vi "EPR DAQ - 1.2.5.13.vi"() -> ()   [LabVIEW 2016]
uses:
  Types/State Control.ctl
  Types/Fitting Model Selection.ctl
  Types/Acquisition Parameters.ctl
  Types/Hardware Parameters.ctl
  Types/Measurement Information.ctl
  Analysis/Dose Calculation and Reporting/Dose Calculation Control.ctl
  Types/Sample Type.ctl
  Types/Spectral Data.ctl
  Types/Save Data Type.ctl
  Types/Global Variables.vi
  DAQ Management/Write Key Bool.vi
  DAQ Management/Get Key U32.vi
panel:
  out "In-Phase SNR":dbl
  in  "Flag Bad Set":bool
  out "Previous Scan range (Gauss)":dbl=25.0 min=0.001 max=55.0 format="%.3f"
  out "Previous Mod. Amp. (Gauss)":dbl=4.0 min=0.0 max=4.0 format="%.4f"
  in  "Acquisition Updates Prescribe":bool
  in  "Single Test Scan":bool
  out "Unacceptable pO2 Estimate":bool
  in  "Exclude Unacceptable pO2":bool
  out "Number of Fit Iterations":i32 caption="Iterations"
  out "SpO2 [%]":dbl format="%#.0f"
  in  "SpO2 Calibration [SpO2/V]":dbl
  in  "Acquire SpO2":bool
  out "pO2 [mmHg]":dbl[](array[numeric]) format="%.1f"
  in  "AFC Field Correction":bool
  in  "Report pO2/Scan":bool
  in  "Open Session Data Folder":bool
  in  "Show Variable Window?":bool
  out "Script Progress":dbl(slide) scale=0.0..1.0
  out "Set Progress":dbl(slide) scale=0.0..1.0
  in  "Sweep Rise [sec]":u32=3
  in  "Prescan delay (ms)":u32=750
  in  "Scan time (sec)":dbl=3.0 format="%.2f"
  in  "Find Peaks":bool
  in  "Continuous Sweeping":bool
  in  "Show Calibration Constants":bool
  in  "Gradients on/off":bool
  in  "Z-Gradient [G/mm]":dbl min=0.0
  in  "Y-Gradient [G/mm]":dbl min=0.0
  in  "X-Gradient [G/mm]":dbl min=0.0
  in  "Spectral Data":T1={"PDT Amp [v]"=0.0, "RIS Amp [v]"=0.0, "B-Field"=[], "All In-Phase Scan Spectra"=[], "Model Select"=enum."OneCompRISTwoPDT", "Fit Each Scan"=FALSE, "PDT Center [g]"=0.0, "In-Phase Average Spectra"=[], "In-Phase Median Spectra"=[], "Out-Phase Median Spectra"=[], "Out-Phase Average Spectra"=[], "Fit Spectra"=[], "Fit No-Baseline Spectra"=[], "All Out-Phase Scan Spectra"=[], "Baseline Offset Correction"=FALSE, "In-Phase Offset [v]"=0.0, "Out-Phase Offset [v]"=0.0, "Ch2 Input\n(Balance)"=[], "Ch3 Input\n(Phase)"=[], "Ch4 Input\n(AFC)"=[], "Fit Pars"=[], "Fit Pars Errors"=[], "Fit Pars Labels"=[], "Raw Scan DAQ Data"=[], "Bad Scans Indicies"=[], "Good In-Phase Scan Spectra"=[], "Good Out-Phase Scan Spectra"=[], "Bad In-Phase Scan Spectra"=[], "Bad Out-Phase Scan Spectra"=[], "Number of bad scans"=0, "Fit History"=[], "PDT Amp. History/Set [v]"=[], "RIS Amp. History/Set [v]"=[], "RIS Amp. History/Scan [v]"=[], "All Shifted B-Fields"=[], "Good Shifted B-Fields"=[], "Ch5 Input\n(SpO2)"=[], "Ch6 Input\n(BPM)"=[], "Global SNR"=0.0, "Fit Error History"=[], "SNR History"=[]} {"Global SNR" min=0.0; "PDT Center [g]" min=0.0; "RIS Amp [v]" min=0.0; "PDT Amp [v]" min=0.0}
  in  "Measurement Information":T3={"Comments"="", "Directory Input"="", "Data file path"=path "C:/Data/EPR Data", "Scripting File"=path "C:/Data/Configuration Script.csv", "Save Data"=FALSE, "Tooth size (d11) [mm]"=0.0, "Tooth size (d12) [mm]"=0.0, "Tooth size (d21) [mm]"=0.0, "Tooth size (d22) [mm]"=0.0, "Dose of Tooth [Gy]"=0.0, "Safe Shutdown?"=FALSE, "Gases Available"=[], "Database Username"="", "Database Password"="", "Database Login URL"="", "Database Upload URL"="", "Database Success URL"="", "Database XML URL"="", "Database Resonator URL"="", "Session Number"=0, "Set #"=0, "Resonator Operator"="", "Session Type"="", "Tooth/Sample ID"="", "Volunteer ID"="", "Computer Operator"="", "Volunteer Type"="", "Site/Tooth Selection (T8,T9)"="", "Resonator"="", "Measurement Site"="", "Non-standard session?"=FALSE, "EPR DAQ Version"="", "Session Path"=path "C:/Data/EPR Data", "Chosen Applied State"="", "Chosen Initial State"="", "Time of Transition"="", "DAQ Mode"=enum."Engineering", "pO2/Scan [mmHg]"=[], "pO2/Set [mmHg]"=[], "Linewidth (HWHM)/Scan [Gauss]"=[], "Linewidth (HWHM)/Set [Gauss]"=[], "pO2 Conversion"="", "Dose Calibration Cluster"={"Dose Response"={"grand_mean"=0.0292016, "slope"=0.0188720543}, "Dose Correction"={"Sex"=1, "a0"=7.719669421, "a1"=-2.746550736, "a2"=-0.186490355, "a3"=0.041922063, "a4"=-0.849147359, "a5"=0.14330063, "a6"=0.019930219, "A_n"=40.0, "H_n"=10.12, "Dose Correction"=FALSE}, "Dose Reporting"={"Reporting is"=TRUE, "sd_threshold [AU]"=0.06, "sd_model [Gy]"=0.66, "dosimetric_threshold [Gy]"=2.0, "Add intrasession errors is"=FALSE, "Prior Radiation?"=FALSE}}, "OxyChip Slope"=0.0, "OxyChip Intercept"=0.0, "QA Mode"=enum."Select QA Mode", "QA Session?"=FALSE, "Sample Type"=enum."Empty Resonator", "Report pO2/Scan"=FALSE, "Skip End Session Save"=FALSE, "Number of sites"=enum."# Probes", "Recipient Name"="", "Sender Name"="", "Recipient Email"="", "Transition State History"=[], "pO2 Report Times"=[], "Temperature [C]"=0.0, "+Error pO2/Scan [mmHg]"=[], "-Error pO2/Scan [mmHg]"=[], "+Error pO2/Set [mmHg]"=[], "-Error pO2/Set [mmHg]"=[], "Oxy Phase Exclusion Tolerance [rad]"=0.0, "Oxy Center Exclusion Tolerance [%]"=0.0, "Oxy Exclude Unacceptable"=FALSE, "Oxy Unacceptable Estimate Flags"=[], "Save Session PPT"=FALSE, "Flagged Bad Sets"=[]} {"Oxy Center Exclusion Tolerance [%]" format="%#_9g"; "Oxy Phase Exclusion Tolerance [rad]" format="%#_9g"; "Temperature [C]" format="%#_9g"; "OxyChip Intercept" format="%#_9g"; "OxyChip Slope" format="%#_9g"; "Dose Calibration Cluster"."Dose Reporting"."dosimetric_threshold [Gy]" format="%#_9g"; "Dose Calibration Cluster"."Dose Reporting"."sd_model [Gy]" format="%#_9g"; "Dose Calibration Cluster"."Dose Reporting"."sd_threshold [AU]" format="%#_9g"; "Dose Calibration Cluster"."Dose Correction"."H_n" format="%#_9g"; "Dose Calibration Cluster"."Dose Correction"."A_n" format="%#_9g"; "Dose Calibration Cluster"."Dose Correction"."a6" format="%#.9g"; "Dose Calibration Cluster"."Dose Correction"."a5" format="%#.9g"; "Dose Calibration Cluster"."Dose Correction"."a4" format="%#.9g"; "Dose Calibration Cluster"."Dose Correction"."a3" format="%#.9g"; "Dose Calibration Cluster"."Dose Correction"."a2" format="%#.9g"; "Dose Calibration Cluster"."Dose Correction"."a1" format="%#.9g"; "Dose Calibration Cluster"."Dose Correction"."a0" format="%#.9g"; "Dose Calibration Cluster"."Dose Correction"."Sex" items=["Male"=1, "Female"=0]; "Dose Calibration Cluster"."Dose Response"."slope" format="%#_9g"; "Dose Calibration Cluster"."Dose Response"."grand_mean" format="%#_9g"}
  in  "Hardware Parameters":T6={"Scan Calibration [G/V]"=0.0, "Modulation Calibration [G/V]"=0.0, "Modulation Phase [deg]"=0.0, "Modulation Frequency [Hz]"=0.0, "Attenuation [dB]"=0, "Input Channel Count"=0, "Time constant"=7, "Sensitivity"=17, "Frequency Output Voltage [V]"=0.0, "Phase Output Voltage [V]"=0.0, "Lock-in Offset Compensation"=FALSE, "RF [GHz]"=0.0, "Q Start"=0.0, "Q End"=0.0, "Balance"=0.0, "Phase Error"=0.0, "AFC Error"=0.0, "AFC"=FALSE, "Magnet Rotation"=FALSE, "Balance Scaling Factor"=1.0, "Phase Error Scaling Factor"=1.0, "AFC Error Scaling Factor"=1.0, "Frequency Counter ID"="", "Sweep Waveform"=enum."Sawtooth", "Q-Factor Scale"=0.0, " Q-Data Scale"=0.0, " Q-Data Offset"=0.0, "Magnet Rotation Slope"=0.0, "Magnet Rotation Offset"=0.0, "Phase Sweep Resolution"=0.0, "Hardware Version Number"="", "Spectrometer ID Number"=0, "Spectrometer Name"="", "Lock in Saturation"=0.0, "Balance Threshold"=0.0, "Phase Error Threshold"=0.0, "AFC Error Threshold"=0.0, "Linear Actuator Length"=0.0, "Lock-in OK?"=FALSE, "Ignore Lock-in Comm. Failure"=FALSE, "Gradient Addresses"=[], "Gradient Calibrations [G/A*mm]"=[], "Gradient Power Supplies"=[], "Lock-in Address"="", "Magnet Type"=enum."RRI", "Camera Names"=[], "Sweep Limit [Gauss]"=0.0, "Modulation Limit [Gauss]"=0.0, "Balance Threshold Exceeded?"=FALSE, "Phase Threshold Exceeded?"=FALSE, "AFC Threshold Exceeded?"=FALSE, "Consecutive Re-tune attempts"=0, "Reverse Sweep Slope [sec]"=0.0, "Reverse Sweep Offset [G]"=0.0, "AFC Field Correction [V/MHz]"=0.0, "Active Gradients (X Y Z)"=[], "SpO2 Calibration [SpO2/V]"=1.0, "Heart Rate Calibration [BPM/V]"=1.0, "Thermocouple Channel"=""} {"Sensitivity" items=["", "2 nV", "5 nV", "10 nV", "20 nV", "50 nV", "100 nV", "200 nV", "500 nV", "1 uV", "2 uV", "5 uV", "10 uV", "20 uV", "50 uV", "100 uV", "200 uV", "500 uV", "1 mV", "2 mV", "5 mV", "10 mV", "20 mV", "50 mV", "100 mV", "200 mV", "500 mV", "1 V"]; "Time constant" items=["10 us", "20 us", "40 us", "80 us", "160 us", "320 us", "640 us", "5 ms", "10 ms", "20 ms", "50 ms", "100 ms", "200 ms", "500 ms", "1 s", "2 s", "5 s", "10 s", "20 s", "50 s", "100 s", "200 s", "500 s", "1 ks", "2 ks", "5 ks", "10 ks", "20 ks", "50 ks", "100 ks"]}
  in  "Acquisition Parameters":T7={"Magnet Angle [deg]"=0.0, "Magnet Angles [deg]"=[], "DeltaVpp [v]"=0.0, "SEM [v]"=0.0, "DeltaVpp Thresh [v]"=0.0, "SEM Thresh [v]"=0.0, "Adaptive Processing"=FALSE, "Acquire Q"=FALSE, "Acquire Photos"=FALSE, "Adaptive Tuning"=FALSE, "Automated Matching"=FALSE, "X-Gradient [G/mm]"=0.0, "Y-Gradient [G/mm]"=0.0, "Z-Gradient [G/mm]"=0.0, "Central Field [G]"=0.0, "Scan Width [G]"=0.0, "Mod. Amp. [G]"=0.0, "Scan Time [s]"=0.0, "Pre-Scan Delay [ms]"=0, "Measurement Timeout [s]"=0.0, "Electromagnet Main Field [G]"=0.0, "Locked Central Field [G]"=0.0, "Scans Excluded"=0, "Scans Completed"=0, "No. Scans/Set"=0, "No. Scans for SNR"=0, "Field Locked Frequency [GHz]"=0.0, "Auto Set-based Field Center"=FALSE, "Prompt for oxy acquisition updates"=FALSE, "Oxy QA Scan?"=FALSE, "Exclude Bad Data"=FALSE, "Optimizing RF Power"=FALSE, "Gradients on/off"=FALSE, "Running Script"=TRUE, "Opto-Coupler Current [A]"=0.0, "Continuous Sweeping"=FALSE, "Sweep Rise Time [sec]"=0, "Reverse Sweep Central Field [G]"=0.0, "Forward Sweep Central Field [G]"=0.0, "Sweep Calibrated"=FALSE, "Modulation Calibrated"=FALSE, "First CheckCal Scan?"=FALSE, "AFC Field Correction"=FALSE, "OxyQAInit Scan Width [G]"=0.0, "OxyQAInit Mod. Amp. [G]"=0.0, "Scans Completed/Session"=0, "Acquire SpO2"=FALSE, "Acquire Temperature"=FALSE, "Over Mod"=FALSE} {"OxyQAInit Mod. Amp. [G]" min=0.0; "OxyQAInit Scan Width [G]" min=0.0; "Mod. Amp. [G]" min=0.0; "Scan Width [G]" min=0.0; "Measurement Timeout [s]" min=0.0; "Scan Time [s]" min=0.0; "Z-Gradient [G/mm]" min=0.0; "Y-Gradient [G/mm]" min=0.0; "X-Gradient [G/mm]" min=0.0; "SEM Thresh [v]" min=0.0; "DeltaVpp Thresh [v]" min=0.0; "SEM [v]" min=0.0}
  in  "Update Scan/Mod from Cursors":bool
  in  "Model Select":T2=enum."OneCompRISTwoPDT"
  in  "Refit Spectra":bool
  in  "Fit Each Scan":bool=TRUE
  in  "DAQ Mode":enum16{"Engineering", "Dosimetry", "Oximetry"}(ring)
  out "Out-Phase Noise":dbl
  out "In-Phase Noise":dbl
  out "Fit Pars and Labels":cluster{"Pars Labels":string[], "pars":dbl[]}
  in  "Timer on/off":bool
  out "Time Remaining":dbl caption="Elapsed Time (s)" format="%<%H:%M:%S>t"
  in  "Timer Value":dbl=600.0 caption="Time Target (s)" min=1.0 format="%<%H:%M:%S>t"
  in  "Optimize RF Power":bool
  in  "Apply & Lock Center Field":bool
  in  "Update Center Field":bool
  in  "Collect QA Scan":bool
  out "Linewidth (HWHM)/Set [Gauss]":dbl[][](graph)
  out "pO2/Set [mmHg]":dbl[][](graph)
  out "Linewidth (HWHM) [Gauss]":dbl[][](graph)
  out "pO2/Scan [mmHg]":dbl[][](graph)
  in  "Prompt for acquisition updates":bool
  in  "Electromagnet Main Field (Gauss)":dbl=-2.1630895005314263 format="%.3f"
  in  "Lock Field":bool
  in  "Auto Set-based Field Center":bool
  in  "Balance Scale Factor":dbl
  in  "Phase Scale Factor":dbl
  in  "AFC Scale Factor":dbl
  out "Last Error":errorcluster
  in  "Ignore Errors":bool
  in  "Mark Time of Transition":bool
  in  "Applied State":i32(ring) items=["Air", "100%-O2", "Compression", "None", "custom1", "custom2"]
  in  "Initial State":i32(ring) items=["Air", "100%-O2", "Compression", "None", "custom1", "custom2"]
  out "State Control History":T8[](array[typedef])
  in  "Error Counter":i32
  in  "Input Channel Count":i32=4
  out "Status of EPR DAQ":T8
  in  "Show All":bool
  in  "Sweep Waveform":T9(ring)=enum."Sawtooth"
  out "Producer Loop":i32
  out "Consumer Loop":i32
  in  "Get Q":bool
  in  "Reset Match":bool
  in  "AdaptiveTune_Enable":bool=TRUE
  in  "Attenuation/dB":u16 max=31 step=1
  in  "Set Match":bool
  in  "Set Freq":bool
  in  "Zero All Voltage":bool
  out "Frequency Voltage":dbl
  out "Phase Voltage":dbl
  in  "Set Phase":bool
  in  "AFC Control":bool=TRUE
  in  "Adaptive Evaluation":bool=TRUE
  out "DELTAVpp_THRESH":dbl
  out "DELTAVpp":dbl
  out "SEM_THRESH":dbl
  out "SEM":dbl
  in  "Magnet Angle (deg)":dbl min=-360.0 max=360.0 step=0.001 format="%.2f"
  out "Balance/Phase/AFC Meter":cluster{dbl, dbl, dbl}(knob)={0.0, 0.3938071037321068, -0.43103227358131235} caption="Balance          Phase              AFC" scale=-10.0..10.0 scale format="%#_3g"
  in  "Magnet Rotation":bool=TRUE
  out "Scripting Sets":i32
  out "Session Number":i32=3344
  out "Out Phase Offset":dbl format="%0.4f"
  out "In Phase Offset":dbl format="%0.4f"
  in  "Baseline Correction":bool=TRUE
  out "Q Start":dbl
  in  "Start Script":bool
  in  "End Session?":bool
  out "Sets Completed":u32 min=1 max=1000 step=1
  out "Volunteer ID":string
  out "Sample ID":string
  out "Session Type":string
  in  "Directory Input":string
  in  "Scripting File":path=path "C:/Data/EPR DAQ Scripting File.csv"
  in  "Data file path":path=path "C:/Data/EPR Data"
  in  "Manual Tuning":bool
  in  "Mode":bool
  out "Lock-In OK?":bool=TRUE
  in  "Calibrate":bool
  in  "Auto-Tune":bool
  in  "Stop Scan":bool
  in  "Measure Noise":bool
  in  "New Session":bool
  out "Operators":string
  in  "Comments":string
  out "PDT Amp p-p":dbl format="%#_4g"
  in  "Visible-Center PDT":bool
  out "Tooth Amp P-P":dbl format="%#_4g"
  in  "Visible-CFitNoBaseline":bool=TRUE
  in  "Visible-CFit":bool
  in  "Visible-Median Out Phase":bool=TRUE
  in  "Visible-Median In Phase":bool
  in  "Offset comp.?":bool
  in  "Sensitivity":u16(ring)=17 items=["", "2 nV", "5 nV", "10 nV", "20 nV", "50 nV", "100 nV", "200 nV", "500 nV", "1 uV", "2 uV", "5 uV", "10 uV", "20 uV", "50 uV", "100 uV", "200 uV", "500 uV", "1 mV", "2 mV", "5 mV", "10 mV", "20 mV", "50 mV", "100 mV", "200 mV", "500 mV", "1 V"]
  in  "Mod. Gauss/Vrms":dbl=6.7 format="%.4f"
  in  "Scan Gauss/V":dbl=3.93 format="%.4f"
  in  "Visible-Out Phase":bool=TRUE
  in  "Visible-In Phase":bool
  out "of":u32=5
  out "Scan no.":u32=2
  in  "No. Scans/Set":u32=5 min=1 step=1
  out "LW,\nAmp":dbl[](array[numeric]) format="%.3f"
  in  "Save data":bool=TRUE
  in  "Mod. Amp. (Gauss)":dbl=4.0 min=0.0 max=4.0 format="%.4f"
  in  "Phase (deg)":dbl=-12.9 min=-360.0 max=360.0 step=0.001 format="%.2f"
  in  "Time constant":u16(ring)=7 items=["10 us", "20 us", "40 us", "80 us", "160 us", "320 us", "640 us", "5 ms", "10 ms", "20 ms", "50 ms", "100 ms", "200 ms", "500 ms", "1 s", "2 s", "5 s", "10 s", "20 s", "50 s", "100 s", "200 s", "500 s", "1 ks", "2 ks", "5 ks", "10 ks", "20 ks", "50 ks", "100 ks"]
  in  "Frequency (Hz)":dbl=20800.0 min=10000.0 max=30000.0 step=1.0
  out "RF (GHz)":dbl=1.1465201999999999 format="%.9f"
  out "Spectra Graph":cluster{dbl[], "Value":dbl[]}[](graph)=[{array[1024 elements], "Value"=array[1024 elements]}, {array[1024 elements], "Value"=array[1024 elements]}, {array[1024 elements], "Value"=array[1024 elements]}, {array[1024 elements], "Value"=array[1024 elements]}, {array[1024 elements], "Value"=array[8194 elements]}, {array[1024 elements], "Value"=array[8194 elements]}, {[5.5, 5.5], "Value"=[4.2, 1.8]}]
  in  "Scan?":bool caption="Scan"
  in  "Central field (Gauss)":dbl format="%.3f"
  in  "Quit":bool
  in  "Scan range (Gauss)":dbl=25.0 min=0.001 max=55.0 format="%.3f"
  # "Fitting Parameters"
  # "Data Saving"
  # "Tuning Controls"
  # "Sweep Field"
  # "Lock-In Amplifier"
  # "Modulation Field"
  # "Offset Correction"
  # "Resonator"
  # "Gradients"
  # "Adaptive Processing"
  # "Fitting"
  # "Noise"
  # "Timing"
  # "Session Information"
  # "Oximetric Data and Information"
  # "Email"
  # "Tooth Information"
  # "Database"
  # "Bridge I/O"
  # "Magnet Rotation"
  # "Field Calibration"
  # "Lock In Amplifier"
  # "Spectrometer Information"
  # "DAQ Settings"
  # "Gradient Coils and Field"
  # "X"
  # "Y"
  # "Z"
  # "Q-Measurements"
  # "Gradients"
  # "Field"
  # "Scans and Sets"
  # "Timing"
  # "Adaptive Dosimetric \nData Processing"
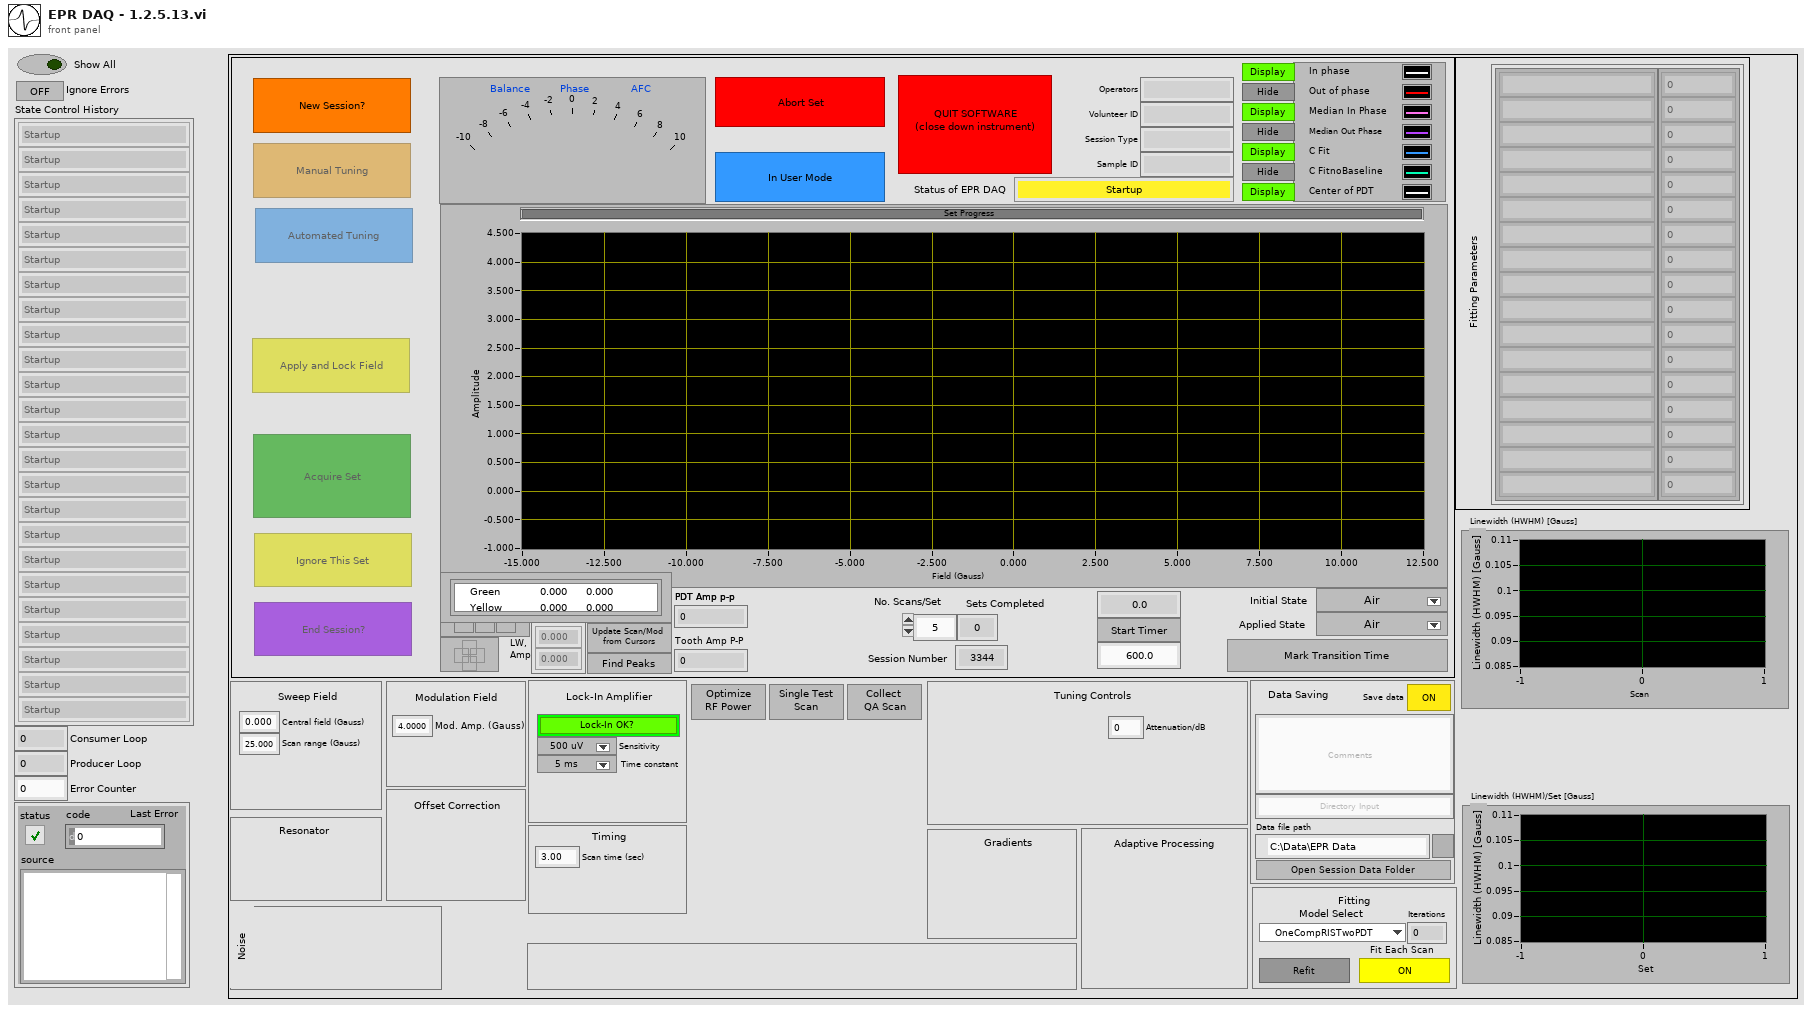
[diagram p1: front panel]
types:
  T1 = typedef "Spectral Data.ctl" = cluster{"PDT Amp [v]":dbl, "RIS Amp [v]":dbl, "B-Field":dbl[], "All In-Phase Scan Spectra":dbl[][], "Model Select":T2, "Fit Each Scan":bool, "PDT Center [g]":dbl, "In-Phase Average Spectra":dbl[], "In-Phase Median Spectra":dbl[], "Out-Phase Median Spectra":dbl[], "Out-Phase Average Spectra":dbl[], "Fit Spectra":dbl[], "Fit No-Baseline Spectra":dbl[], "All Out-Phase Scan Spectra":dbl[][], "Baseline Offset Correction":bool, "In-Phase Offset [v]":dbl, "Out-Phase Offset [v]":dbl, "Ch2 Input\n(Balance)":dbl[], "Ch3 Input\n(Phase)":dbl[], "Ch4 Input\n(AFC)":dbl[], "Fit Pars":dbl[], "Fit Pars Errors":dbl[], "Fit Pars Labels":string[], "Raw Scan DAQ Data":dbl[][], "Bad Scans Indicies":i32[], "Good In-Phase Scan Spectra":dbl[][], "Good Out-Phase Scan Spectra":dbl[][], "Bad In-Phase Scan Spectra":dbl[][], "Bad Out-Phase Scan Spectra":dbl[][], "Number of bad scans":i32, "Fit History":dbl[][], "PDT Amp. History/Set [v]":dbl[], "RIS Amp. History/Set [v]":dbl[], "RIS Amp. History/Scan [v]":dbl[], "All Shifted B-Fields":dbl[][], "Good Shifted B-Fields":dbl[][], "Ch5 Input\n(SpO2)":dbl[], "Ch6 Input\n(BPM)":dbl[], "Global SNR":dbl, "Fit Error History":dbl[][], "SNR History":dbl[]}
  T2 = typedef "Fitting Model Selection.ctl" = enum16{"OneCompRIS", "OneCompRISTwoPDT", "OneCompRISRev", "OneCompRISTwoPDTRev", "LiPc", "TwoLiPc", "ThreeLiPc", "FourLiPc", "PDTCalibration", "CE_Ink", "Printex", "MelaninTwoPDT"}
  T3 = typedef "Measurement Information.ctl" = cluster{"Comments":string, "Directory Input":string, "Data file path":path, "Scripting File":path, "Save Data":bool, "Tooth size (d11) [mm]":dbl, "Tooth size (d12) [mm]":dbl, "Tooth size (d21) [mm]":dbl, "Tooth size (d22) [mm]":dbl, "Dose of Tooth [Gy]":dbl, "Safe Shutdown?":bool, "Gases Available":string[], "Database Username":string, "Database Password":string, "Database Login URL":string, "Database Upload URL":string, "Database Success URL":string, "Database XML URL":string, "Database Resonator URL":string, "Session Number":i32, "Set #":u32, "Resonator Operator":string, "Session Type":string, "Tooth/Sample ID":string, "Volunteer ID":string, "Computer Operator":string, "Volunteer Type":string, "Site/Tooth Selection (T8,T9)":string, "Resonator":string, "Measurement Site":string, "Non-standard session?":bool, "EPR DAQ Version":string, "Session Path":path, "Chosen Applied State":string, "Chosen Initial State":string, "Time of Transition":string, "DAQ Mode":enum16{"Engineering", "Dosimetry", "Oximetry"}, "pO2/Scan [mmHg]":dbl[][], "pO2/Set [mmHg]":dbl[][], "Linewidth (HWHM)/Scan [Gauss]":dbl[][], "Linewidth (HWHM)/Set [Gauss]":dbl[][], "pO2 Conversion":string, "Dose Calibration Cluster":T4, "OxyChip Slope":dbl, "OxyChip Intercept":dbl, "QA Mode":enum16{"Select QA Mode", "QA-Start/End", "QA-Mid", "QA-Weekly", "QA-Eng", "Check Calibration"}, "QA Session?":bool, "Sample Type":T5, "Report pO2/Scan":bool, "Skip End Session Save":bool, "Number of sites":enum16{"# Probes", "1", "2", "3", "4"}, "Recipient Name":string, "Sender Name":string, "Recipient Email":string, "Transition State History":string[], "pO2 Report Times":string[], "Temperature [C]":dbl, "+Error pO2/Scan [mmHg]":dbl[][], "-Error pO2/Scan [mmHg]":dbl[][], "+Error pO2/Set [mmHg]":dbl[][], "-Error pO2/Set [mmHg]":dbl[][], "Oxy Phase Exclusion Tolerance [rad]":dbl, "Oxy Center Exclusion Tolerance [%]":dbl, "Oxy Exclude Unacceptable":bool, "Oxy Unacceptable Estimate Flags":bool[], "Save Session PPT":bool, "Flagged Bad Sets":u32[]}
  T4 = typedef "Dose Calculation Control.ctl" = cluster{"Dose Response":cluster{"grand_mean":dbl, "slope":dbl}, "Dose Correction":cluster{"Sex":u16, "a0":dbl, "a1":dbl, "a2":dbl, "a3":dbl, "a4":dbl, "a5":dbl, "a6":dbl, "A_n":dbl, "H_n":dbl, "Dose Correction":bool}, "Dose Reporting":cluster{"Reporting is":bool, "sd_threshold [AU]":dbl, "sd_model [Gy]":dbl, "dosimetric_threshold [Gy]":dbl, "Add intrasession errors is":bool, "Prior Radiation?":bool}}
  T5 = typedef "Sample Type.ctl" = enum16{"Empty Resonator", "IRS", "BallZero", "Irradiated Tooth", "Non-irradiated Tooth", "OxyChip", "LiPc", "PDT", "India Ink"}
  T6 = typedef "Hardware Parameters.ctl" = cluster{"Scan Calibration [G/V]":dbl, "Modulation Calibration [G/V]":dbl, "Modulation Phase [deg]":dbl, "Modulation Frequency [Hz]":dbl, "Attenuation [dB]":u16, "Input Channel Count":i32, "Time constant":u16, "Sensitivity":u16, "Frequency Output Voltage [V]":dbl, "Phase Output Voltage [V]":dbl, "Lock-in Offset Compensation":bool, "RF [GHz]":dbl, "Q Start":dbl, "Q End":dbl, "Balance":dbl, "Phase Error":dbl, "AFC Error":dbl, "AFC":bool, "Magnet Rotation":bool, "Balance Scaling Factor":dbl, "Phase Error Scaling Factor":dbl, "AFC Error Scaling Factor":dbl, "Frequency Counter ID":string, "Sweep Waveform":enum16{"Sine Wave", "Square Wave", "Sawtooth", "Triangle Wave"}, "Q-Factor Scale":dbl, " Q-Data Scale":dbl, " Q-Data Offset":dbl, "Magnet Rotation Slope":dbl, "Magnet Rotation Offset":dbl, "Phase Sweep Resolution":dbl, "Hardware Version Number":string, "Spectrometer ID Number":i32, "Spectrometer Name":string, "Lock in Saturation":dbl, "Balance Threshold":dbl, "Phase Error Threshold":dbl, "AFC Error Threshold":dbl, "Linear Actuator Length":dbl, "Lock-in OK?":bool, "Ignore Lock-in Comm. Failure":bool, "Gradient Addresses":string[], "Gradient Calibrations [G/A*mm]":dbl[], "Gradient Power Supplies":string[], "Lock-in Address":refnum<visa-resource-name>, "Magnet Type":enum16{"RRI", "BARDA", "Whole Body Permanent", "RRI Electromagnet"}, "Camera Names":string[], "Sweep Limit [Gauss]":dbl, "Modulation Limit [Gauss]":dbl, "Balance Threshold Exceeded?":bool, "Phase Threshold Exceeded?":bool, "AFC Threshold Exceeded?":bool, "Consecutive Re-tune attempts":i32, "Reverse Sweep Slope [sec]":dbl, "Reverse Sweep Offset [G]":dbl, "AFC Field Correction [V/MHz]":dbl, "Active Gradients (X Y Z)":bool[], "SpO2 Calibration [SpO2/V]":dbl, "Heart Rate Calibration [BPM/V]":dbl, "Thermocouple Channel":tag}
  T7 = typedef "Acquisition Parameters.ctl" = cluster{"Magnet Angle [deg]":dbl, "Magnet Angles [deg]":dbl[], "DeltaVpp [v]":dbl, "SEM [v]":dbl, "DeltaVpp Thresh [v]":dbl, "SEM Thresh [v]":dbl, "Adaptive Processing":bool, "Acquire Q":bool, "Acquire Photos":bool, "Adaptive Tuning":bool, "Automated Matching":bool, "X-Gradient [G/mm]":dbl, "Y-Gradient [G/mm]":dbl, "Z-Gradient [G/mm]":dbl, "Central Field [G]":dbl, "Scan Width [G]":dbl, "Mod. Amp. [G]":dbl, "Scan Time [s]":dbl, "Pre-Scan Delay [ms]":u32, "Measurement Timeout [s]":dbl, "Electromagnet Main Field [G]":dbl, "Locked Central Field [G]":dbl, "Scans Excluded":u32, "Scans Completed":u32, "No. Scans/Set":u32, "No. Scans for SNR":u32, "Field Locked Frequency [GHz]":dbl, "Auto Set-based Field Center":bool, "Prompt for oxy acquisition updates":bool, "Oxy QA Scan?":bool, "Exclude Bad Data":bool, "Optimizing RF Power":bool, "Gradients on/off":bool, "Running Script":bool, "Opto-Coupler Current [A]":dbl, "Continuous Sweeping":bool, "Sweep Rise Time [sec]":u32, "Reverse Sweep Central Field [G]":dbl, "Forward Sweep Central Field [G]":dbl, "Sweep Calibrated":bool, "Modulation Calibrated":bool, "First CheckCal Scan?":bool, "AFC Field Correction":bool, "OxyQAInit Scan Width [G]":dbl, "OxyQAInit Mod. Amp. [G]":dbl, "Scans Completed/Session":u32, "Acquire SpO2":bool, "Acquire Temperature":bool, "Over Mod":bool}
  T8 = typedef "State Control.ctl" = enum16{"Startup", "Read Config File", "Initilize Optional Hardware", "Idle", "New Session", "Read GUI Pars", "Configure Hardware", "Initialize Set", "Pre-Scan", "Scan", "Post-Scan", "Exit Set", "Automated Tuning", "Manual Tuning", "Check Calibration", "Optimize RF Power", "Test Scan", "Set Oxy QA-Scan Pars", "Find Peaks", "Update from Cursors", "Flag Bad Set", "Mark transition time", "Measure Q", "Measure Noise", "Rotate Magnet", "Lock Field", "Engineering Tuning", "Zero Voltages", "Update Center Field", "Refit Data", "Open Session Data Folder", "AfterSave", "Undo Auto Update Pars", "Read from Script", "End Session", "Quit Software", "Error"}
  T9 = enum16{"Sine Wave", "Square Wave", "Sawtooth", "Triangle Wave"}
  T10 = enum8{"Enabled", "Disabled", "Disabled and Grayed Out"}
  T11 = enum16{"RRI", "BARDA", "Whole Body Permanent", "RRI Electromagnet"}
  T12 = enum16{"Main and Gradients", "Main Field", "Gradients"}
  T13 = typedef "Save Data Type.ctl" = enum16{"Good Scan", "Bad Scan", "Appended Scans", "Median", "Filename"}
  T14 = enum16{"Select QA Mode", "QA-Start/End", "QA-Mid", "QA-Weekly", "QA-Eng", "Check Calibration"}
  T15 = typedef "LVCursorListTypeDef.ctl" = cluster{"Name":string, "Color":u32, "Style":u8, "Point Style":u8, "Name Visible":bool, "Allow Drag":bool, "Cursor Mode":u32, "Plot":i32, "Index":i32, "Position":cluster{"X":dbl, "Y":dbl}, "X Scale":u32, "Y Scale":u32, "Watch Plots":i32[], "Watch All Plots":bool, "Plot Area":i32, "Label Offset":cluster{"X":dbl, "Y":dbl}}[]
  T16 = cluster{"Name":string, "Color":u32, "Style":u8, "Point Style":u8, "Name Visible":bool, "Allow Drag":bool, "Cursor Mode":u32, "Plot":i32, "Index":i32, "Position":cluster{"X":dbl, "Y":dbl}, "X Scale":u32, "Y Scale":u32, "Watch Plots":i32[], "Watch All Plots":bool, "Plot Area":i32, "Label Offset":cluster{"X":dbl, "Y":dbl}}
  T17 = cluster{"Name":string, "Color":u32, "Style":u8, "Point Style":u8, "Name Visible":bool, "Allow Drag":bool, "Cursor Mode":u32, "Plot":i32, "Index":i32, "Position":cluster{"X":dbl, "Y":dbl}, "X Scale":u32, "Y Scale":u32, "Watch Plots":i32[], "Watch All Plots":bool, "Plot Area":i32, "Label Offset":cluster{"X":dbl, "Y":dbl}}[]
  T18 = cluster{"B-Field":dbl[], "Graphing Array":dbl[]}[]
  T19 = typedef "LVPointTypeDef.ctl" = cluster{"Horizontal":i16, "Vertical":i16}
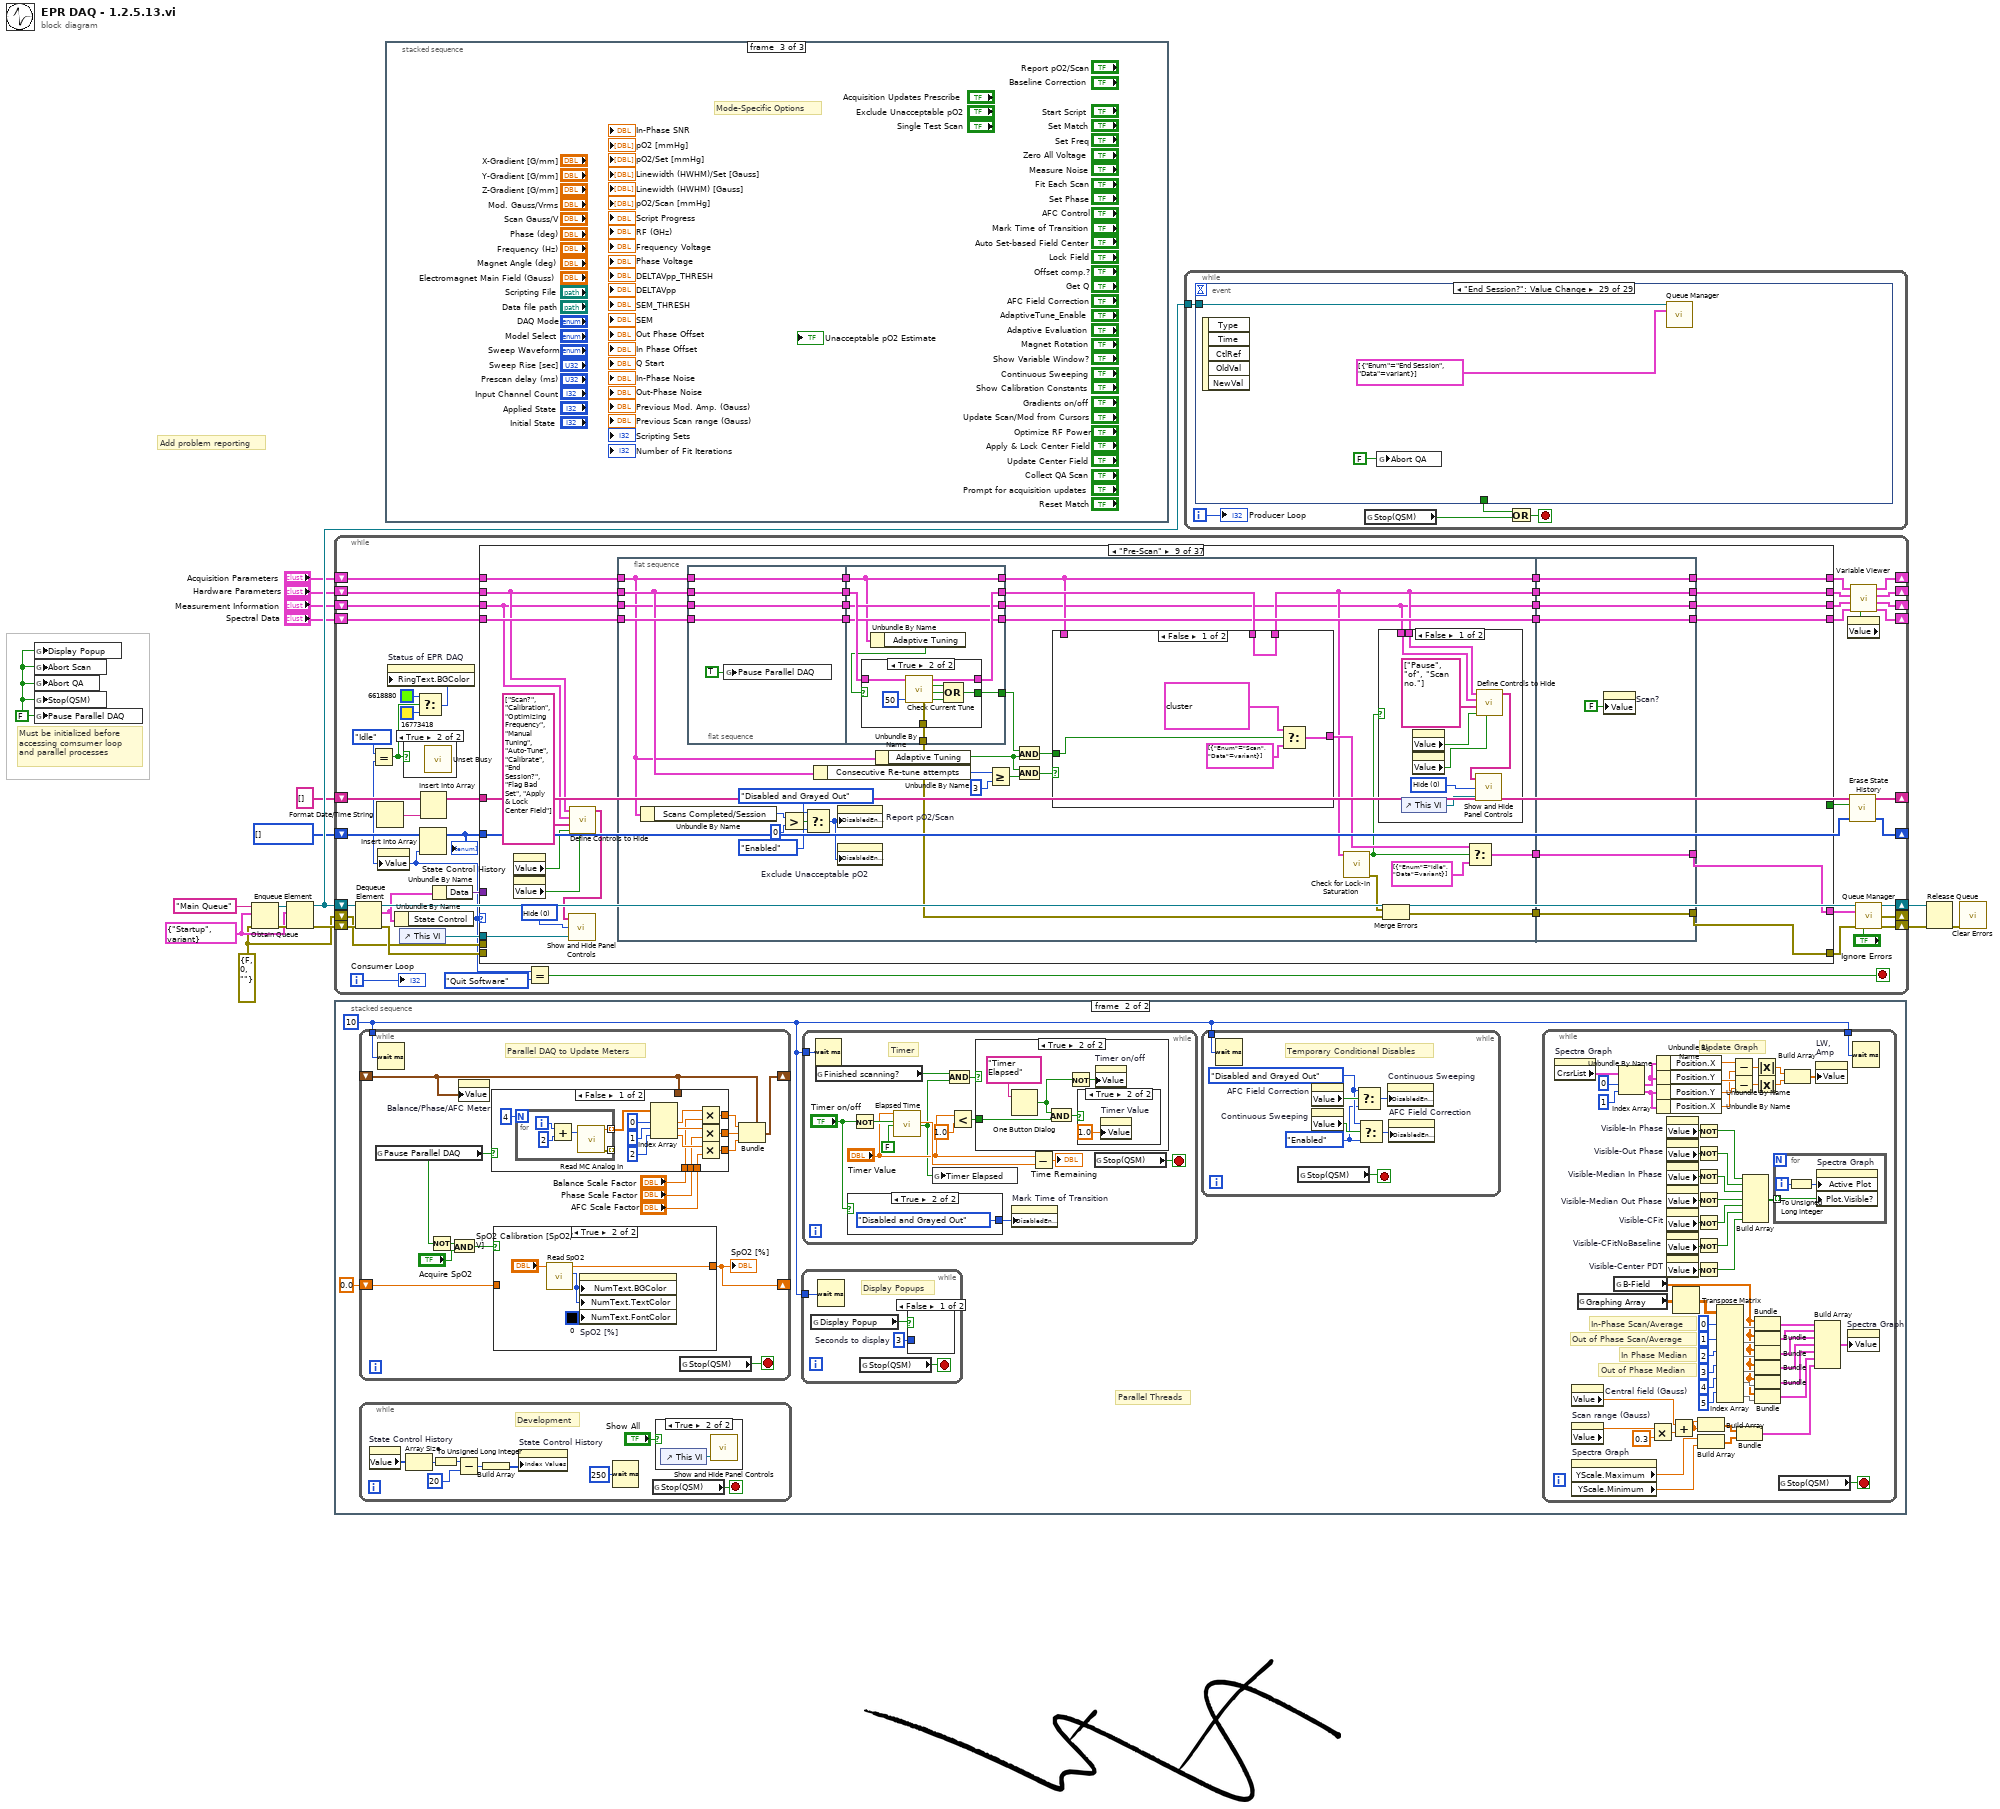
[diagram p0: block diagram]
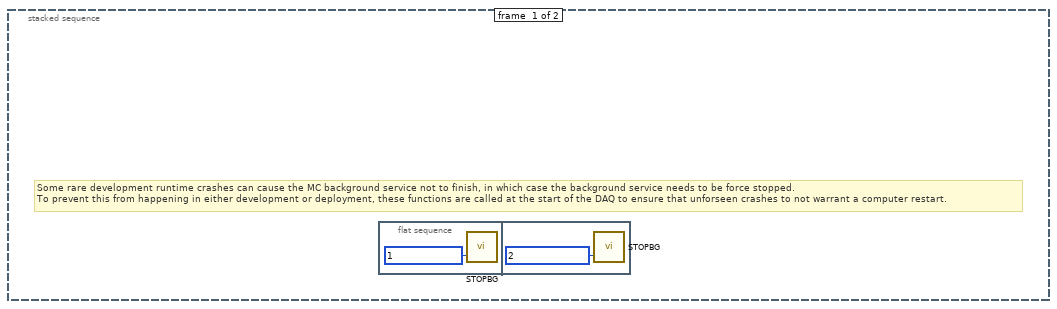
[diagram p2: hidden frame]
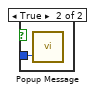
[diagram p3: hidden frame]
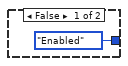
[diagram p4: hidden frame]
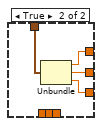
[diagram p9: hidden frame]
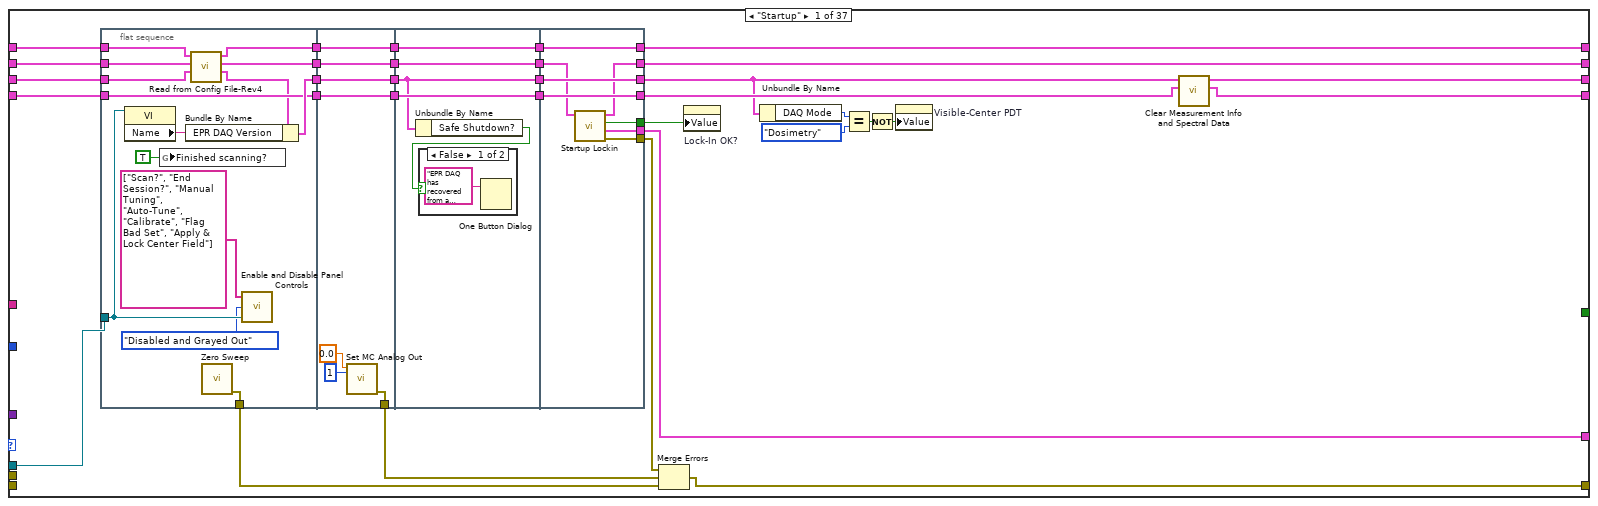
[diagram p10: hidden frame]
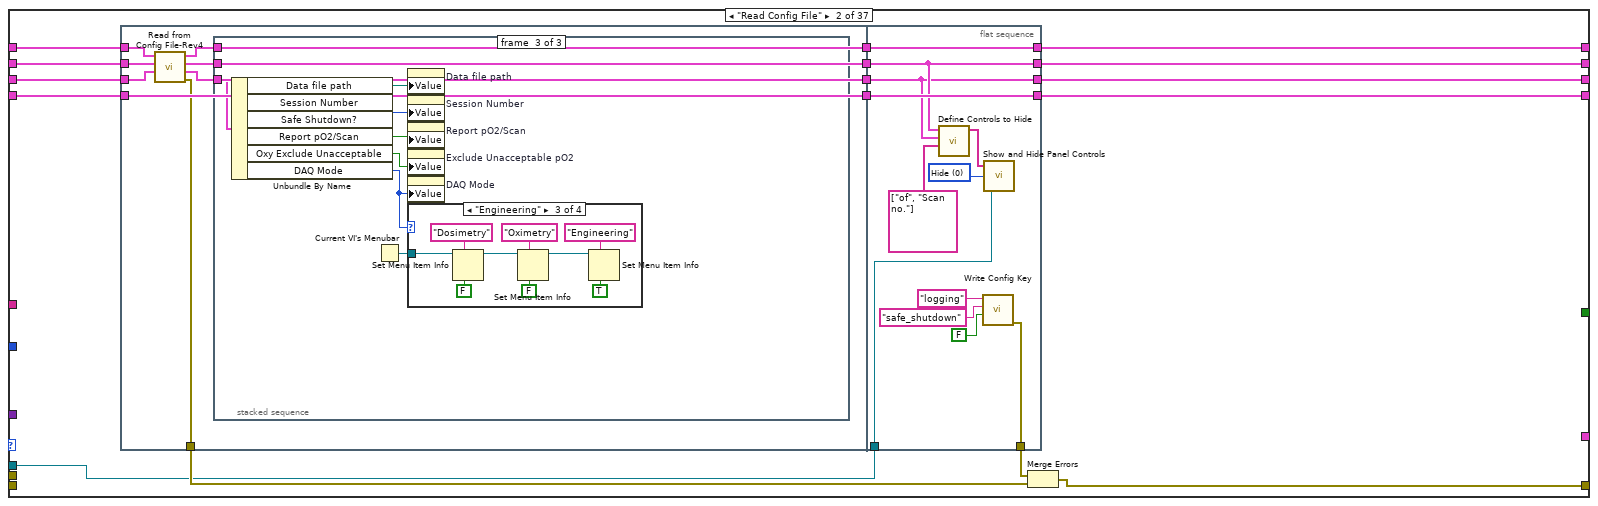
[diagram p12: hidden frame]
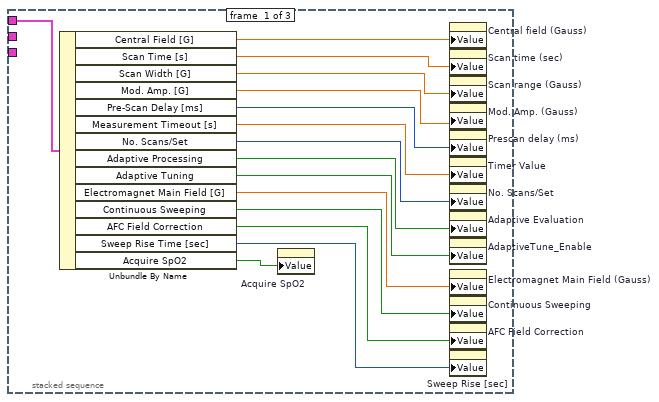
[diagram p13: hidden frame]
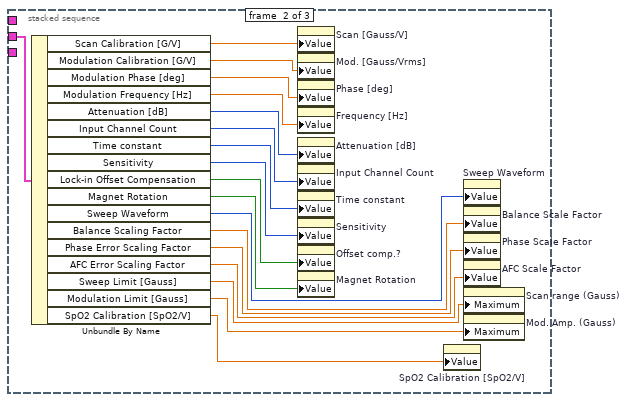
[diagram p14: hidden frame]
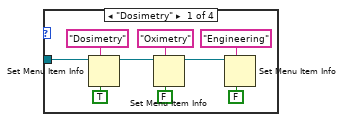
[diagram p15: hidden frame]
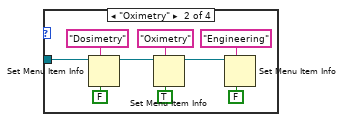
[diagram p16: hidden frame]
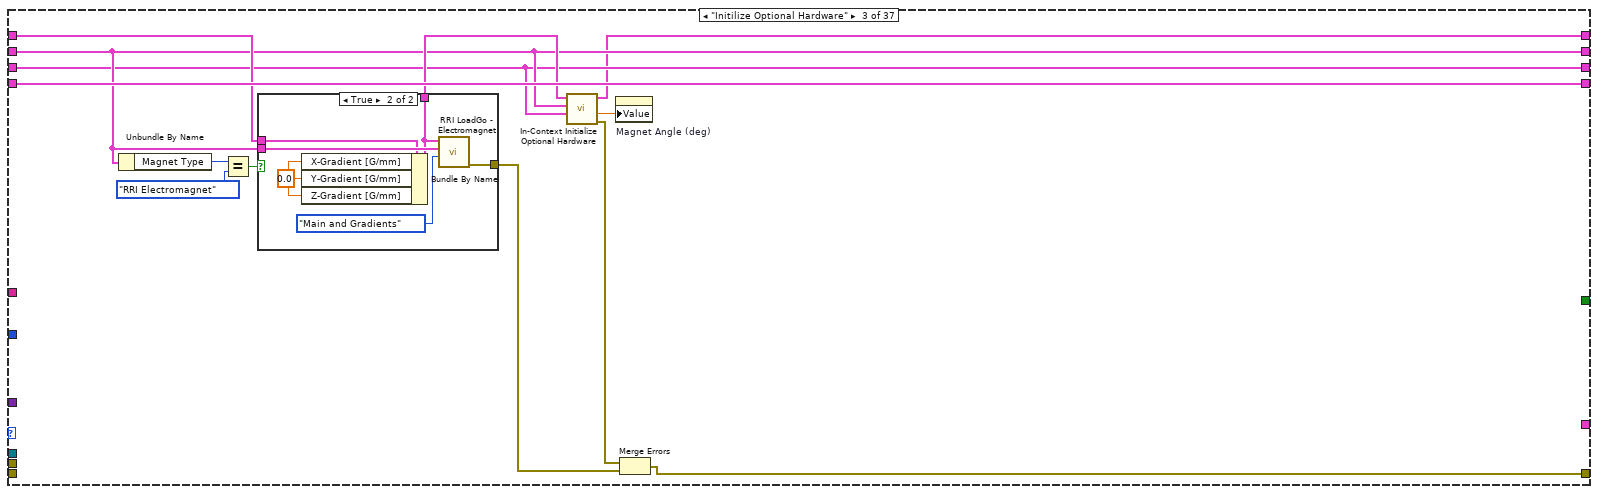
[diagram p18: hidden frame]
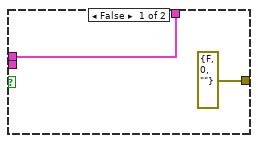
[diagram p19: hidden frame]
diagram:
  w1 = FALSE ("Stop(QSM)")
  w8 = T8[] [] items=["Startup", "Read Config File", "Initilize Optional Hardware", "Idle", "New Session", "Read GUI Pars", "Configure Hardware", "Initialize Set", "Pre-Scan", "Scan", "Post-Scan", "Exit Set", "Automated Tuning", "Manual Tuning", "Check Calibration", "Optimize RF Power", "Test Scan", "Set Oxy QA-Scan Pars", "Find Peaks", "Update from Cursors", "Flag Bad Set", "Mark transition time", "Measure Q", "Measure Noise", "Rotate Magnet", "Lock Field", "Engineering Tuning", "Zero Voltages", "Update Center Field", "Refit Data", "Open Session Data Folder", "AfterSave", "Undo Auto Update Pars", "Read from Script", "End Session", "Quit Software", "Error"]
  w6 = errorcluster {"status"=FALSE, "code"=0, "source"=""} ("error out")
  w14 = cluster{"State Control":T8, "Data":variant} {"State Control"=enum."Startup", "Data"=variant} ("element")
  # "Add problem reporting"
  # "Must be initialized before accessing comsumer loop and parallel processes"
  n1 = global write "Global Variables.vi" "Display Popup"(w1) -> ()
  n2 = global write "Global Variables.vi" "Abort Scan"(w1) -> ()
  n3 = global write "Global Variables.vi" "Abort QA"(w1) -> ()
  n4 = global write "Global Variables.vi" "Stop(QSM)"(w1) -> ()
  n5 = global write "Global Variables.vi" "Pause Parallel DAQ"(w1) -> ()
  n6 = Obtain Queue(name (unnamed)="Main Queue" ("Main Queue"), element data type=w14, error in (no error)=w6) -> (queue out=w16:refnum<queue>, error out=w17:errorcluster)  [unwired: 2 in, 1 out]
  n7 = Enqueue Element(queue=w16, element=w14, error in (no error)=w17) -> (queue out=w11:refnum<queue>, error out=w13:errorcluster)  [unwired: 1 in, 1 out]
  n8 = while {
    shift-right: [w56] -> w12
    shift-left: w11 -> [w61]
    shift-right: [w58] -> w10
    shift-left: w13 -> [w57]
    shift-right: [w21] -> _
    shift-left: "Acquisition Parameters" -> [w51]
    shift-right: [w20] -> _
    shift-left: "Hardware Parameters" -> [w50]
    shift-right: [w19] -> _
    shift-left: "Measurement Information" -> [w49]
    shift-right: [w18] -> _
    shift-left: "Spectral Data" -> [w48]
    shift-right: [w35] -> _
    shift-left: w8 -> [w45]
    shift-right: [w44] -> _
    shift-left: w6 -> [w43]
    shift-right: [w37] -> _
    shift-left: string[] [] -> [w40]
    i -> [w54]
    stop <- w33 stop-if-true
    n9 = Dequeue Element(queue=w61, error in (no error)=w57) -> (queue out=w60:refnum<queue>, element=w53:cluster{"State Control":T8, "Data":variant}, error out=w59:errorcluster)  [unwired: 1 in, 1 out]
    n10 = Format Date/Time String() -> (date/time string=w41:string)  [unwired: 3 in]
    n11 = Unbundle By Name(w53) -> ("State Control"=w27:T8)
    n12 = Equal?(x=State_Control."Idle" ("State Control"), y=w27) -> (x = y?=w22:bool)
    n13 = property on="Status of EPR DAQ" class="Enum (strict)"("Value"=w27) -> ()  [unwired: 2 in, 2 out]
    n14 = control-ref of="This VI"() -> (w47:refnum<vi>)
    n15 = case shown="True" w22 {
      frame False {
        n16 = call <vilib>:"Set Busy.vi"("disable click? (T)"=FALSE) -> ()  [unwired: 9 in, 2 out]
      }
      frame True {
        n17 = call <vilib>:"Unset Busy.vi"() -> ()  [unwired: 11 in, 1 out]
      }
    }
    n18 = Select(t=u32 6618880, s=w22, f=u32 16773418) -> (s? t:f=w24:u32)
    n19 = property on="Status of EPR DAQ" class="Enum (strict)"("RingText.BGColor"=w24) -> ()  [unwired: 2 in, 2 out]
    n20 = Insert Into Array(array=w45, new element=w27) -> (w36:T8[])  [unwired: 1 in]
    "State Control History" <- w36
    n21 = Insert Into Array(array=w40, new element=w41) -> (w38:string[])  [unwired: 1 in]
    n22 = Unbundle By Name(w53) -> ("Data"=w52:variant)
    n23 = case shown="\"Pre-Scan\"" w27 {
      tunnel: [w90 _ _ _ w272 _ w380 _ w486 cluster{"Enum":T8, "Data":variant}[] [{"Enum"=enum."Post-Scan", "Data"=variant}] w617 w766 _ _ w963 w1039 _ _ _ _ _ _ _ _ _ _ _ _ _ _ _ _ _ w1444 cluster{"Enum":T8, "Data":variant}[] [{"Enum"=enum."Idle", "Data"=variant}] _ _] -> w46
      tunnel: w59 -> [_ _ _ w254 _ w308 _ _ _ _ _ _ _ w929 w969 _ w1114 w1120 w1150 w1183 _ w1212 _ _ _ w1282 w1320 _ w1360 _ _ _ _ _ _ _ w1602]
      tunnel: [w92 w131 w244 w254 w268 w308 w369 w442 w485 w581 w598 w782 w817 w929 w969 w1028 w1114 w1120 w1150 w1183 _ w1212 w1232 w1244 w1259 w1282 w1320 w1342 w1360 w1369 w1403 w1413 _ w1429 w1497 w1537 w1602] -> w39
      tunnel: w52 -> [_ _ _ _ _ _ _ _ _ _ _ _ _ _ _ _ _ _ _ _ _ _ _ _ _ _ _ _ _ _ _ _ _ _ _ _ _]
      tunnel: [w85 w142 w235 w258 w259 w306 w372 w414 w476 w578 w612 w746 w822 w927 w965 w1036 w1108 w1123 w1131 w1181 w1194 w1217 w1236 w1248 w1261 w1278 w1327 w1351 w1363 w1371 w1408 w1416 w1428 w1439 w1491 w1536 w1609] -> w31
      tunnel: w51 -> [w86 w145 w240 w258 w260 w307 w372 w407 w475 w579 w632 w733 w827 w927 w958 w1037 w1109 w1117 w1131 w1182 w1194 w1217 w1236 w1248 w1261 w1281 w1327 w1351 w1366 w1378 w1408 w1416 w1428 w1462 w1491 w1547 w1609]
      tunnel: w50 -> [w91 w144 w237 w257 w265 w305 w368 w425 w478 w583 w631 w751 w818 w928 w962 w1033 w1116 w1128 w1152 w1174 w1193 w1216 w1227 w1247 w1260 w1280 w1325 w1343 w1365 w1379 w1407 w1415 w1427 w1461 w1507 w1549 w1608]
      tunnel: [w88 w141 w237 w257 w264 w301 w373 w418 w473 w577 w616 w756 w828 w920 w961 w1032 w1116 w1128 w1152 w1174 w1193 w1216 w1233 w1247 w1260 w1279 w1326 w1343 w1364 w1372 w1407 w1415 w1427 w1460 w1507 w1545 w1608] -> w30
      tunnel: w49 -> [w94 w143 w236 w256 w270 w304 w382 w408 w477 w585 w620 w737 w826 w926 w967 w1035 w1112 w1127 w1151 w1185 w1189 w1214 w1235 w1246 w1264 w1277 w1324 w1350 w1367 w1368 w1405 w1414 w1426 w1438 w1484 w1544 w1607]
      tunnel: [w77 w140 w236 w256 w262 w300 w382 w413 w472 w585 w618 w783 w823 w926 w959 w1034 w1111 w1127 w1151 w1185 w1190 w1211 w1235 w1246 w1264 w1276 w1324 w1350 w1367 w1373 w1405 w1414 w1426 w1430 w1484 w1541 w1607] -> w29
      tunnel: w48 -> [w87 w136 w245 w255 w269 w303 w381 w430 w487 w588 w630 w770 w825 w925 w966 w1038 w1115 w1126 w1148 w1184 w1192 w1215 w1234 w1245 w1263 w1273 w1323 w1349 w1362 w1374 w1406 w1412 w1425 w1463 w1496 w1543 w1606]
      tunnel: [w76 w134 w245 w255 w276 w302 w381 w429 w484 w586 w601 w763 w824 w925 w964 w1038 w1115 w1126 w1148 w1184 w1192 w1215 w1234 w1245 w1263 w1273 w1323 w1349 w1362 w1377 w1406 w1412 w1425 w1463 w1495 w1539 w1606] -> w28
      tunnel: w47 -> [w93 w130 _ _ w289 w297 _ _ w474 _ _ w784 _ _ _ _ _ _ _ _ _ _ _ _ _ _ _ _ _ _ _ _ _ _ w1506 _ _]
      tunnel: w43 -> [_ _ _ _ _ _ _ _ _ _ _ _ _ _ _ _ _ _ _ _ _ _ _ _ _ _ _ _ _ _ _ _ _ _ _ _ w1603]
      tunnel: w38 -> [_ _ _ _ _ _ _ _ _ _ _ _ _ _ _ _ _ _ _ _ _ _ _ _ _ _ _ _ _ _ _ _ _ _ w1500 _ _]
      tunnel: w36 -> [_ _ _ _ _ _ _ _ _ _ _ _ _ _ _ _ _ _ _ _ _ _ _ _ _ _ _ _ _ _ _ _ _ _ w1499 _ _]
      tunnel: [_ _ _ _ _ _ _ _ _ _ _ _ _ _ _ _ _ _ _ _ _ _ _ _ _ _ _ _ _ _ _ _ _ _ TRUE ("Erase History? (f)") _ _] -> w34
      frame "Startup" {
        n24 = flat-sequence {
          tunnel: w94 -> [w98]
          tunnel: w93 -> [w106]
          tunnel: [w107] -> w84
          tunnel: w91 -> [w99]
          tunnel: [w96] -> w83
          tunnel: [w102] -> w82
          tunnel: w87 -> [w102]
          tunnel: w86 -> [w100]
          tunnel: [w97] -> w81
          tunnel: [w101] -> w80
          tunnel: w84 -> [w115]
          tunnel: [w115] -> w75
          tunnel: [w112] -> w73
          tunnel: w83 -> [w112]
          tunnel: w82 -> [w111]
          tunnel: [w111] -> w71
          tunnel: w81 -> [w110]
          tunnel: [w110] -> w69
          tunnel: [w109] -> w79
          tunnel: w75 -> [w117]
          tunnel: [w117] -> w74
          tunnel: w73 -> [w120]
          tunnel: [w120] -> w72
          tunnel: w71 -> [w119]
          tunnel: [w119] -> w70
          tunnel: w69 -> [w118]
          tunnel: [w118] -> w68
          tunnel: [w129] -> w66
          tunnel: w74 -> [w129]
          tunnel: [w124] -> w90
          tunnel: w72 -> [w126]
          tunnel: [w125] -> w88
          tunnel: [w123] -> w89
          tunnel: w70 -> [w128]
          tunnel: [w128] -> w78
          tunnel: w68 -> [w127]
          tunnel: [w127] -> w85
          tunnel: [w122] -> w67
          frame #0 {
            n25 = property class="VI"(reference=w106) -> ("Name"=w108:string)  [unwired: 1 in, 2 out]
            n26 = global write "Global Variables.vi" "Finished scanning?"(TRUE ("Finished scanning?")) -> ()
            n27 = call "Read from Config File-Rev4.vi"("Measurement Information In"=w98, "Hardware Parameters In"=w99, "Acquisition Parameters In"=w100) -> ("Measurement Information Out"=w95:T3, "Hardware Parameters Out"=w96:T6, "Acquisition Parameters Out"=w97:T7)  [unwired: 1 in, 1 out]
            n28 = Bundle By Name(cluster=w95, "EPR DAQ Version"=w108) -> (w107:T3)
            n29 = call "Zero Sweep.vi"() -> ("error out"=w101:errorcluster)  [unwired: 11 in]
            n30 = call "Enable and Disable Panel Controls.vi"("VI Reference In"=w106, "Disabled"=T10."Disabled and Grayed Out", "Items to Hide"=string[] ["Scan?", "End Session?", "Manual Tuning", "Auto-Tune", "Calibrate", "Flag Bad Set", "Apply & Lock Center Field"]) -> ()  [unwired: 2 in, 1 out]
          }
          frame #1 {
            n31 = call "Set MC Analog Out.vi"("Channel"=1, "Output Voltage"=sgl 0.0) -> ("error out"=w109:errorcluster)  [unwired: 9 in]
          }
          frame #2 {
            n32 = Unbundle By Name(w117) -> ("Safe Shutdown?"=w116:bool)
            n33 = case shown="False" w116 {
              frame False {
                n34 = One Button Dialog(message="EPR DAQ has recovered from a crash.\n\nIf you believe this crash was a result of a malfunction of the \nEPR DAQ, please contact the engineers at Clin-EPR") -> ()  [unwired: 1 in, 1 out]
              }
              frame True {
              }
            }
          }
          frame #3 {
            n35 = call "Startup Lockin.vi"("Hardware Parameters In"=w126) -> ("error out"=w123:errorcluster, "QSM Response"=w124:cluster{"Enum":T8, "Data":variant}[], "Lockin OK?"=w122:bool, "Hardware Parameters Out"=w125:T6)  [unwired: 7 in]
          }
        }
        n36 = Merge Errors(w89, w79, w80) -> (w92:errorcluster)
        n37 = property on="Lock-In OK?" class="Bool (strict)"("Value"=w67) -> ()  [unwired: 2 in, 2 out]
        n38 = Unbundle By Name(w66) -> ("DAQ Mode"=w65:enum16{"Engineering", "Dosimetry", "Oximetry"})
        n39 = Equal?(x=w65, y=enum16{"Engineering", "Dosimetry", "Oximetry"}."Dosimetry" ("DAQ Mode")) -> (x = y?=w63:bool)
        n40 = Not(x=w63) -> (.not. x?=w62:bool)
        n41 = property on="Visible-Center PDT" class="Bool (strict)"("Value"=w62) -> ()  [unwired: 2 in, 2 out]
        n42 = call "Clear Measurement Info and Spectral Data.vi"("Spectral Data In"=w78, "Measurement Information In"=w66) -> ("Spectral Data Out"=w76:T1, "Measurement Information Out"=w77:T3)  [unwired: 8 in]
      }
      frame "Read Config File" {
        n43 = flat-sequence {
          tunnel: w145 -> [w149]
          tunnel: w144 -> [w153]
          tunnel: w143 -> [w152]
          tunnel: [w148] -> w139
          tunnel: [w147] -> w138
          tunnel: [w146] -> w137
          tunnel: w136 -> [w151]
          tunnel: [w151] -> w135
          tunnel: [w150] -> w133
          tunnel: [w223] -> w140
          tunnel: [w224] -> w141
          tunnel: [w232] -> w142
          tunnel: w139 -> [w232]
          tunnel: w138 -> [w224]
          tunnel: w137 -> [w223]
          tunnel: [w231] -> w134
          tunnel: w135 -> [w231]
          tunnel: [w227] -> w132
          tunnel: w130 -> [w222]
          frame #0 {
            n44 = call "Read from Config File-Rev4.vi"("Measurement Information In"=w152, "Hardware Parameters In"=w153, "Acquisition Parameters In"=w149) -> ("error out"=w150:errorcluster, "Measurement Information Out"=w146:T3, "Hardware Parameters Out"=w147:T6, "Acquisition Parameters Out"=w148:T7)  [unwired: 1 in]
            n45 = stacked-sequence {
              tunnel: w148 -> [w156 _ _]
              tunnel: w147 -> [_ w170 _]
              tunnel: w146 -> [_ _ w188]
              frame #0 {
                n46 = Unbundle By Name(w156) -> ("Central Field [G]"=w158:dbl, "Scan Time [s]"=w159:dbl, "Scan Width [G]"=w160:dbl, "Mod. Amp. [G]"=w161:dbl, "Pre-Scan Delay [ms]"=w162:u32, "Measurement Timeout [s]"=w167:dbl, "No. Scans/Set"=w163:u32, "Adaptive Processing"=w164:bool, "Adaptive Tuning"=w165:bool, "Electromagnet Main Field [G]"=w166:dbl, "Continuous Sweeping"=w168:bool, "AFC Field Correction"=w157:bool, "Sweep Rise Time [sec]"=w155:u32, "Acquire SpO2"=w154:bool)
                n47 = property on="Acquire SpO2" class="Bool (strict)"("Value"=w154) -> ()  [unwired: 2 in, 2 out]
                n48 = property on="Central field (Gauss)" class="DigNum (strict)"("Value"=w158) -> ()  [unwired: 2 in, 2 out]
                n49 = property on="Scan time (sec)" class="DigNum (strict)"("Value"=w159) -> ()  [unwired: 2 in, 2 out]
                n50 = property on="Scan range (Gauss)" class="DigNum (strict)"("Value"=w160) -> ()  [unwired: 2 in, 2 out]
                n51 = property on="Mod. Amp. (Gauss)" class="DigNum (strict)"("Value"=w161) -> ()  [unwired: 2 in, 2 out]
                n52 = property on="Prescan delay (ms)" class="DigNum (strict)"("Value"=w162) -> ()  [unwired: 2 in, 2 out]
                n53 = property on="Timer Value" class="DigNum (strict)"("Value"=w167) -> ()  [unwired: 2 in, 2 out]
                n54 = property on="No. Scans/Set" class="DigNum (strict)"("Value"=w163) -> ()  [unwired: 2 in, 2 out]
                n55 = property on="Adaptive Evaluation" class="Bool (strict)"("Value"=w164) -> ()  [unwired: 2 in, 2 out]
                n56 = property on="AdaptiveTune_Enable" class="Bool (strict)"("Value"=w165) -> ()  [unwired: 2 in, 2 out]
                n57 = property on="Electromagnet Main Field (Gauss)" class="DigNum (strict)"("Value"=w166) -> ()  [unwired: 2 in, 2 out]
                n58 = property on="Continuous Sweeping" class="Bool (strict)"("Value"=w168) -> ()  [unwired: 2 in, 2 out]
                n59 = property on="AFC Field Correction" class="Bool (strict)"("Value"=w157) -> ()  [unwired: 2 in, 2 out]
                n60 = property on="Sweep Rise [sec]" class="DigNum (strict)"("Value"=w155) -> ()  [unwired: 2 in, 2 out]
              }
              frame #1 {
                n61 = Unbundle By Name(w170) -> ("Scan Calibration [G/V]"=w171:dbl, "Modulation Calibration [G/V]"=w172:dbl, "Modulation Phase [deg]"=w173:dbl, "Modulation Frequency [Hz]"=w174:dbl, "Attenuation [dB]"=w175:u16, "Input Channel Count"=w176:i32, "Time constant"=w177:u16, "Sensitivity"=w178:u16, "Lock-in Offset Compensation"=w179:bool, "Magnet Rotation"=w180:bool, "Sweep Waveform"=w181:T9, "Balance Scaling Factor"=w182:dbl, "Phase Error Scaling Factor"=w183:dbl, "AFC Error Scaling Factor"=w184:dbl, "Sweep Limit [Gauss]"=w185:dbl, "Modulation Limit [Gauss]"=w186:dbl, "SpO2 Calibration [SpO2/V]"=w169:dbl)
                n62 = property on="Scan [Gauss/V]" class="DigNum (strict)"("Value"=w171) -> ()  [unwired: 2 in, 2 out]
                n63 = property on="Mod. [Gauss/Vrms]" class="DigNum (strict)"("Value"=w172) -> ()  [unwired: 2 in, 2 out]
                n64 = property on="Phase [deg]" class="DigNum (strict)"("Value"=w173) -> ()  [unwired: 2 in, 2 out]
                n65 = property on="Frequency [Hz]" class="DigNum (strict)"("Value"=w174) -> ()  [unwired: 2 in, 2 out]
                n66 = property on="Attenuation [dB]" class="DigNum (strict)"("Value"=w175) -> ()  [unwired: 2 in, 2 out]
                n67 = property on="Input Channel Count" class="DigNum (strict)"("Value"=w176) -> ()  [unwired: 2 in, 2 out]
                n68 = property on="Time constant" class="Ring (strict)"("Value"=w177) -> ()  [unwired: 2 in, 2 out]
                n69 = property on="Sensitivity" class="Ring (strict)"("Value"=w178) -> ()  [unwired: 2 in, 2 out]
                n70 = property on="Offset comp.?" class="Bool (strict)"("Value"=w179) -> ()  [unwired: 2 in, 2 out]
                n71 = property on="Magnet Rotation" class="Bool (strict)"("Value"=w180) -> ()  [unwired: 2 in, 2 out]
                n72 = property on="SpO2 Calibration [SpO2/V]" class="DigNum (strict)"("Value"=w169) -> ()  [unwired: 2 in, 2 out]
                n73 = property on="Sweep Waveform" class="Enum (strict)"("Value"=w181) -> ()  [unwired: 2 in, 2 out]
                n74 = property on="Balance Scale Factor" class="DigNum (strict)"("Value"=w182) -> ()  [unwired: 2 in, 2 out]
                n75 = property on="Phase Scale Factor" class="DigNum (strict)"("Value"=w183) -> ()  [unwired: 2 in, 2 out]
                n76 = property on="AFC Scale Factor" class="DigNum (strict)"("Value"=w184) -> ()  [unwired: 2 in, 2 out]
                n77 = property on="Scan range (Gauss)" class="DigNum (strict)"("Maximum"=w185) -> ()  [unwired: 2 in, 2 out]
                n78 = property on="Mod. Amp. (Gauss)" class="DigNum (strict)"("Maximum"=w186) -> ()  [unwired: 2 in, 2 out]
              }
              frame #2 {
                n79 = Unbundle By Name(w188) -> ("Data file path"=w191:path, "Session Number"=w192:i32, "Report pO2/Scan"=w189:bool, "Oxy Exclude Unacceptable"=w187:bool, "DAQ Mode"=w190:enum16{"Engineering", "Dosimetry", "Oximetry"})  [unwired: 1 out]
                n80 = Current VI's Menubar() -> (w193:refnum<k9>)
                n81 = property on="Data file path" class="Path"("Value"=w191) -> ()  [unwired: 2 in, 2 out]
                n82 = property on="Session Number" class="DigNum (strict)"("Value"=w192) -> ()  [unwired: 2 in, 2 out]
                n83 = property on="Report pO2/Scan" class="Bool (strict)"("Value"=w189) -> ()  [unwired: 2 in, 2 out]
                n84 = property on="Exclude Unacceptable pO2" class="Bool (strict)"("Value"=w187) -> ()  [unwired: 2 in, 2 out]
                n85 = property on="DAQ Mode" class="Enum (strict)"("Value"=w190) -> ()  [unwired: 2 in, 2 out]
                n86 = case shown="\"Engineering\"" w190 {
                  tunnel: w193 -> [w198 w207 w216 _]
                  frame "Dosimetry" {
                    n87 = Set Menu Item Info(6:TRUE ("checked"), 7:"Dosimetry" ("item tag"), 11:w198) -> (3:w197:refnum<k9>)  [unwired: 4 in, 1 out]
                    n88 = Set Menu Item Info(6:FALSE ("checked"), 7:"Oximetry" ("item tag"), 11:w197) -> (3:w202:refnum<k9>)  [unwired: 4 in, 1 out]
                    n89 = Set Menu Item Info(6:FALSE ("checked"), 7:"Engineering" ("item tag"), 11:w202) -> ()  [unwired: 4 in, 2 out]
                  }
                  frame "Oximetry" {
                    n90 = Set Menu Item Info(6:FALSE ("checked"), 7:"Dosimetry" ("item tag"), 11:w207) -> (3:w206:refnum<k9>)  [unwired: 4 in, 1 out]
                    n91 = Set Menu Item Info(6:TRUE ("checked"), 7:"Oximetry" ("item tag"), 11:w206) -> (3:w211:refnum<k9>)  [unwired: 4 in, 1 out]
                    n92 = Set Menu Item Info(6:FALSE ("checked"), 7:"Engineering" ("item tag"), 11:w211) -> ()  [unwired: 4 in, 2 out]
                  }
                  frame "Engineering" {
                    n93 = Set Menu Item Info(6:FALSE ("checked"), 7:"Dosimetry" ("item tag"), 11:w216) -> (3:w215:refnum<k9>)  [unwired: 4 in, 1 out]
                    n94 = Set Menu Item Info(6:FALSE ("checked"), 7:"Oximetry" ("item tag"), 11:w215) -> (3:w220:refnum<k9>)  [unwired: 4 in, 1 out]
                    n95 = Set Menu Item Info(6:TRUE ("checked"), 7:"Engineering" ("item tag"), 11:w220) -> ()  [unwired: 4 in, 2 out]
                  }
                  frame Default {
                  }
                }
              }
            }
          }
          frame #1 {
            w225 = u16 0 items=["Hide", "Show"] ("Operation")
            n96 = call "Define Controls to Hide.vi"("Other Controls to Hide"=string[] ["of", "Scan no."] ("Items to Hide"), "Measurement Information"=w223, "Hardware Parameters"=w224) -> ("Controls to Hide"=w226:string[])  [unwired: 8 in]
            n97 = call-poly "Write Config Key.vi"("value"=FALSE ("Safe Shutdown?"), "key"="safe_shutdown", "section"="logging") -> ("error out"=w227:errorcluster)  [unwired: 8 in]
            n98 = call "Show and Hide Panel Controls.vi"("VI Reference In"=w222, "Operation"=w225, "Items to Hide"=w226) -> ()  [unwired: 2 in, 1 out]
          }
        }
        n99 = Merge Errors(w132, w133) -> (w131:errorcluster)
      }
      frame "Initilize Optional Hardware" {
        n100 = Unbundle By Name(w237) -> ("Magnet Type"=w243:T11)
        n101 = Equal?(x=w243, y=T11."RRI Electromagnet" ("Magnet Type")) -> (x = y?=w241:bool)
        n102 = case shown="True" w241 {
          tunnel: w240 -> [w246 w250]
          tunnel: w237 -> [_ w252]
          tunnel: [errorcluster {"status"=FALSE, "code"=0, "source"=""} ("error out") w251] -> w239
          tunnel: [w246 w248] -> w238
          frame False {
          }
          frame True {
            w249 = 0.0 ("Y-Gradient [G/mm]")
            n103 = Bundle By Name(cluster=w250, "X-Gradient [G/mm]"=w249, "Y-Gradient [G/mm]"=w249, "Z-Gradient [G/mm]"=w249) -> (w248:T7)
            n104 = call "RRI LoadGo - Electromagnet.vi"("Control Coils"=T12."Main and Gradients", "Hardware Parameters"=w252, "Acquisition Parameters"=w248) -> ("error out"=w251:errorcluster)  [unwired: 4 in]
          }
        }
        n105 = call "In-Context Initialize Optional Hardware.vi"("Measurement Information In"=w236, "Hardware Parameters In"=w237, "Acquisition Parameters In"=w238) -> ("error out"=w234:errorcluster, "Magnet Angle [deg]"=w233:dbl, "Acquisition Parameters Out"=w235:T7)  [unwired: 6 in]
        n106 = property on="Magnet Angle (deg)" class="DigNum (strict)"("Value"=w233) -> ()  [unwired: 2 in, 2 out]
        n107 = Merge Errors(w234, w239) -> (w244:errorcluster)
      }
      frame "Idle", Default {
      }
      frame "New Session" {
        n108 = property on="New Session" class="Bool (strict)"("Value"=FALSE ("New Session")) -> ()  [unwired: 2 in, 2 out]
        n109 = call "Enable and Disable Panel Controls.vi"("VI Reference In"=w289, "Disabled"=T10."Disabled and Grayed Out", "Items to Hide"=string[] ["New Session", "Quit"]) -> ()  [unwired: 2 in, 1 out]
        n110 = call "Initialize Session.vi"("Acquisition Parameters In"=w260, "Spectral Data In"=w269, "Measurement Information In"=w270, "Hardware Parameters In"=w265) -> ("QSM Response"=w272:cluster{"Enum":T8, "Data":variant}[], "Spectral Data Out"=w266:T1, "Measurement Information Out"=w267:T3, "Hardware Parameters Out"=w264:T6, "error out"=w268:errorcluster, "Acquisition Parameters Out"=w259:T7)  [unwired: 2 in]
        n111 = Unbundle By Name(w267) -> ("Resonator Operator"=w284:string, "Computer Operator"=w283:string, "Tooth/Sample ID"=w275:string, "Volunteer ID"=w281:string, "Gases Available"=w279:string[], "Session Number"=w280:i32, "Session Type"=w273:string, "Set #"=w271:u32)  [unwired: 2 out]
        n112 = Unbundle By Name(w264) -> ("Sensitivity"=w263:u16)
        n113 = Concatenate Strings(w284, "-" ("string"), w283) -> (w282:string)
        n114 = Decrement(x=w271) -> (x-1=w278:u32)
        n115 = property on="Operators" class="Str"("Value"=w282) -> ()  [unwired: 2 in, 2 out]
        n116 = property on="Sample ID" class="Str"("Value"=w275) -> ()  [unwired: 2 in, 2 out]
        n117 = property on="Volunteer ID" class="Str"("Value"=w281) -> ()  [unwired: 2 in, 2 out]
        n118 = property on="Initial State" class="Ring (strict)"("Strings []"=w279) -> ()  [unwired: 2 in, 2 out]
        n119 = property on="Applied State" class="Ring (strict)"("Strings []"=w279) -> ()  [unwired: 2 in, 2 out]
        n120 = property on="Session Number" class="DigNum (strict)"("Value"=w280) -> ()  [unwired: 2 in, 2 out]
        n121 = property on="Session Type" class="Str"("Value"=w273) -> ()  [unwired: 2 in, 2 out]
        n122 = property on="Sets Completed" class="DigNum (strict)"("Value"=w278) -> ()  [unwired: 2 in, 2 out]
        n123 = property on="Sensitivity" class="Ring (strict)"("Value"=w263) -> ()  [unwired: 2 in, 2 out]
        n124 = To Lower Case(string=w275) -> (all lower case string=w274:string)
        n125 = case shown="\"oxychip\"" w274 {
          tunnel: w267 -> [w290 w292]
          tunnel: [w290 w291] -> w262
          frame "False", Default {
          }
          frame "oxychip" {
            n126 = call "OxyChip Calibration Prompt.vi"("Measurement Information In"=w292) -> ("Measurement Information Out"=w291:T3)  [unwired: 10 in]
          }
        }
        n127 = call "Choose Fitting Model.vi"("Spectral Data In"=w266, "Measurement Information In"=w262) -> ("Model Select"=w277:T2, "Spectral Data Out"=w276:T1)  [unwired: 8 in]
        n128 = Unbundle By Name(w262) -> ("Report pO2/Scan"=w261:bool)
        n129 = property on="Model Select" class="Enum (strict)"("Value"=w277) -> ()  [unwired: 2 in, 2 out]
        n130 = property on="Report pO2/Scan" class="Bool (strict)"("Value"=w261) -> ()  [unwired: 2 in, 2 out]
      }
      frame "Read GUI Pars" {
        w298 = u16 0 items=["Hide", "Show"] ("Operation")
        n131 = stacked-sequence {
          tunnel: w307 -> [w324 _ _ _]
          tunnel: [w323 _ _ _] -> w306
          tunnel: w305 -> [_ w336 _ _]
          tunnel: [_ w335 _ _] -> w301
          tunnel: w304 -> [_ _ w353 _]
          tunnel: [_ _ w352 _] -> w300
          tunnel: w303 -> [_ _ _ w362]
          tunnel: [_ _ _ w361] -> w302
          frame #0 {
            n132 = property on="X-Gradient [G/mm]" class="DigNum (strict)"() -> ("Value"=w321:dbl)  [unwired: 2 in, 2 out]
            n133 = property on="Y-Gradient [G/mm]" class="DigNum (strict)"() -> ("Value"=w320:dbl)  [unwired: 2 in, 2 out]
            n134 = property on="Z-Gradient [G/mm]" class="DigNum (strict)"() -> ("Value"=w319:dbl)  [unwired: 2 in, 2 out]
            n135 = property on="Continuous Sweeping" class="Bool (strict)"() -> ("Value"=w316:bool)  [unwired: 2 in, 2 out]
            n136 = property on="Sweep Rise [sec]" class="DigNum (strict)"() -> ("Value"=w315:u32)  [unwired: 2 in, 2 out]
            n137 = property on="AFC Field Correction" class="Bool (strict)"() -> ("Value"=w313:bool)  [unwired: 2 in, 2 out]
            n138 = property on="Magnet Angle (deg)" class="DigNum (strict)"() -> ("Value"=w312:dbl)  [unwired: 2 in, 2 out]
            n139 = property on="Acquisition Updates Prescribe" class="Bool (strict)"() -> ("Value"=w311:bool)  [unwired: 2 in, 2 out]
            n140 = property on="Central field (Gauss)" class="DigNum (strict)"() -> ("Value"=w314:dbl)  [unwired: 2 in, 2 out]
            n141 = property on="Scan time (sec)" class="DigNum (strict)"() -> ("Value"=w328:dbl)  [unwired: 2 in, 2 out]
            n142 = property on="Scan range (Gauss)" class="DigNum (strict)"() -> ("Value"=w327:dbl)  [unwired: 2 in, 2 out]
            n143 = property on="Mod. Amp. (Gauss)" class="DigNum (strict)"() -> ("Value"=w326:dbl)  [unwired: 2 in, 2 out]
            n144 = property on="Prescan delay (ms)" class="DigNum (strict)"() -> ("Value"=w325:u32)  [unwired: 2 in, 2 out]
            n145 = property on="Timer Value" class="DigNum (strict)"() -> ("Value"=w318:dbl)  [unwired: 2 in, 2 out]
            n146 = property on="No. Scans/Set" class="DigNum (strict)"() -> ("Value"=w329:u32)  [unwired: 2 in, 2 out]
            n147 = property on="Adaptive Evaluation" class="Bool (strict)"() -> ("Value"=w317:bool)  [unwired: 2 in, 2 out]
            n148 = property on="AdaptiveTune_Enable" class="Bool (strict)"() -> ("Value"=w330:bool)  [unwired: 2 in, 2 out]
            n149 = property on="Auto Set-based Field Center" class="Bool (strict)"() -> ("Value"=w331:bool)  [unwired: 2 in, 2 out]
            n150 = property on="Electromagnet Main Field (Gauss)" class="DigNum (strict)"() -> ("Value"=w332:dbl)  [unwired: 2 in, 2 out]
            n151 = property on="Prompt for acquisition updates" class="Bool (strict)"() -> ("Value"=w333:bool)  [unwired: 2 in, 2 out]
            n152 = property on="Gradients on/off" class="Bool (strict)"() -> ("Value"=w322:bool)  [unwired: 2 in, 2 out]
            n153 = Bundle By Name(cluster=w324, "Central Field [G]"=w314, "Forward Sweep Central Field [G]"=w314, "Scan Time [s]"=w328, "Scan Width [G]"=w327, "Mod. Amp. [G]"=w326, "Pre-Scan Delay [ms]"=w325, "Measurement Timeout [s]"=w318, "No. Scans/Set"=w329, "Adaptive Processing"=w317, "Adaptive Tuning"=w330, "Auto Set-based Field Center"=w331, "Electromagnet Main Field [G]"=w332, "Prompt for oxy acquisition updates"=w333, "Gradients on/off"=w322, "X-Gradient [G/mm]"=w321, "Y-Gradient [G/mm]"=w320, "Z-Gradient [G/mm]"=w319, "Continuous Sweeping"=w316, "Sweep Rise Time [sec]"=w315, "AFC Field Correction"=w313, "Magnet Angle [deg]"=w312, "Over Mod"=w311) -> (w323:T7)
            n154 = case shown="True" w317 {
              selector: w317 -> [_ w334]
              frame False {
              }
              frame True {
                n155 = property on="Fit Each Scan" class="Bool (strict)"("Value"=w334) -> ()  [unwired: 2 in, 2 out]
              }
            }
          }
          frame #1 {
            n156 = property on="Scan Gauss/V" class="DigNum (strict)"() -> ("Value"=w340:dbl)  [unwired: 2 in, 2 out]
            n157 = property on="Mod. Gauss/Vrms" class="DigNum (strict)"() -> ("Value"=w337:dbl)  [unwired: 2 in, 2 out]
            n158 = property on="Phase (deg)" class="DigNum (strict)"() -> ("Value"=w338:dbl)  [unwired: 2 in, 2 out]
            n159 = property on="Frequency (Hz)" class="DigNum (strict)"() -> ("Value"=w339:dbl)  [unwired: 2 in, 2 out]
            n160 = property on="Attenuation/dB" class="DigNum (strict)"() -> ("Value"=w342:u16)  [unwired: 2 in, 2 out]
            n161 = property on="Input Channel Count" class="DigNum (strict)"() -> ("Value"=w348:i32)  [unwired: 2 in, 2 out]
            n162 = property on="Time constant" class="Ring (strict)"() -> ("Value"=w341:u16)  [unwired: 2 in, 2 out]
            n163 = property on="Sensitivity" class="Ring (strict)"() -> ("Value"=w343:u16)  [unwired: 2 in, 2 out]
            n164 = property on="Offset comp.?" class="Bool (strict)"() -> ("Value"=w344:bool)  [unwired: 2 in, 2 out]
            n165 = property on="AFC Control" class="Bool (strict)"() -> ("Value"=w345:bool)  [unwired: 2 in, 2 out]
            n166 = property on="Magnet Rotation" class="Bool (strict)"() -> ("Value"=w346:bool)  [unwired: 2 in, 2 out]
            n167 = property on="Sweep Waveform" class="Enum (strict)"() -> ("Value"=w347:T9)  [unwired: 2 in, 2 out]
            n168 = Bundle By Name(cluster=w336, "Scan Calibration [G/V]"=w340, "Modulation Calibration [G/V]"=w337, "Modulation Phase [deg]"=w338, "Modulation Frequency [Hz]"=w339, "Attenuation [dB]"=w342, "Input Channel Count"=w348, "Time constant"=w341, "Sensitivity"=w343, "Lock-in Offset Compensation"=w344, "AFC"=w345, "Magnet Rotation"=w346, "Sweep Waveform"=w347) -> (w335:T6)
          }
          frame #2 {
            n169 = property on="Comments" class="Str"() -> ("Value"=w354:string)  [unwired: 2 in, 2 out]
            n170 = property on="Directory Input" class="Str"() -> ("Value"=w355:string)  [unwired: 2 in, 2 out]
            n171 = property on="Data file path" class="Path"() -> ("Value"=w357:path)  [unwired: 2 in, 2 out]
            n172 = property on="Scripting File" class="Path"() -> ("Value"=w356:path)  [unwired: 2 in, 2 out]
            n173 = property on="Save data" class="Bool (strict)"() -> ("Value"=w358:bool)  [unwired: 2 in, 2 out]
            n174 = property on="DAQ Mode" class="Enum (strict)"() -> ("Value"=w351:enum16{"Engineering", "Dosimetry", "Oximetry"})  [unwired: 2 in, 2 out]
            n175 = property on="Report pO2/Scan" class="Bool (strict)"() -> ("Value"=w350:bool)  [unwired: 2 in, 2 out]
            n176 = property on="Exclude Unacceptable pO2" class="Bool (strict)"() -> ("Value"=w349:bool)  [unwired: 2 in, 2 out]
            n177 = Bundle By Name(cluster=w353, "Comments"=w354, "Directory Input"=w355, "Data file path"=w357, "Scripting File"=w356, "Save Data"=w358, "DAQ Mode"=w351, "Report pO2/Scan"=w350, "Oxy Exclude Unacceptable"=w349) -> (w352:T3)
            n178 = case shown="True" w350 {
              selector: w350 -> [_ w359]
              frame False {
              }
              frame True {
                n179 = property on="Fit Each Scan" class="Bool (strict)"("Value"=w359) -> ()  [unwired: 2 in, 2 out]
              }
            }
          }
          frame #3 {
            n180 = property on="Model Select" class="Enum (strict)"() -> ("Value"=w360:T2)  [unwired: 2 in, 2 out]
            n181 = property on="Fit Each Scan" class="Bool (strict)"() -> ("Value"=w363:bool)  [unwired: 2 in, 2 out]
            n182 = property on="Baseline Correction" class="Bool (strict)"() -> ("Value"=w364:bool)  [unwired: 2 in, 2 out]
            n183 = Bundle By Name(cluster=w362, "Model Select"=w360, "Fit Each Scan"=w363, "Baseline Offset Correction"=w364) -> (w361:T1)
          }
        }
        n184 = property on="Scan?" class="Bool (strict)"() -> ("Value"=w293:bool)  [unwired: 2 in, 2 out]
        n185 = case shown="True" w293 {
          tunnel: [string[] ["of", "Scan no.", "Manual Tuning", "Auto-Tune", "Calibrate", "Scan?", "End Session?", "Flag Bad Set"] ("Items to Hide") string[] ["of", "Scan no."] ("Items to Hide")] -> w296
          frame True {
          }
          frame False {
          }
        }
        n186 = property on="Show Calibration Constants" class="Bool (strict)"() -> ("Value"=w294:bool)  [unwired: 2 in, 2 out]
        n187 = property on="Mode" class="Bool (strict)"() -> ("Value"=w295:bool)  [unwired: 2 in, 2 out]
        n188 = call "Define Controls to Hide.vi"("Troubleshooting Mode? (f)"=w295, "Show Calibration Values? (f)"=w294, "Other Controls to Hide"=w296, "Measurement Information"=w300, "Hardware Parameters"=w301) -> ("Controls to Hide"=w299:string[])  [unwired: 6 in]
        n189 = call "Show and Hide Panel Controls.vi"("VI Reference In"=w297, "Operation"=w298, "Items to Hide"=w299) -> ()  [unwired: 2 in, 1 out]
      }
      frame "Configure Hardware" {
        n190 = call "Check Lockin.vi"("Hardware Parameters"=w368) -> ("error out"=w365:errorcluster, "Lockin OK?"=w366:bool, "Hardware Parameters Out"=w367:T6)  [unwired: 8 in]
        n191 = case shown="False" w366 {
          tunnel: [w394 w404] -> w379
          tunnel: [w388 w403] -> w371
          tunnel: [w393 _] -> w380
          tunnel: w367 -> [w390 w404]
          tunnel: w372 -> [w389 w405]
          tunnel: w365 -> [w388 w402]
          frame False {
            n192 = Unbundle By Name(w390) -> ("Ignore Lock-in Comm. Failure"=w392:bool)
            n193 = case shown="False" w392 {
              selector: w392 -> [_ w401]
              tunnel: [w399 _] -> w393
              tunnel: [w398 w401] -> w391
              tunnel: w390 -> [_ _]
              tunnel: w389 -> [_ _]
              frame False {
                n194 = Two Button Dialog(message="Unable to communicate with lock in amplifier. \nDo you want to continue, or quit the software?", 1:"Quit" ("F button name (\"Cancel\")"), 2:"Continue" ("T button name (\"OK\")")) -> (T button?=w398:bool)
                n195 = case shown="False" w398 {
                  tunnel: [cluster{"Enum":T8, "Data":variant}[] [{"Enum"=enum."Quit Software", "Data"=variant}] _] -> w399
                  frame False {
                  }
                  frame True {
                  }
                }
              }
              frame True {
              }
            }
            n196 = Bundle By Name(cluster=w390, "Ignore Lock-in Comm. Failure"=w391) -> (w394:T6)
          }
          frame True {
            n197 = call "Configure Lock-in.vi"("error in (no error)"=w402, "Hardware Parameters"=w404, "Acquisition Parameters"=w405) -> ("error out"=w403:errorcluster)  [unwired: 8 in]
          }
        }
        n198 = call "MiniCircuits UFC-6000 Read Frequency.vi"("Hardware Parameters In"=w379) -> ("Hardware Parameters Out"=w373:T6)  [unwired: 9 in, 1 out]
        n199 = Unbundle By Name(w373) -> ("RF [GHz]"=w378:dbl, "Lock-in OK?"=w377:bool)
        n200 = property on="RF (GHz)" class="DigNum (strict)"("Value"=w378) -> ()  [unwired: 2 in, 2 out]
        n201 = property on="Lock-In OK?" class="Bool (strict)"("Value"=w377) -> ()  [unwired: 2 in, 2 out]
        n202 = Unbundle By Name(w373) -> ("Magnet Type"=w376:T11)
        n203 = Equal?(x=w376, y=T11."RRI Electromagnet" ("Magnet Type")) -> (x = y?=w374:bool)
        n204 = case shown="True" w374 {
          tunnel: w372 -> [_ w384]
          tunnel: w373 -> [_ w386]
          tunnel: [errorcluster {"status"=FALSE, "code"=0, "source"=""} ("error out") w385] -> w370
          frame False {
          }
          frame True {
            n205 = call "RRI LoadGo - Electromagnet.vi"("Control Coils"=T12."Main Field", "Hardware Parameters"=w386, "Acquisition Parameters"=w384) -> ("error out"=w385:errorcluster)  [unwired: 4 in]
          }
        }
        n206 = Merge Errors(w370, w371) -> (w369:errorcluster)
      }
      frame "Initialize Set" {
        w446 = u32 0 ("Scans Completed")
        n207 = property on="No. Scans/Set" class="DigNum (strict)"() -> ("Value"=w444:u32)  [unwired: 2 in, 2 out]
        n208 = global write "Global Variables.vi" "Finished scanning?"(FALSE ("Finished scanning?")) -> ()
        n209 = property on="Unacceptable pO2 Estimate" class="Bool (strict)"("Value"=FALSE ("Unacceptable pO2 Estimate")) -> ()  [unwired: 2 in, 2 out]
        n210 = property on="of" class="DigNum (strict)"("Value"=w444) -> ()  [unwired: 2 in, 2 out]
        n211 = call "Check for Save Data.vi"("Measurement Information In"=w408, "Acquisition Parameters In"=w407) -> ("Measurement Information Out"=w410:T3, "Save Data Out"=w409:bool)  [unwired: 8 in]
        n212 = property on="Save data" class="Bool (strict)"("Value"=w409) -> ()  [unwired: 2 in, 2 out]
        n213 = call "Initialize Arrays for New Set.vi"("Spectral Data In"=w430, "Measurement Information In"=w410) -> ("Spectral Data Out"=w429:T1, "Measurement Information Out"=w417:T3)  [unwired: 8 in]
        n214 = Bundle By Name(cluster=w425, "Consecutive Re-tune attempts"=0) -> (w424:T6)
        n215 = Increment(x=w446) -> (x+1=w445:u32)
        n216 = Bundle By Name(cluster=w407, "Scans Completed"=w446) -> (w431:T7)
        n217 = property on="Set Progress" class="Slide (strict)"("Value"=0.0 ("Set Progress"), "Fill Color"=u32 16711680) -> ()  [unwired: 2 in, 2 out]
        n218 = property on="Scan no." class="DigNum (strict)"("Value"=w445) -> ()  [unwired: 2 in, 2 out]
        n219 = Unbundle By Name(w425) -> ("Lock-in OK?"=w432:bool)
        n220 = Unbundle By Name(w431) -> ("Acquire Q"=w437:bool)
        n221 = Unbundle By Name(w417) -> ("Save Data"=w436:bool)
        n222 = Compound Arithmetic op=AND(w432, w437, w436) -> (w435:bool)
        n223 = case shown="False" w435 {
          tunnel: w424 -> [w448 w452]
          tunnel: [w448 w451] -> w434
          tunnel: [_ w450] -> w428
          tunnel: [nan ("Q Factor") w449] -> w433
          frame False {
          }
          frame True {
            n224 = call "Measure Q.vi"("Hardware Parameters"=w452) -> ("error out"=w450:errorcluster, "Q Factor"=w449:dbl, "Hardware Parameters Out"=w451:T6)  [unwired: 8 in]
          }
        }
        n225 = property on="Q Start" class="DigNum (strict)"("Value"=w433) -> ()  [unwired: 2 in, 2 out]
        n226 = Unbundle By Name(w431) -> ("Acquire Photos"=w439:bool)
        n227 = Unbundle By Name(w417) -> ("Save Data"=w440:bool)
        n228 = And(x=w439, y=w440) -> (x .and. y?=w438:bool)
        n229 = case shown="True" w438 {
          tunnel: w434 -> [_ w463]
          tunnel: w417 -> [_ w462]
          tunnel: w429 -> [_ w465]
          tunnel: w431 -> [_ w464]
          tunnel: [errorcluster {"status"=FALSE, "code"=0, "source"=""} ("error out") _] -> w427
          frame False {
          }
          frame True {
            # "0.2.5.14 - Removed\nCamera Grab_AG.vi"
            n230 = call "Save EPR Data-Rev3.vi"("Save Data Type"=Save_Data_Type."Filename", "Spectral Data"=w465, "Measurement Information"=w462, "Hardware Parameters"=w463, "Acquisition Parameters"=w464) -> ()  [unwired: 5 in, 1 out]
          }
        }
        n231 = Unbundle By Name(w431) -> ("Auto Set-based Field Center"=w441:bool)
        n232 = case shown="True" w441 {
          tunnel: w434 -> [w453 w459]
          tunnel: [w454 w456] -> w419
          tunnel: [w453 w458] -> w418
          tunnel: w431 -> [w454 w457]
          frame False {
          }
          frame True {
            n233 = call "Software-Based FFL.vi"("Hardware Parameters In"=w459, "Acquisition Parameters In"=w457) -> ("Central Field [G]"=w455:dbl, "Hardware Parameters Out"=w458:T6, "Acquisition Parameters Out"=w456:T7)  [unwired: 3 in]
            n234 = property on="Central field (Gauss)" class="DigNum (strict)"("Value"=w455) -> ()  [unwired: 2 in, 2 out]
          }
        }
        n235 = local read "Timer on/off"() -> (w421:bool)
        n236 = property on="Initial State" class="Ring (strict)"() -> ("Value"=w416:i32)  [unwired: 2 in, 2 out]
        n237 = property on="Applied State" class="Ring (strict)"() -> ("Value"=w415:i32)  [unwired: 2 in, 2 out]
        n238 = call "In-Context Initialize Set.vi"("Acquisition Parameters In"=w419, "Hardware Parameters In"=w418, "Measurement Information In"=w417, "Initial State"=w416, "Applied State"=w415, "Timer on/off In"=w421) -> ("Acquisition Parameters Out"=w414:T7, "Measurement Information Out"=w413:T3, "Magnet Angle [deg]"=w411:dbl, "Timer on/off Out"=w420:bool, "error out"=w412:errorcluster)  [unwired: 5 in]
        n239 = local write "Timer on/off"(w420) -> ()
        n240 = property on="Magnet Angle (deg)" class="DigNum (strict)"("Value"=w411) -> ()  [unwired: 2 in, 2 out]
        n241 = Merge Errors(w412, w427, w428) -> (w442:errorcluster)
      }
      frame "Pre-Scan" {
        w483 = u16 0 items=["Hide", "Show"] ("Operation")
        n242 = property on="Show Calibration Constants" class="Bool (strict)"() -> ("Value"=w480:bool)  [unwired: 2 in, 2 out]
        n243 = property on="Mode" class="Bool (strict)"() -> ("Value"=w479:bool)  [unwired: 2 in, 2 out]
        n244 = call "Define Controls to Hide.vi"("Troubleshooting Mode? (f)"=w479, "Show Calibration Values? (f)"=w480, "Other Controls to Hide"=string[] ["Scan?", "Calibration", "Optimizing Frequency", "Manual Tuning", "Auto-Tune", "Calibrate", "End Session?", "Flag Bad Set", "Apply & Lock Center Field"] ("Items to Hide"), "Measurement Information"=w477, "Hardware Parameters"=w478) -> ("Controls to Hide"=w481:string[])  [unwired: 6 in]
        n245 = call "Show and Hide Panel Controls.vi"("VI Reference In"=w474, "Operation"=w483, "Items to Hide"=w481) -> ()  [unwired: 2 in, 1 out]
        n246 = flat-sequence {
          tunnel: w487 -> [w516]
          tunnel: w478 -> [w500]
          tunnel: w477 -> [w499]
          tunnel: w475 -> [w492]
          tunnel: [w505] -> w471
          tunnel: [w503] -> w470
          tunnel: [w501] -> w469
          tunnel: [w498] -> w468
          tunnel: [w491] -> w467
          tunnel: [w490] -> w466
          tunnel: [w569] -> w472
          tunnel: [w570] -> w473
          tunnel: [w571] -> w476
          tunnel: [w572] -> w484
          tunnel: [w573] -> w485
          tunnel: [w574] -> w486
          tunnel: w471 -> [w574]
          tunnel: w470 -> [w573]
          tunnel: w469 -> [w572]
          tunnel: w468 -> [w571]
          tunnel: w467 -> [w570]
          tunnel: w466 -> [w569]
          frame #0 {
            n247 = Unbundle By Name(w492) -> ("Scans Completed/Session"=w497:u32)
            n248 = flat-sequence {
              tunnel: w500 -> [w549]
              tunnel: [w549] -> w520
              tunnel: w492 -> [w545]
              tunnel: w499 -> [w546]
              tunnel: w516 -> [w547]
              tunnel: [w547] -> w519
              tunnel: [w546] -> w518
              tunnel: [w545] -> w517
              tunnel: [w556] -> w508
              tunnel: w520 -> [w557]
              tunnel: [w555] -> w501
              tunnel: w519 -> [w555]
              tunnel: [w554] -> w490
              tunnel: w518 -> [w554]
              tunnel: [w550] -> w498
              tunnel: w517 -> [w550]
              tunnel: [w553] -> w515
              tunnel: [w552] -> w504
              frame #0 {
                n249 = global write "Global Variables.vi" "Pause Parallel DAQ"(TRUE ("Pause Parallel DAQ")) -> ()
              }
              frame #1 {
                n250 = Unbundle By Name(w550) -> ("Adaptive Tuning"=w551:bool)
                n251 = case shown="True" w551 {
                  selector: w551 -> [w558 _]
                  tunnel: w557 -> [w559 w567]
                  tunnel: [w559 w566] -> w556
                  tunnel: [w558 w562] -> w553
                  tunnel: [_ w560] -> w552
                  frame False {
                  }
                  frame True {
                    n252 = call "Check Current Tune.vi"("Time to collect [ms]"=50, "Hardware Parameters"=w567) -> ("AFC Threshold Exceeded?"=w563:bool, "Phase Threshold Exceeded?"=w564:bool, "Balance Threshold Exceeded?"=w565:bool, "Hardware Parameters Out"=w566:T6, "error out"=w560:errorcluster)  [unwired: 5 in]
                    n253 = Compound Arithmetic op=OR(w565, w564, w563) -> (w562:bool)
                  }
                }
              }
            }
            n254 = Greater?(x=w497, y=u32 0) -> (0:w495:bool)
            n255 = Select(t=T10."Disabled and Grayed Out" ("Disabled"), s=w495, f=T10."Enabled" ("Disabled")) -> (s? t:f=w488:T10)
            n256 = Unbundle By Name(w500) -> ("Consecutive Re-tune attempts"=w512:i32)
            n257 = property on="Report pO2/Scan" class="Bool (strict)"("DisabledEnum"=w488) -> ()  [unwired: 2 in, 2 out]
            n258 = property on="Exclude Unacceptable pO2" class="Bool (strict)"("DisabledEnum"=w488) -> ()  [unwired: 2 in, 2 out]
            n259 = Unbundle By Name(w492) -> ("Adaptive Tuning"=w513:bool)
            n260 = Greater Or Equal?(x=w512, y=3) -> (x >= y?=w510:bool)
            n261 = And(x=w515, y=w513) -> (x .and. y?=w514:bool)
            n262 = And(x=w513, y=w510) -> (x .and. y?=w509:bool)
            n263 = case shown="False" w509 {
              tunnel: [w532 w535] -> w507
              tunnel: w514 -> [w530 _]
              tunnel: w508 -> [w529 w542]
              tunnel: [w529 w541] -> w491
              tunnel: w498 -> [_ w539]
              frame False {
                n264 = Select(t=cluster{"Enum":T8, "Data":variant}[] [{"Enum"=enum."Automated Tuning", "Data"=variant}, {"Enum"=enum."Pre-Scan", "Data"=variant}], s=w530, f=cluster{"Enum":T8, "Data":variant}[] [{"Enum"=enum."Scan", "Data"=variant}]) -> (s? t:f=w532:cluster{"Enum":T8, "Data":variant}[])
              }
              frame True {
                n265 = Unbundle By Name(w539) -> ("Scans Completed"=w538:u32)
                n266 = global write "Global Variables.vi" "Abort Scan"(TRUE ("Abort Scan")) -> ()
                n267 = Bundle By Name(cluster=w542, "Consecutive Re-tune attempts"=0) -> (w541:T6)
                n268 = Greater Than 0?(x=w538) -> (x > 0?=w537:bool)
                n269 = One Button Dialog(message="Too many consecutive tuning attempts.\nMeasurement is being aborted.") -> ()  [unwired: 1 in, 1 out]
                n270 = Select(t=cluster{"Enum":T8, "Data":variant}[] [{"Enum"=enum."Exit Set", "Data"=variant}], s=w537, f=cluster{"Enum":T8, "Data":variant}[] [{"Enum"=enum."Read GUI Pars", "Data"=variant}, {"Enum"=enum."Idle", "Data"=variant}]) -> (s? t:f=w535:cluster{"Enum":T8, "Data":variant}[])
              }
            }
            n271 = call "Check for Lock-in Saturation.vi"("Hardware Parameters"=w491) -> ("error out"=w502:errorcluster, "Continue Measurement"=w489:bool)  [unwired: 9 in]
            n272 = case shown="False" w489 {
              tunnel: w491 -> [w523 _]
              tunnel: w490 -> [w522 _]
              frame False {
                w528 = u16 0 items=["Hide", "Show"] ("Operation")
                n273 = control-ref of="This VI"() -> (w521:refnum<vi>)
                n274 = property on="Show Calibration Constants" class="Bool (strict)"() -> ("Value"=w525:bool)  [unwired: 2 in, 2 out]
                n275 = property on="Mode" class="Bool (strict)"() -> ("Value"=w524:bool)  [unwired: 2 in, 2 out]
                n276 = call "Define Controls to Hide.vi"("Troubleshooting Mode? (f)"=w524, "Show Calibration Values? (f)"=w525, "Other Controls to Hide"=string[] ["Pause", "of", "Scan no."] ("Items to Hide"), "Measurement Information"=w522, "Hardware Parameters"=w523) -> ("Controls to Hide"=w526:string[])  [unwired: 6 in]
                n277 = call "Show and Hide Panel Controls.vi"("VI Reference In"=w521, "Operation"=w528, "Items to Hide"=w526) -> ()  [unwired: 2 in, 1 out]
              }
              frame True {
              }
            }
            n278 = Merge Errors(w502, w504) -> (w503:errorcluster)
            n279 = Select(t=w507, s=w489, f=cluster{"Enum":T8, "Data":variant}[] [{"Enum"=enum."Idle", "Data"=variant}]) -> (s? t:f=w505:cluster{"Enum":T8, "Data":variant}[])
          }
          frame #1 {
            n280 = property on="Scan?" class="Bool (strict)"("Value"=FALSE ("Visible")) -> ()  [unwired: 2 in, 2 out]
          }
        }
      }
      frame "Scan" {
        n281 = Bundle By Name(cluster=w583, "Consecutive Re-tune attempts"=0) -> (w580:T6)
        n282 = Unbundle By Name(w579) -> ("Continuous Sweeping"=w576:bool)
        n283 = case shown="True" w576 {
          tunnel: w580 -> [w591 w596]
          tunnel: [w591 w593] -> w577
          tunnel: [errorcluster {"status"=FALSE, "code"=0, "source"=""} ("error out") w592] -> w575
          tunnel: [w589 w594] -> w578
          tunnel: w579 -> [w589 w595]
          frame False {
          }
          frame True {
            n284 = call "Reverse Sweep.vi"("Hardware Parameters In"=w596, "Acquisition Parameters In"=w595) -> ("error out"=w592:errorcluster, "Hardware Parameters Out"=w593:T6, "Acquisition Parameters Out"=w594:T7)  [unwired: 7 in]
          }
        }
        n285 = call "Sweep Field and Get Data.vi"("Spectral Data In"=w588, "Hardware Parameters"=w577, "Acquisition Parameters"=w578) -> ("error out"=w582:errorcluster, "Spectral Data Out"=w586:T1)  [unwired: 2 in, 1 out]
        n286 = Merge Errors(w582, w575) -> (w581:errorcluster)
      }
      frame "Post-Scan" {
        n287 = flat-sequence {
          tunnel: w632 -> [w650]
          tunnel: w631 -> [w648]
          tunnel: w620 -> [w649]
          tunnel: [w651] -> w640
          tunnel: [w650] -> w639
          tunnel: [w648] -> w638
          tunnel: [w649] -> w637
          tunnel: w630 -> [w647]
          tunnel: [w646] -> w606
          tunnel: [w645] -> w605
          tunnel: w640 -> [w658]
          tunnel: [w658] -> w629
          tunnel: w639 -> [w655]
          tunnel: [w655] -> w627
          tunnel: w638 -> [w657]
          tunnel: [w656] -> w625
          tunnel: w637 -> [w659]
          tunnel: [w659] -> w623
          tunnel: [w653] -> w621
          tunnel: [w652] -> w611
          tunnel: w629 -> [w679]
          tunnel: [w678] -> w628
          tunnel: w627 -> [w669]
          tunnel: [w669] -> w626
          tunnel: w625 -> [w680]
          tunnel: [w680] -> w624
          tunnel: w623 -> [w674]
          tunnel: [w674] -> w622
          tunnel: w621 -> [w672]
          tunnel: [w675] -> w613
          tunnel: w611 -> [w670]
          tunnel: w628 -> [w687]
          tunnel: [w687] -> w644
          tunnel: w626 -> [w690]
          tunnel: [w690] -> w643
          tunnel: w624 -> [w689]
          tunnel: [w689] -> w642
          tunnel: w622 -> [w688]
          tunnel: [w688] -> w641
          tunnel: w613 -> [w686]
          tunnel: w644 -> [w698]
          tunnel: w643 -> [w697]
          tunnel: w642 -> [w701]
          tunnel: w641 -> [w700]
          tunnel: [w699] -> w636
          tunnel: [w697] -> w635
          tunnel: [w701] -> w634
          tunnel: [w700] -> w633
          tunnel: w636 -> [w705]
          tunnel: w635 -> [w707]
          tunnel: w634 -> [w706]
          tunnel: w633 -> [w703]
          tunnel: [w704] -> w610
          tunnel: [w707] -> w609
          tunnel: [w706] -> w608
          tunnel: [w703] -> w607
          tunnel: [w702] -> w600
          tunnel: [w721] -> w615
          tunnel: [w728] -> w616
          tunnel: [w722] -> w619
          tunnel: [w729] -> w614
          tunnel: w610 -> [w729]
          tunnel: w609 -> [w723]
          tunnel: w608 -> [w728]
          tunnel: w607 -> [w721]
          frame #0 {
            n288 = call "Append Scan Data-Rev1.vi"("Spectral Data In"=w647, "Hardware Parameters"=w648, "Acquisition Parameters"=w650) -> ("Spectral Data Out"=w651:T1, "Out-Phase Offset [v]"=w645:dbl, "In-Phase Offset [v]"=w646:dbl)  [unwired: 4 in]
          }
          frame #1 {
            n289 = Unbundle By Name(w655) -> ("Adaptive Tuning"=w654:bool)
            n290 = case shown="True" w654 {
              selector: w654 -> [w660 _]
              tunnel: w658 -> [_ w665]
              tunnel: w657 -> [w661 w664]
              tunnel: [w661 w663] -> w656
              tunnel: [w660 w662] -> w653
              frame False {
              }
              frame True {
                n291 = call "Check Tune from Data.vi"("Spectral Data In"=w665, "Hardware Parameters In"=w664) -> ("AFC Threshold Exceeded"=w668:bool, "Phase Threshold Exceeded"=w667:bool, "Balance Threshold Exceeded"=w666:bool, "Hardware Parameters Out"=w663:T6)  [unwired: 6 in]
                n292 = Compound Arithmetic op=OR(w666, w667, w668) -> (w662:bool)
              }
            }
            n293 = global read "Global Variables.vi" "Abort Scan"() -> (w652:bool)
          }
          frame #2 {
            n294 = Or(x=w672, y=w670) -> (x .or. y?=w671:bool)
            n295 = Unbundle By Name(w669) -> ("Exclude Bad Data"=w673:bool)
            n296 = case shown="True" w673 {
              tunnel: w679 -> [w681 w684]
              tunnel: [w681 w685] -> w678
              tunnel: w671 -> [_ w683]
              tunnel: w669 -> [_ w682]
              frame False {
              }
              frame True {
                n297 = call "Remove Bad Scans Spectra.vi"("Bad Scan"=w683, "Spectral Data In"=w684, "Acquisition Parameters"=w682) -> ("Spectral Data Out"=w685:T1)  [unwired: 8 in]
              }
            }
            n298 = Select(t=Save_Data_Type."Bad Scan" ("Save Data Type"), s=w671, f=Save_Data_Type."Good Scan" ("Save Data Type")) -> (s? t:f=w675:T13)
          }
          frame #3 {
            n299 = Unbundle By Name(w688) -> ("Save Data"=w691:bool)
            n300 = case shown="True" w691 {
              tunnel: w690 -> [_ w696]
              tunnel: w689 -> [_ w695]
              tunnel: w688 -> [_ w694]
              tunnel: w687 -> [_ w693]
              tunnel: w686 -> [_ w692]
              frame False {
              }
              frame True {
                n301 = call "Save EPR Data-Rev3.vi"("Save Data Type"=w692, "Spectral Data"=w693, "Measurement Information"=w694, "Hardware Parameters"=w695, "Acquisition Parameters"=w696) -> ()  [unwired: 5 in, 1 out]
              }
            }
          }
          frame #4 {
            n302 = call "Median and Average Spectra.vi"("Spectral Data In"=w698, "Acquisition Parameters In"=w697) -> ("Spectral Data Out"=w699:T1)  [unwired: 5 in]
          }
          frame #5 {
            n303 = Unbundle By Name(w705) -> ("Fit Each Scan"=w708:bool)
            n304 = case shown="True" w708 {
              tunnel: w705 -> [w710 w715]
              tunnel: w707 -> [_ w719]
              tunnel: w706 -> [_ w718]
              tunnel: [w710 w717] -> w704
              tunnel: w703 -> [_ w714]
              tunnel: [_ w713] -> w702
              frame False {
                n305 = property on="Fit Pars and Labels" class="Clust (strict)"("Value"=cluster{"Pars Labels":string[], "pars":dbl[]} {"Pars Labels"=[], "pars"=[]} ("Fit Pars and Labels")) -> ()  [unwired: 2 in, 2 out]
              }
              frame True {
                n306 = call "Fit EPR Spectra (QSM)-Rev2.vi"("Spectral Data In"=w715, "Measurement Information"=w714, "Hardware Parameters In"=w718, "Acquisition Parameters In"=w719) -> ("Fit Pars and Labels"=w716:cluster{"Pars Labels":string[], "pars":dbl[]}, "Spectral Data Out"=w717:T1, "Number of Fit Iterations"=w712:i32, "error out"=w713:errorcluster, "Global SNR"=w711:dbl)  [unwired: 3 in]
                n307 = property on="Number of Fit Iterations" class="DigNum (strict)"("Value"=w712) -> ()  [unwired: 2 in, 2 out]
                n308 = property on="Fit Pars and Labels" class="Clust (strict)"("Value"=w716) -> ()  [unwired: 2 in, 2 out]
                n309 = property on="In-Phase SNR" class="DigNum (strict)"("Value"=w711) -> ()  [unwired: 2 in, 2 out]
              }
            }
          }
          frame #6 {
            n310 = property on="Scan no." class="DigNum (strict)"() -> ("Value"=w727:u32)  [unwired: 2 in, 2 out]
            n311 = Increment(x=w727) -> (x+1=w726:u32)
            n312 = property on="Scan no." class="DigNum (strict)"("Value"=w726) -> ()  [unwired: 2 in, 2 out]
            n313 = property on="No. Scans/Set" class="DigNum (strict)"() -> ("Value"=w725:u32)  [unwired: 2 in, 2 out]
            n314 = call "Increment Scan Counters.vi"("Measurement Information"=w721, "Acquisition Parameters In"=w723) -> ("Scans Completed"=w720:u32, "Acquisition Parameters Out"=w722:T7)  [unwired: 8 in]
            n315 = Divide(x=w720, y=w725) -> (x/y=w724:dbl)
            n316 = property on="Set Progress" class="Slide (strict)"("Value"=w724) -> ()  [unwired: 2 in, 2 out]
          }
        }
        n317 = property on="Out Phase Offset" class="DigNum (strict)"("Value"=w605) -> ()  [unwired: 2 in, 2 out]
        n318 = property on="In Phase Offset" class="DigNum (strict)"("Value"=w606) -> ()  [unwired: 2 in, 2 out]
        n319 = call "In-Context Exit Scan-Rev5.vi"("Acquisition Parameters In"=w619, "Hardware Parameters In"=w616, "Measurement Information In"=w615, "Spectral Data In"=w614) -> ("Linewidth (HWHM)/Scan [Gauss] Out"=w604:dbl[][], "Exclude pO2 Estimate"=w597:bool, "Acquisition Parameters Out"=w612:T7, "Measurement Information Out"=w618:T3, "Spectral Data Out"=w601:T1, "pO2/Scan [mmHg] Out"=w603:dbl[][], "error out"=w599:errorcluster, "pO2 [mmHg]"=w602:dbl[], "QSM Response"=w617:cluster{"Enum":T8, "Data":variant}[])  [unwired: 2 in, 1 out]
        n320 = Merge Errors(w599, w600) -> (w598:errorcluster)
        n321 = property on="Unacceptable pO2 Estimate" class="Bool (strict)"("Value"=w597) -> ()  [unwired: 2 in, 2 out]
        n322 = property on="Linewidth (HWHM) [Gauss]" class="WFGraph (strict)"("Value"=w604) -> ()  [unwired: 2 in, 2 out]
        n323 = property on="pO2 [mmHg]" class="Arr (strict)"("Value"=w602) -> ()  [unwired: 2 in, 2 out]
        n324 = property on="pO2/Scan [mmHg]" class="WFGraph (strict)"("Value"=w603) -> ()  [unwired: 2 in, 2 out]
        n325 = call "Update Plots for Spectra Graph.vi"("Spectral Data"=w601, "Acquisition Parameters"=w612) -> ()
      }
      frame "Exit Set" {
        w774 = u16 0 items=["Hide", "Show"] ("Operation")
        n326 = property on="Show Calibration Constants" class="Bool (strict)"() -> ("Value"=w769:bool)  [unwired: 2 in, 2 out]
        n327 = property on="Mode" class="Bool (strict)"() -> ("Value"=w768:bool)  [unwired: 2 in, 2 out]
        n328 = call "Fit EPR Spectra (QSM)-Rev2.vi"("Spectral Data In"=w770, "Measurement Information"=w737, "Hardware Parameters In"=w751, "Acquisition Parameters In"=w733) -> ("Fit Pars and Labels"=w777:cluster{"Pars Labels":string[], "pars":dbl[]}, "Spectral Data Out"=w736:T1, "Number of Fit Iterations"=w735:i32, "error out"=w744:errorcluster, "Global SNR"=w730:dbl)  [unwired: 3 in]
        n329 = call "Define Controls to Hide.vi"("Troubleshooting Mode? (f)"=w768, "Show Calibration Values? (f)"=w769, "Other Controls to Hide"=string[] ["Pause", "of", "Scan no."] ("Items to Hide"), "Measurement Information"=w737, "Hardware Parameters"=w751) -> ("Controls to Hide"=w772:string[])  [unwired: 6 in]
        n330 = call "Show and Hide Panel Controls.vi"("VI Reference In"=w784, "Operation"=w774, "Items to Hide"=w772) -> ()  [unwired: 2 in, 1 out]
        n331 = property on="Number of Fit Iterations" class="DigNum (strict)"("Value"=w735) -> ()  [unwired: 2 in, 2 out]
        n332 = property on="Fit Pars and Labels" class="Clust (strict)"("Value"=w777) -> ()  [unwired: 2 in, 2 out]
        n333 = property on="In-Phase SNR" class="DigNum (strict)"("Value"=w730) -> ()  [unwired: 2 in, 2 out]
        n334 = property on="Set Progress" class="Slide (strict)"("Fill Color"=u32 6618880) -> ()  [unwired: 2 in, 2 out]
        n335 = property on="Scan?" class="Bool (strict)"("Value"=FALSE ("Pause Parallel DAQ")) -> ()  [unwired: 2 in, 2 out]
        n336 = global write "Global Variables.vi" "Pause Parallel DAQ"(FALSE ("Pause Parallel DAQ")) -> ()
        n337 = global write "Global Variables.vi" "Finished scanning?"(TRUE ("Finished scanning?")) -> ()
        n338 = Unbundle By Name(w737) -> ("Save Data"=w753:bool)
        n339 = case shown="True" w753 {
          tunnel: w733 -> [_ w811]
          tunnel: w751 -> [_ w810]
          tunnel: w737 -> [_ w809]
          tunnel: w736 -> [_ w808]
          frame False {
          }
          frame True {
            n340 = call "Save EPR Data-Rev3.vi"("Save Data Type"=Save_Data_Type."Median", "Spectral Data"=w808, "Measurement Information"=w809, "Hardware Parameters"=w810, "Acquisition Parameters"=w811) -> ()  [unwired: 5 in, 1 out]
          }
        }
        n341 = Unbundle By Name(w733) -> ("AFC Field Correction"=w752:bool)
        n342 = Unbundle By Name(w733) -> ("Scan Width [G]"=w732:dbl, "Mod. Amp. [G]"=w731:dbl)
        n343 = Unbundle By Name(w736) -> ("PDT Amp [v]"=w776:dbl, "RIS Amp [v]"=w775:dbl)
        n344 = Unbundle By Name(w737) -> ("Save Data"=w749:bool)
        n345 = property on="Previous Scan range (Gauss)" class="DigNum (strict)"("Value"=w732) -> ()  [unwired: 2 in, 2 out]
        n346 = property on="Previous Mod. Amp. (Gauss)" class="DigNum (strict)"("Value"=w731) -> ()  [unwired: 2 in, 2 out]
        n347 = property on="PDT Amp p-p" class="DigNum (strict)"("Value"=w776) -> ()  [unwired: 2 in, 2 out]
        n348 = property on="Tooth Amp P-P" class="DigNum (strict)"("Value"=w775) -> ()  [unwired: 2 in, 2 out]
        n349 = And(x=w749, y=w752) -> (x .and. y?=w750:bool)
        n350 = case shown="True" w750 {
          tunnel: w733 -> [_ w789]
          tunnel: w751 -> [_ w788]
          tunnel: w737 -> [_ w787]
          tunnel: w736 -> [_ w786]
          frame False {
          }
          frame True {
            n351 = call "Save EPR Data-Rev3.vi"("Save Data Type"=Save_Data_Type."Appended Scans", "Spectral Data"=w786, "Measurement Information"=w787, "Hardware Parameters"=w788, "Acquisition Parameters"=w789) -> ()  [unwired: 5 in, 1 out]
          }
        }
        n352 = Unbundle By Name(w733) -> ("Acquire Photos"=w748:bool)
        n353 = Unbundle By Name(w737) -> ("Save Data"=w747:bool)
        n354 = And(x=w747, y=w748) -> (x .and. y?=w778:bool)
        n355 = case shown="True" w778 {
          tunnel: w751 -> [_ w804]
          tunnel: w737 -> [_ w803]
          tunnel: w736 -> [_ w806]
          tunnel: w733 -> [_ w805]
          tunnel: [errorcluster {"status"=FALSE, "code"=0, "source"=""} ("error out") _] -> w760
          frame False {
          }
          frame True {
            # "0.2.5.14 - Removed\nCamera Grab_AG.vi"
            n356 = call "Save EPR Data-Rev3.vi"("Save Data Type"=Save_Data_Type."Filename", "Spectral Data"=w806, "Measurement Information"=w803, "Hardware Parameters"=w804, "Acquisition Parameters"=w805) -> ()  [unwired: 5 in, 1 out]
          }
        }
        n357 = call "Update Plots for Spectra Graph.vi"("Spectral Data"=w736, "Acquisition Parameters"=w733) -> ()
        n358 = Unbundle By Name(w733) -> ("Continuous Sweeping"=w757:bool)
        n359 = case shown="True" w757 {
          tunnel: w733 -> [w790 w796]
          tunnel: w751 -> [w791 w795]
          tunnel: [w791 w793] -> w756
          tunnel: [_ w792] -> w759
          tunnel: [w790 w794] -> w755
          frame False {
          }
          frame True {
            n360 = call "Return Original Field.vi"("Hardware Parameters In"=w795, "Acquisition Parameters In"=w796) -> ("error out"=w792:errorcluster, "Hardware Parameters Out"=w793:T6, "Acquisition Parameters Out"=w794:T7)  [unwired: 7 in]
          }
        }
        n361 = call "In-Context Exit Set Actions-Rev5.vi"("Acquisition Parameters In"=w755, "Hardware Parameters In"=w756, "Measurement Information In"=w737, "Spectral Data In"=w736) -> ("Exclude pO2 Estimate"=w734:bool, "Scan Width [G]"=w742:dbl, "Mod. Amp. [G]"=w743:dbl, "Acquisition Parameters Out"=w746:T7, "Measurement Information Out"=w740:T3, "Spectral Data Out"=w763:T1, "QSM Response"=w762:cluster{"Enum":T8, "Data":variant}[], "Magnet Angle [deg]"=w741:dbl, "Calibration dBpp/Set [Gauss]"=w738:dbl[][], "pO2/Set [mmHg]"=w739:dbl[][], "error out"=w761:errorcluster)  [unwired: 1 in]
        n362 = call "Zero Sweep.vi"("error in (no error)"=w759) -> ("error out"=w758:errorcluster)  [unwired: 10 in]
        n363 = property on="Scan range (Gauss)" class="DigNum (strict)"("Value"=w742) -> ()  [unwired: 2 in, 2 out]
        n364 = property on="Mod. Amp. (Gauss)" class="DigNum (strict)"("Value"=w743) -> ()  [unwired: 2 in, 2 out]
        n365 = property on="pO2/Set [mmHg]" class="WFGraph (strict)"("Value"=w739) -> ()  [unwired: 2 in, 2 out]
        n366 = property on="Linewidth (HWHM)/Set [Gauss]" class="WFGraph (strict)"("Value"=w738) -> ()  [unwired: 2 in, 2 out]
        n367 = property on="Magnet Angle (deg)" class="DigNum (strict)"("Value"=w741) -> ()  [unwired: 2 in, 2 out]
        n368 = property on="Unacceptable pO2 Estimate" class="Bool (strict)"("Value"=w734) -> ()  [unwired: 2 in, 2 out]
        n369 = Merge Errors(w761, w758, w760, w744) -> (w782:errorcluster)
        n370 = global read "Global Variables.vi" "Abort Scan"() -> (w745:bool)
        n371 = Unbundle By Name(w746) -> ("Running Script"=w767:bool)
        n372 = Unbundle By Name(w740) -> ("Save Data"=w781:bool)
        n373 = case shown="True" w781 {
          tunnel: [w812 w816] -> w783
          tunnel: w740 -> [w812 w813]
          frame False {
          }
          frame True {
            n374 = Unbundle By Name(w813) -> ("Set #"=w814:u32)
            n375 = Increment(x=w814) -> (x+1=w815:u32)
            n376 = Bundle By Name(cluster=w813, "Set #"=w815) -> (w816:T3)
            n377 = property on="Sets Completed" class="DigNum (strict)"("Value"=w814) -> ()  [unwired: 2 in, 2 out]
          }
        }
        n378 = case shown="True" w745 {
          selector: w745 -> [_ w798]
          tunnel: [FALSE ("Abort Scan") FALSE ("Abort Scan")] -> w771
          frame False {
          }
          frame True {
            n379 = global write "Global Variables.vi" "Abort QA"(w798) -> ()
            n380 = One Button Dialog(message="Measurement aborted") -> ()  [unwired: 1 in, 1 out]
          }
        }
        n381 = global write "Global Variables.vi" "Abort Scan"(w771) -> ()
        n382 = Select(t=cluster{"Enum":T8, "Data":variant}[] [{"Enum"=enum."Read from Script", "Data"=variant}], s=w767, f=w762) -> (s? t:f=w766:cluster{"Enum":T8, "Data":variant}[])
      }
      frame "Automated Tuning" {
        n383 = Unbundle By Name(w818) -> ("Lock-in OK?"=w821:bool, "Ignore Lock-in Comm. Failure"=w820:bool)
        n384 = Or(x=w821, y=w820) -> (x .or. y?=w819:bool)
        n385 = case shown="True" w819 {
          tunnel: [w833 w853] -> w828
          tunnel: w818 -> [w833 w852]
          tunnel: w827 -> [w834 w851]
          tunnel: w826 -> [w832 w850]
          tunnel: w825 -> [w831 w849]
          tunnel: [w831 w848] -> w824
          tunnel: [w832 w847] -> w823
          tunnel: [w834 w846] -> w822
          tunnel: [errorcluster {"status"=FALSE, "code"=0, "source"=""} ("error out") w836] -> w817
          frame False {
            n386 = One Button Dialog(message="Unable to communicate with Lock In.\nCannot perform automated tuning.") -> ()  [unwired: 1 in, 1 out]
            n387 = property on="Auto-Tune" class="Bool (strict)"("Value"=FALSE ("Auto-Tune")) -> ()  [unwired: 2 in, 2 out]
          }
          frame True {
            n388 = flat-sequence {
              tunnel: w849 -> [w860]
              tunnel: w850 -> [w861]
              tunnel: w851 -> [w862]
              tunnel: w852 -> [w863]
              tunnel: [w863] -> w845
              tunnel: [w862] -> w844
              tunnel: [w861] -> w843
              tunnel: [w860] -> w842
              tunnel: [w858] -> w837
              tunnel: [w875] -> w857
              tunnel: [w869] -> w856
              tunnel: [w868] -> w855
              tunnel: [w867] -> w854
              tunnel: w845 -> [w866]
              tunnel: w844 -> [w869]
              tunnel: w843 -> [w868]
              tunnel: w842 -> [w867]
              tunnel: w837 -> [w864]
              tunnel: w857 -> [w901]
              tunnel: w856 -> [w904]
              tunnel: w855 -> [w903]
              tunnel: w854 -> [w902]
              tunnel: [w900] -> w841
              tunnel: [w904] -> w840
              tunnel: [w903] -> w839
              tunnel: [w902] -> w838
              tunnel: [w898] -> w836
              tunnel: [w907] -> w848
              tunnel: [w908] -> w847
              tunnel: [w909] -> w846
              tunnel: [w910] -> w853
              tunnel: w841 -> [w910]
              tunnel: w840 -> [w909]
              tunnel: w839 -> [w908]
              tunnel: w838 -> [w907]
              frame #0 {
                n389 = global read "Global Variables.vi" "Finished scanning?"() -> (w858:bool)
                n390 = global write "Global Variables.vi" "Pause Parallel DAQ"(TRUE ("Stop(QSM)")) -> ()
              }
              frame #1 {
                n391 = case shown="False" w864 {
                  tunnel: w866 -> [w877 w880]
                  tunnel: [w876 w880] -> w865
                  frame False {
                    n392 = Unbundle By Name(w877) -> ("Consecutive Re-tune attempts"=w878:i32)
                    n393 = Increment(x=w878) -> (x+1=w879:i32)
                    n394 = Bundle By Name(cluster=w877, "Consecutive Re-tune attempts"=w879) -> (w876:T6)
                  }
                  frame True {
                  }
                }
                n395 = property on="Auto-Tune" class="Bool (strict)"() -> ("Value"=w873:bool)  [unwired: 2 in, 2 out]
                n396 = case shown="False" w873 {
                  tunnel: w866 -> [w886 _]
                  tunnel: [w885 w888] -> w872
                  tunnel: [w883 w888] -> w871
                  tunnel: [w882 w888] -> w870
                  frame False {
                    n397 = Unbundle By Name(w886) -> ("Balance Threshold Exceeded?"=w881:bool, "AFC Threshold Exceeded?"=w884:bool, "Phase Threshold Exceeded?"=w885:bool)
                    n398 = Not(x=w881) -> (.not. x?=w882:bool)
                    n399 = Or(x=w881, y=w884) -> (x .or. y?=w883:bool)
                  }
                  frame True {
                    w888 = TRUE ("Phase Threshold Exceeded?")
                    n400 = property on="Auto-Tune" class="Bool (strict)"("Value"=FALSE ("Auto-Tune")) -> ()  [unwired: 2 in, 2 out]
                  }
                }
                n401 = case shown="True" w871 {
                  tunnel: w865 -> [w889 w893]
                  tunnel: [w889 w892] -> w874
                  tunnel: w870 -> [_ w890]
                  frame False {
                  }
                  frame True {
                    n402 = call "Network Analyzer and Frequency Tune.vi"("FTUNE(ON)/NETA(OFF)"=w890, "Hardware Parameters In"=w893) -> ("Voltage Output"=w891:dbl, "Hardware Parameters Out"=w892:T6)  [unwired: 5 in]
                    n403 = property on="Frequency Voltage" class="DigNum (strict)"("Value"=w891) -> ()  [unwired: 2 in, 2 out]
                  }
                }
                n404 = case shown="True" w872 {
                  tunnel: w874 -> [w894 w897]
                  tunnel: [w894 w896] -> w875
                  frame False {
                  }
                  frame True {
                    n405 = call "Phase Tune.vi"("Hardware Parameters"=w897) -> ("Phase Voltage [v]"=w895:dbl, "Hardware Parameters Out"=w896:T6)  [unwired: 8 in, 1 out]
                    n406 = property on="Phase Voltage" class="DigNum (strict)"("Value"=w895) -> ()  [unwired: 2 in, 2 out]
                  }
                }
              }
              frame #2 {
                n407 = call "Check Current Tune.vi"("Time to collect [ms]"=100, "Hardware Parameters"=w901) -> ("Hardware Parameters Out"=w900:T6, "error out"=w898:errorcluster)  [unwired: 5 in, 3 out]
              }
              frame #3 {
                n408 = global write "Global Variables.vi" "Pause Parallel DAQ"(FALSE ("Stop(QSM)")) -> ()
                n409 = Wait Until Next ms Multiple(millisecond multiple=u32 50) -> ()  [unwired: 1 out]
              }
            }
          }
        }
      }
      frame "Manual Tuning" {
        n410 = property on="Manual Tuning" class="Bool (strict)"("Value"=FALSE ("Manual Tuning")) -> ()  [unwired: 2 in, 2 out]
        n411 = flat-sequence {
          tunnel: w925 -> [w931]
          tunnel: w926 -> [w932]
          tunnel: w927 -> [w933]
          tunnel: w928 -> [w934]
          tunnel: [w934] -> w924
          tunnel: [w933] -> w923
          tunnel: [w932] -> w922
          tunnel: [w931] -> w921
          tunnel: [w938] -> w919
          tunnel: [w937] -> w917
          tunnel: [w936] -> w915
          tunnel: [w935] -> w913
          tunnel: w924 -> [w937]
          tunnel: w923 -> [w938]
          tunnel: w922 -> [w936]
          tunnel: w921 -> [w935]
          tunnel: w919 -> [w949]
          tunnel: [w949] -> w918
          tunnel: w917 -> [w944]
          tunnel: [w943] -> w916
          tunnel: w915 -> [w948]
          tunnel: [w948] -> w914
          tunnel: w913 -> [w947]
          tunnel: [w947] -> w912
          tunnel: [w951] -> _
          tunnel: [w952] -> _
          tunnel: [w953] -> w920
          tunnel: [w954] -> _
          tunnel: w918 -> [w954]
          tunnel: w916 -> [w953]
          tunnel: w914 -> [w952]
          tunnel: w912 -> [w951]
          frame #0 {
            n412 = global write "Global Variables.vi" "Pause Parallel DAQ"(TRUE ("Pause Parallel DAQ")) -> ()
          }
          frame #1 {
            n413 = Unbundle By Name(w937) -> ("Lock-in OK?"=w941:bool, "Ignore Lock-in Comm. Failure"=w940:bool)
            n414 = Or(x=w941, y=w940) -> (x .or. y?=w939:bool)
            n415 = case shown="True" w939 {
              frame False {
                n416 = One Button Dialog(message="Unable to communicate with Lock In.\nAFC may or may not be on while coupling.") -> ()  [unwired: 1 in, 1 out]
              }
              frame True {
              }
            }
          }
          frame #2 {
            n417 = call "Network Analyzer and Frequency Tune.vi"("FTUNE(ON)/NETA(OFF)"=FALSE, "Hardware Parameters In"=w944) -> ("Voltage Output"=w946:dbl, "Hardware Parameters Out"=w943:T6)  [unwired: 5 in]
            n418 = property on="Frequency Voltage" class="DigNum (strict)"("Value"=w946) -> ()  [unwired: 2 in, 2 out]
          }
          frame #3 {
            n419 = global write "Global Variables.vi" "Pause Parallel DAQ"(FALSE ("Pause Parallel DAQ")) -> ()
          }
        }
      }
      frame "Check Calibration" {
        w956 = Fitting_Model_Selection."PDTCalibration" ("Model Select")
        # "Store and restore original values"
        n420 = Bundle By Name(cluster=w967, "Save Data"=FALSE) -> (w960:T3)
        n421 = property on="Calibrate" class="Bool (strict)"("Value"=FALSE ("Calibrate")) -> ()  [unwired: 2 in, 2 out]
        n422 = Bundle By Name(cluster=w966, "Model Select"=w956) -> (w964:T1)
        n423 = property on="Model Select" class="Enum (strict)"("Value"=w956) -> ()  [unwired: 2 in, 2 out]
        n424 = Unbundle By Name(w958) -> ("First CheckCal Scan?"=w957:bool)
        n425 = case shown="False" w957 {
          tunnel: w967 -> [_ w1014]
          tunnel: [w976 w1013] -> w965
          tunnel: w958 -> [w974 w1012]
          tunnel: w962 -> [w981 w1011]
          tunnel: w960 -> [w980 w1004]
          tunnel: w964 -> [w979 _]
          tunnel: [w975 w1011] -> w961
          tunnel: [w977 w1003] -> w959
          tunnel: [w978 _] -> w963
          frame False {
            n426 = flat-sequence {
              tunnel: w981 -> [w993]
              tunnel: w980 -> [w992]
              tunnel: w979 -> [w991]
              tunnel: w974 -> [w983]
              tunnel: [w990] -> w973
              tunnel: [w989] -> w972
              tunnel: [w987] -> w971
              tunnel: [w986] -> w970
              tunnel: [w998] -> w975
              tunnel: [w999] -> w976
              tunnel: [w1000] -> w977
              tunnel: [w1001] -> w978
              tunnel: w973 -> [w1001]
              tunnel: w972 -> [w1000]
              tunnel: w971 -> [w999]
              tunnel: w970 -> [w998]
              frame #0 {
                n427 = call "Check Calibration.vi"("Spectral Data In"=w991, "Measurement Information In"=w992, "Hardware Parameters In"=w993, "Acquisition Parameters In"=w983) -> ("QSM Action"=w990:cluster{"Enum":T8, "Data":variant}[], "Measurement Information Out"=w989:T3, "Hardware Parameters Out"=w986:T6, "Acquisition Parameters Out"=w987:T7)  [unwired: 4 in]
                n428 = Unbundle By Name(w986) -> ("Scan Calibration [G/V]"=w985:dbl, "Modulation Calibration [G/V]"=w984:dbl)
                n429 = Unbundle By Name(w987) -> ("Central Field [G]"=w988:dbl)
                n430 = property on="Central field (Gauss)" class="DigNum (strict)"("Value"=w988) -> ()  [unwired: 2 in, 2 out]
                n431 = property on="Scan Gauss/V" class="DigNum (strict)"("Value"=w985) -> ()  [unwired: 2 in, 2 out]
                n432 = property on="Mod. Gauss/Vrms" class="DigNum (strict)"("Value"=w984) -> ()  [unwired: 2 in, 2 out]
                n433 = property on="Scan range (Gauss)" class="DigNum (strict)"("Value"=25.0 ("Scan range (Gauss)")) -> ()  [unwired: 2 in, 2 out]
              }
              frame #1 {
                n434 = call-poly "Get Config Key.vi"("default value"=u32 10, "key"="scans_set", "section"="acquisition") -> ("value"=w994:u32)  [unwired: 7 in, 1 out]
                n435 = property on="No. Scans/Set" class="DigNum (strict)"("Value"=w994) -> ()  [unwired: 2 in, 2 out]
              }
            }
          }
          frame True {
            n436 = Unbundle By Name(w1014) -> ("DAQ Mode"=w1015:enum16{"Engineering", "Dosimetry", "Oximetry"})
            n437 = Equal?(x=w1015, y=enum16{"Engineering", "Dosimetry", "Oximetry"}."Dosimetry" ("DAQ Mode")) -> (x = y?=w1017:bool)
            n438 = case shown="True" w1017 {
              tunnel: [40.0 ("Scan Width [G]") 50.0 ("Scan Width [G]")] -> w1009
              tunnel: [w1022 4.0 ("Mod. Amp. [G]")] -> w1008
              tunnel: [w1021 0.0 ("Central Field [G]")] -> w1007
              tunnel: [w1020 u32 3 ("No. Scans/Set")] -> w1006
              frame False {
                n439 = One Button Dialog(message="Please ensure the PDT and resonator is centered within the magnet. ") -> ()  [unwired: 1 in, 1 out]
                n440 = property on="Mod. Amp. (Gauss)" class="DigNum (strict)"() -> ("Value"=w1022:dbl)  [unwired: 2 in, 2 out]
                n441 = property on="Central field (Gauss)" class="DigNum (strict)"() -> ("Value"=w1021:dbl)  [unwired: 2 in, 2 out]
                n442 = property on="No. Scans/Set" class="DigNum (strict)"() -> ("Value"=w1020:u32)  [unwired: 2 in, 2 out]
              }
              frame True {
                n443 = One Button Dialog(message="Please fasten the BallZero in the magnet,\nturn on the Kepco Sweep Amplifier,\nplace the resonator on the BallZero, and\nclick the OK button to continue.") -> ()  [unwired: 1 in, 1 out]
              }
            }
            n444 = Bundle By Name(cluster=w1004, "QA Mode"=T14."Check Calibration", "QA Session?"=TRUE) -> (w1003:T3)
            n445 = Bundle By Name(cluster=w1012, "First CheckCal Scan?"=FALSE ("First Check Calibration Scan"), "Scan Width [G]"=w1009, "Mod. Amp. [G]"=w1008, "Central Field [G]"=w1007, "No. Scans/Set"=w1006) -> (w1013:T7)
            n446 = property on="Scan range (Gauss)" class="DigNum (strict)"("Value"=w1009) -> ()  [unwired: 2 in, 2 out]
            n447 = property on="Mod. Amp. (Gauss)" class="DigNum (strict)"("Value"=w1008) -> ()  [unwired: 2 in, 2 out]
            n448 = property on="Central field (Gauss)" class="DigNum (strict)"("Value"=w1007) -> ()  [unwired: 2 in, 2 out]
            n449 = property on="No. Scans/Set" class="DigNum (strict)"("Value"=w1006) -> ()  [unwired: 2 in, 2 out]
          }
        }
      }
      frame "Optimize RF Power" {
        # "Insert this into its own VI"
        # "Lock-in needs to be okay for this, as it changes the attenuator on the bridge, which is controlled via the digital output port of the lock-in"
        n450 = Unbundle By Name(w1033) -> ("Lock-in OK?"=w1030:bool, "Ignore Lock-in Comm. Failure"=w1029:bool)
        n451 = property on="Optimize RF Power" class="Bool (strict)"("Value"=FALSE ("Optimize RF Power")) -> ()  [unwired: 2 in, 2 out]
        n452 = Or(x=w1030, y=w1029) -> (x .or. y?=w1031:bool)
        n453 = case shown="True" w1031 {
          tunnel: w1038 -> [_ w1056]
          tunnel: w1037 -> [w1042 w1053]
          tunnel: [_ w1052] -> w1039
          tunnel: w1035 -> [w1043 w1051]
          tunnel: w1038 -> [_ w1050]
          tunnel: [w1042 w1049] -> w1036
          tunnel: [w1043 w1048] -> w1034
          tunnel: w1033 -> [w1041 w1047]
          tunnel: [w1041 w1046] -> w1032
          tunnel: [_ w1045] -> w1028
          frame False {
            n454 = One Button Dialog(message="Unable to communicate with Lock In.\nCannot perform RF Power Optimization") -> ()  [unwired: 1 in, 1 out]
          }
          frame True {
            # "Need to have at least one good spectra to know where the peak is before optimizing the RF power."
            n455 = Unbundle By Name(w1056) -> ("Fit Spectra"=w1055:dbl[])
            n456 = Empty Array?(array=w1055) -> (empty?=w1054:bool)
            n457 = case shown="False" w1054 {
              tunnel: w1053 -> [w1065 w1104]
              tunnel: [w1064 _] -> w1052
              tunnel: w1051 -> [w1063 w1105]
              tunnel: w1050 -> [w1062 _]
              tunnel: [w1061 w1104] -> w1049
              tunnel: [w1060 w1105] -> w1048
              tunnel: w1047 -> [w1059 w1103]
              tunnel: [w1058 w1103] -> w1046
              tunnel: [w1057 _] -> w1045
              frame False {
                # "Need to setup n-scans (as dictated by GUI) with high mod amp to broaden out potentially narrow peaks. This flag is only written to within this boolean case structure."
                n458 = Unbundle By Name(w1065) -> ("Optimizing RF Power"=w1066:bool)
                n459 = case shown="False" w1066 {
                  tunnel: w1065 -> [w1073 w1101]
                  tunnel: [cluster{"Enum":T8, "Data":variant}[] [{"Enum"=enum."Configure Hardware", "Data"=variant}, {"Enum"=enum."Initialize Set", "Data"=variant}, {"Enum"=enum."Pre-Scan", "Data"=variant}] _] -> w1064
                  tunnel: w1063 -> [w1080 w1099]
                  tunnel: w1062 -> [w1072 w1096]
                  tunnel: [w1070 w1100] -> w1061
                  tunnel: [w1069 w1099] -> w1060
                  tunnel: w1059 -> [w1068 w1098]
                  tunnel: [w1068 w1097] -> w1058
                  tunnel: [_ w1092] -> w1057
                  frame False {
                    # "Consider having another check to make sure that either single LiPc or ink model is chosen"
                    # "Find minimum linewidth, and set scan/mod from it"
                    n460 = Unbundle By Name(w1072) -> ("Model Select"=w1089:T2, "Fit Pars"=w1088:dbl[])
                    n461 = Bundle By Name(cluster=w1073, "Optimizing RF Power"=TRUE) -> (w1071:T7)
                    n462 = Bundle By Name(cluster=w1080, "Save Data"=FALSE) -> (w1069:T3)
                    n463 = Index Array(array=w1088, index #1=6 ("index"), index #2=9 ("index")) -> (element #1=w1085:dbl, element #2=w1084:dbl)
                    n464 = Build Array(w1085, w1084) -> (w1083:dbl[])
                    n465 = Array Max & Min(array=w1083) -> (min value=w1082:dbl)  [unwired: 3 out]
                    n466 = Equal?(x=w1089, y=Fitting_Model_Selection."LiPc") -> (x = y?=w1090:bool)
                    n467 = Select(t=w1085, s=w1090, f=w1082) -> (s? t:f=w1076:dbl)
                    n468 = Multiply(x=2.0, y=w1076) -> (x*y=w1074:dbl)
                    n469 = Multiply(x=w1076, y=10.0) -> (x*y=w1077:dbl)
                    n470 = Bundle By Name(cluster=w1071, "Mod. Amp. [G]"=w1074, "Scan Width [G]"=w1077) -> (w1070:T7)
                  }
                  frame True {
                    # "Run power optimizing routine"
                    n471 = Bundle By Name(cluster=w1101, "Optimizing RF Power"=FALSE) -> (w1100:T7)
                    n472 = call "Optimize RF Power.vi"("Spectral Data In"=w1096, "Hardware Parameters In"=w1098) -> ("Resultant Attenuation [dB]"=w1095:u16, "MC error out"=w1093:errorcluster, "Lock-in error out"=w1094:errorcluster, "Hardware Parameters Out"=w1097:T6)  [unwired: 4 in]
                    n473 = Merge Errors(w1094, w1093) -> (w1092:errorcluster)
                    n474 = property on="Attenuation/dB" class="DigNum (strict)"("Value"=w1095) -> ()  [unwired: 2 in, 2 out]
                  }
                }
              }
              frame True {
                n475 = One Button Dialog(message="Please collect at least one scan with an EPR signal") -> ()  [unwired: 1 in, 1 out]
              }
            }
          }
        }
      }
      frame "Test Scan" {
        n476 = Bundle By Name(cluster=w1112, "Save Data"=FALSE) -> (w1111:T3)
        n477 = Bundle By Name(cluster=w1109, "No. Scans/Set"=u32 1) -> (w1108:T7)
        n478 = property on="Single Test Scan" class="Bool (strict)"("Value"=FALSE ("Single Test Scan")) -> ()  [unwired: 2 in, 2 out]
      }
      frame "Set Oxy QA-Scan Pars" {
        n479 = Unbundle By Name(w1117) -> ("Scan Width [G]"=w1119:dbl, "Mod. Amp. [G]"=w1118:dbl)
        n480 = Bundle By Name(cluster=w1117, "Mod. Amp. [G]"=1.0 ("Mod. Amp. (Gauss)"), "Scan Width [G]"=40.0 ("Scan range (Gauss)"), "Oxy QA Scan?"=TRUE, "OxyQAInit Scan Width [G]"=w1119, "OxyQAInit Mod. Amp. [G]"=w1118) -> (w1123:T7)
        n481 = property on="Collect QA Scan" class="Bool (strict)"("Value"=FALSE ("Collect QA Scan")) -> ()  [unwired: 2 in, 2 out]
      }
      frame "Find Peaks" {
        n482 = Unbundle By Name(w1131) -> ("AFC Field Correction"=w1130:bool, "Exclude Bad Data"=w1129:bool)
        n483 = property on="Find Peaks" class="Bool (strict)"("Value"=FALSE ("Find Peaks")) -> ()  [unwired: 2 in, 2 out]
        n484 = case shown="True" w1130 {
          tunnel: w1148 -> [w1155 w1165]
          tunnel: [w1154 w1159] -> w1139
          tunnel: [w1153 w1158] -> w1138
          tunnel: w1129 -> [_ w1164]
          frame False {
            n485 = Unbundle By Name(w1155) -> ("In-Phase Median Spectra"=w1154:dbl[], "B-Field"=w1153:dbl[])
          }
          frame True {
            n486 = Unbundle By Name(w1165) -> ("Good Shifted B-Fields"=w1161:dbl[][], "All Shifted B-Fields"=w1160:dbl[][], "Good In-Phase Scan Spectra"=w1163:dbl[][], "All In-Phase Scan Spectra"=w1162:dbl[][])
            n487 = Select(t=w1161, s=w1164, f=w1160) -> (s? t:f=w1157:dbl[][])
            n488 = Select(t=w1163, s=w1164, f=w1162) -> (s? t:f=w1156:dbl[][])
            n489 = call "Flatten EPR and B-Field Arrays.vi"("2D EPR Data"=w1156, "2D B-Fields"=w1157) -> ("1D Flattened EPR Data"=w1158:dbl[], "1D Flattened B-Fields"=w1159:dbl[])
          }
        }
        n490 = property on="Spectra Graph" class="XYGraph (strict)"() -> ("CrsrList"=w1147:T15)  [unwired: 2 in, 2 out]
        n491 = Array Max & Min(array=w1139) -> (max value=w1133:dbl, max index (indices)=w1137:i32, min value=w1132:dbl, min index (indices)=w1136:i32)
        n492 = Index Array(array=w1138, index #1=w1137, index #2=w1136) -> (element #1=w1135:dbl, element #2=w1134:dbl)
        n493 = Index Array(array=w1147, index #1=0 ("index"), index #2=1 ("index")) -> (element #1=w1144:T16, element #2=w1143:T16)
        n494 = Bundle By Name(cluster=w1144, "Position.X"=w1135, "Position.Y"=w1133) -> (w1142:T16)
        n495 = Bundle By Name(cluster=w1143, "Position.X"=w1134, "Position.Y"=w1132) -> (w1141:T16)
        n496 = Build Array(w1142, w1141) -> (w1140:T17)
        n497 = property on="Spectra Graph" class="XYGraph (strict)"("CrsrList"=w1140) -> ()  [unwired: 2 in, 2 out]
      }
      frame "Update from Cursors" {
        n498 = Unbundle By Name(w1174) -> ("Sweep Limit [Gauss]"=w1168:dbl, "Modulation Limit [Gauss]"=w1171:dbl)
        n499 = property on="Update Scan/Mod from Cursors" class="Bool (strict)"("Value"=FALSE ("Update Scan/Mod from Cursors")) -> ()  [unwired: 2 in, 2 out]
        n500 = property on="LW,\nAmp" class="Arr (strict)"() -> ("Value"=w1178:dbl[])  [unwired: 2 in, 2 out]
        n501 = Index Array(array=w1178, index=0) -> (element=w1176:dbl)
        n502 = Multiply(x=10.0, y=w1176) -> (x*y=w1167:dbl)
        n503 = Divide(x=w1176, y=3.0) -> (x/y=w1170:dbl)
        n504 = Greater?(x=w1167, y=w1168) -> (0:w1173:bool)
        n505 = Greater?(x=w1170, y=w1171) -> (0:w1172:bool)
        n506 = Select(t=w1168, s=w1173, f=w1167) -> (s? t:f=w1166:dbl)
        n507 = Select(t=w1171, s=w1172, f=w1170) -> (s? t:f=w1169:dbl)
        n508 = property on="Scan range (Gauss)" class="DigNum (strict)"("Value"=w1166) -> ()  [unwired: 2 in, 2 out]
        n509 = Bundle By Name(cluster=w1182, "Scan Width [G]"=w1166, "Mod. Amp. [G]"=w1169) -> (w1181:T7)
        n510 = property on="Mod. Amp. (Gauss)" class="DigNum (strict)"("Value"=w1169) -> ()  [unwired: 2 in, 2 out]
      }
      frame "Flag Bad Set" {
        n511 = property on="Flag Bad Set" class="Bool (strict)"("Value"=FALSE ("Flag Bad Set")) -> ()  [unwired: 2 in, 2 out]
        n512 = Unbundle By Name(w1189) -> ("Set #"=w1188:u32)
        n513 = Greater?(x=w1188, y=u32 1) -> (0:w1186:bool)
        n514 = case shown="True" w1186 {
          tunnel: w1189 -> [w1196 w1198]
          tunnel: [w1196 w1197] -> w1190
          frame False {
            n515 = One Button Dialog(message="No sets collected") -> ()  [unwired: 1 in, 1 out]
          }
          frame True {
            n516 = Two Button Dialog(message="Please confirm that the last set should be flagged as 'bad'\n            Note that 'bad fit' does not mean 'bad set'\n     (closing this window is equivalent to clicking 'No)", 1:"No" ("F button name (\"Cancel\")"), 2:" Yes - last set was bad     " ("T button name (\"OK\")")) -> (T button?=w1199:bool)
            n517 = case shown="False" w1199 {
              tunnel: w1198 -> [w1203 w1210]
              tunnel: [w1203 w1207] -> w1197
              frame False {
              }
              frame True {
                n518 = Unbundle By Name(w1210) -> ("Flagged Bad Sets"=w1206:u32[], "Set #"=w1208:u32)
                n519 = Array Size(array=w1206) -> (size(s)=w1205:i32)
                n520 = Decrement(x=w1208) -> (x-1=w1204:u32)
                n521 = Insert Into Array(array=w1206, index=w1205, new element=w1204) -> (w1209:u32[])
                n522 = Bundle By Name(cluster=w1210, "Flagged Bad Sets"=w1209) -> (w1207:T3)
              }
            }
          }
        }
      }
      frame "Mark transition time" {
        n523 = flat-sequence {
          tunnel: w1214 -> [w1222]
          tunnel: [w1219] -> w1211
          frame #0 {
            n524 = call "Get and Format Time (String).vi"() -> ("Formatted Time"=w1221:string)
            n525 = Bundle By Name(cluster=w1222, "Time of Transition"=w1221) -> (w1220:T3)
            n526 = property on="Applied State" class="Ring (strict)"() -> ("RingText.Text"=w1218:string)  [unwired: 2 in, 2 out]
            n527 = call "Append to Transition State History.vi"("Applied State"=w1218, "Measurement Information In"=w1220) -> ("Measurement Information Out"=w1219:T3)  [unwired: 9 in]
          }
          frame #1 {
            n528 = Two Button Dialog(message="Do you want to start the timer?", 1:"No" ("F button name (\"Cancel\")"), 2:"Yes" ("T button name (\"OK\")")) -> (T button?=w1226:bool)
            n529 = local write "Timer on/off"(w1226) -> ()
          }
        }
        n530 = property on="Mark Time of Transition" class="Bool (strict)"("Value"=FALSE ("Mark Time of Transition")) -> ()  [unwired: 2 in, 2 out]
      }
      frame "Measure Q" {
        n531 = Unbundle By Name(w1227) -> ("Lock-in OK?"=w1230:bool, "Ignore Lock-in Comm. Failure"=w1229:bool)
        n532 = Or(x=w1230, y=w1229) -> (x .or. y?=w1228:bool)
        n533 = case shown="True" w1228 {
          tunnel: [w1237 w1243] -> w1233
          tunnel: [errorcluster {"status"=FALSE, "code"=0, "source"=""} ("error out") w1241] -> w1232
          tunnel: w1227 -> [w1237 w1240]
          frame False {
            n534 = One Button Dialog(message="Unable to communicate with Lock In.\nCannot perform Q-measurement") -> ()  [unwired: 1 in, 1 out]
          }
          frame True {
            n535 = call "Measure Q.vi"("Hardware Parameters"=w1240) -> ("error out"=w1241:errorcluster, "Q Factor"=w1242:dbl, "Hardware Parameters Out"=w1243:T6)  [unwired: 8 in]
            n536 = property on="Q Start" class="DigNum (strict)"("Value"=w1242) -> ()  [unwired: 2 in, 2 out]
          }
        }
        n537 = property on="Get Q" class="Bool (strict)"("Value"=FALSE ("Get Q")) -> ()  [unwired: 2 in, 2 out]
      }
      frame "Measure Noise" {
        n538 = flat-sequence {
          tunnel: [w1255] -> w1244
          frame #0 {
            n539 = global write "Global Variables.vi" "Pause Parallel DAQ"(TRUE ("Pause Parallel DAQ")) -> ()
            n540 = property on="Measure Noise" class="Bool (strict)"("Value"=FALSE ("Measure Noise")) -> ()  [unwired: 2 in, 2 out]
            n541 = global write "Global Variables.vi" "Finished scanning?"(FALSE ("Finished scanning?")) -> ()
          }
          frame #1 {
            n542 = property on="No. Scans/Set" class="DigNum (strict)" props=["Value"]() -> ()  [unwired: 2 in, 3 out]
            n543 = property on="Scan time (sec)" class="DigNum (strict)"() -> ("Value"=w1256:dbl)  [unwired: 2 in, 2 out]
            n544 = call "Measure Noise-Rev1.vi"("Scan Time [s]"=w1256, "Number of Scans"=u32 1) -> ("error out"=w1255:errorcluster, "Out-Phase Noise"=w1253:dbl, "In-Phase Noise"=w1254:dbl)  [unwired: 7 in]
            n545 = property on="In-Phase Noise" class="DigNum (strict)"("Value"=w1254) -> ()  [unwired: 2 in, 2 out]
            n546 = property on="Out-Phase Noise" class="DigNum (strict)"("Value"=w1253) -> ()  [unwired: 2 in, 2 out]
          }
          frame #2 {
            w1257 = FALSE ("Pause Parallel DAQ")
            n547 = global write "Global Variables.vi" "Pause Parallel DAQ"(w1257) -> ()
            n548 = global write "Global Variables.vi" "Abort Scan"(w1257) -> ()
            n549 = global write "Global Variables.vi" "Finished scanning?"(TRUE ("Finished scanning?")) -> ()
          }
        }
      }
      frame "Rotate Magnet" {
        n550 = Unbundle By Name(w1260) -> ("Magnet Rotation"=w1262:bool)
        n551 = case shown="True" w1262 {
          tunnel: w1261 -> [_ w1271]
          tunnel: w1260 -> [_ w1270]
          tunnel: [errorcluster {"status"=FALSE, "code"=0, "source"=""} ("error out") w1268] -> w1259
          frame False {
            n552 = One Button Dialog(message="Magnet rotation is disabled") -> ()  [unwired: 1 in, 1 out]
          }
          frame True {
            n553 = call "Magnet Rotation.vi"("Timeout (sec)"=8.0, "Hardware Parameters"=w1270, "Acquisition Parameters"=w1271) -> ("error out"=w1268:errorcluster, "Achieved Desired Position"=w1267:bool)  [unwired: 7 in]
            n554 = case shown="False" w1267 {
              frame False {
                n555 = One Button Dialog(message="Rotation platform did not arrive at the requested angle.\nPlease check the hardware.") -> ()  [unwired: 1 in, 1 out]
              }
              frame True {
              }
            }
          }
        }
      }
      frame "Lock Field" {
        n556 = Unbundle By Name(w1273) -> ("Fit Spectra"=w1275:dbl[])
        n557 = Empty Array?(array=w1275) -> (empty?=w1274:bool)
        n558 = case shown="True" w1274 {
          tunnel: w1273 -> [w1289 _]
          tunnel: w1281 -> [w1288 w1318]
          tunnel: w1280 -> [w1287 w1317]
          tunnel: [w1286 w1317] -> w1279
          tunnel: [w1285 w1318] -> w1278
          tunnel: w1277 -> [w1284 w1316]
          tunnel: [w1283 w1316] -> w1276
          frame False {
            n559 = flat-sequence {
              tunnel: w1289 -> [w1298]
              tunnel: w1288 -> [w1297]
              tunnel: [w1296] -> w1292
              tunnel: w1287 -> [w1295]
              tunnel: [w1295] -> w1291
              tunnel: w1284 -> [w1294]
              tunnel: [w1294] -> w1290
              tunnel: [w1311] -> w1285
              tunnel: w1292 -> [w1312]
              tunnel: w1291 -> [w1310]
              tunnel: [w1310] -> w1286
              tunnel: w1290 -> [w1309]
              tunnel: [w1309] -> w1283
              frame #0 {
                n560 = property on="Apply & Lock Center Field" class="Bool (strict)"() -> ("Value"=w1299:bool)  [unwired: 2 in, 2 out]
                n561 = property on="Auto Set-based Field Center" class="Bool (strict)"("DisabledEnum"=T10."Enabled" ("Disabled")) -> ()  [unwired: 2 in, 2 out]
                n562 = case shown="True" w1299 {
                  tunnel: w1298 -> [_ w1307]
                  tunnel: w1297 -> [w1300 w1304]
                  tunnel: [w1300 w1303] -> w1296
                  frame False {
                  }
                  frame True {
                    w1301 = TRUE ("Prompt for acquisition updates")
                    n563 = Unbundle By Name(w1307) -> ("Fit Pars"=w1306:dbl[])
                    n564 = property on="Apply & Lock Center Field" class="Bool (strict)"("Value"=FALSE ("Apply & Lock Center Field")) -> ()  [unwired: 2 in, 2 out]
                    n565 = property on="Prompt for acquisition updates" class="Bool (strict)"("Value"=w1301) -> ()  [unwired: 2 in, 2 out]
                    n566 = property on="Auto Set-based Field Center" class="Bool (strict)"("Value"=w1301) -> ()  [unwired: 2 in, 2 out]
                    n567 = Index Array(array=w1306, index=5) -> (element=w1302:dbl)
                    n568 = Bundle By Name(cluster=w1304, "Central Field [G]"=w1302) -> (w1303:T7)
                    n569 = property on="Central field (Gauss)" class="DigNum (strict)"("Value"=w1302) -> ()  [unwired: 2 in, 2 out]
                  }
                }
              }
              frame #1 {
                n570 = property on="Central field (Gauss)" class="DigNum (strict)"() -> ("Value"=w1315:dbl)  [unwired: 2 in, 2 out]
                n571 = call "MiniCircuits UFC-6000 Read Frequency.vi"() -> ("RF [GHz]"=w1314:dbl)  [unwired: 10 in, 1 out]
                n572 = property on="RF (GHz)" class="DigNum (strict)"("Value"=w1314) -> ()  [unwired: 2 in, 2 out]
                n573 = Bundle By Name(cluster=w1312, "Field Locked Frequency [GHz]"=w1314, "Central Field [G]"=w1315, "Locked Central Field [G]"=w1315) -> (w1311:T7)
                n574 = property on="Lock Field" class="Bool (strict)"("Value"=FALSE ("Lock Field")) -> ()  [unwired: 2 in, 2 out]
              }
            }
          }
          frame True {
            n575 = One Button Dialog(message="Please collect at least one scan with an EPR signal") -> ()  [unwired: 1 in, 1 out]
          }
        }
      }
      frame "Engineering Tuning" {
        n576 = property on="Set Freq" class="Bool (strict)"() -> ("Value"=w1322:bool)  [unwired: 2 in, 2 out]
        n577 = case shown="True" w1322 {
          tunnel: w1325 -> [w1334 w1339]
          tunnel: [w1334 w1338] -> w1328
          frame False {
          }
          frame True {
            n578 = call "Network Analyzer and Frequency Tune.vi"("FTUNE(ON)/NETA(OFF)"=FALSE, "Hardware Parameters In"=w1339) -> ("Voltage Output"=w1337:dbl, "Hardware Parameters Out"=w1338:T6)  [unwired: 5 in]
            n579 = property on="Frequency Voltage" class="DigNum (strict)"("Value"=w1337) -> ()  [unwired: 2 in, 2 out]
            n580 = property on="Set Freq" class="Bool (strict)"("Value"=FALSE ("Set Freq")) -> ()  [unwired: 2 in, 2 out]
          }
        }
        n581 = property on="Set Phase" class="Bool (strict)"() -> ("Value"=w1321:bool)  [unwired: 2 in, 2 out]
        n582 = case shown="True" w1321 {
          tunnel: w1328 -> [w1329 w1333]
          tunnel: [w1329 w1332] -> w1326
          frame False {
          }
          frame True {
            n583 = call "Phase Tune.vi"("Hardware Parameters"=w1333) -> ("Phase Voltage [v]"=w1331:dbl, "Hardware Parameters Out"=w1332:T6)  [unwired: 8 in, 1 out]
            n584 = property on="Phase Voltage" class="DigNum (strict)"("Value"=w1331) -> ()  [unwired: 2 in, 2 out]
            n585 = property on="Set Phase" class="Bool (strict)"("Value"=FALSE ("Set Freq")) -> ()  [unwired: 2 in, 2 out]
          }
        }
      }
      frame "Zero Voltages" {
        w1340 = sgl 0.0 ("Output Voltage")
        n586 = Unbundle By Name(w1343) -> ("Lock-in OK?"=w1344:bool)
        n587 = case shown="True" w1344 {
          tunnel: [errorcluster {"status"=FALSE, "code"=0, "source"=""} ("error out") w1355] -> w1345
          tunnel: w1343 -> [_ w1354]
          frame False {
          }
          frame True {
            w1356 = 0 ("Output Voltage [V]")
            n588 = call "Lock-in Output Voltage.vi"("Output Voltage [V]"=w1356, "Output Channel"=enum16{"Ch1", "Ch2"}."Ch1", "Hardware Parameters"=w1354) -> ("error out"=w1359:errorcluster)  [unwired: 8 in]
            n589 = property on="Phase Voltage" class="DigNum (strict)"("Value"=0.0 ("Phase Voltage")) -> ()  [unwired: 2 in, 2 out]
            n590 = call "Lock-in Output Voltage.vi"("error in (no error)"=w1359, "Output Voltage [V]"=w1356, "Output Channel"=enum16{"Ch1", "Ch2"}."Ch2", "Hardware Parameters"=w1354) -> ("error out"=w1355:errorcluster)  [unwired: 7 in]
          }
        }
        n591 = call "Zero Sweep.vi"() -> ("error out"=w1347:errorcluster)  [unwired: 11 in]
        n592 = property on="Zero All Voltage" class="Bool (strict)"("Value"=FALSE ("Zero All Voltage")) -> ()  [unwired: 2 in, 2 out]
        n593 = property on="Frequency Voltage" class="DigNum (strict)"("Value"=w1340) -> ()  [unwired: 2 in, 2 out]
        n594 = call "Set MC Analog Out.vi"("error in (no error)"=w1347, "Channel"=1, "Output Voltage"=w1340) -> ("error out"=w1346:errorcluster)  [unwired: 8 in]
        n595 = Merge Errors(w1345, w1346) -> (w1342:errorcluster)
      }
      frame "Update Center Field" {
        n596 = call "Software-Based FFL.vi"("Hardware Parameters In"=w1365, "Acquisition Parameters In"=w1366) -> ("Hardware Parameters Out"=w1364:T6, "Acquisition Parameters Out"=w1363:T7)  [unwired: 3 in, 1 out]
        n597 = property on="Update Center Field" class="Bool (strict)"("Value"=FALSE ("Update Center Field")) -> ()  [unwired: 2 in, 2 out]
      }
      frame "Refit Data" {
        n598 = property on="Refit Spectra" class="Bool (strict)"("Value"=FALSE ("Refit Spectra")) -> ()  [unwired: 2 in, 2 out]
        n599 = Unbundle By Name(w1374) -> ("Fit Spectra"=w1375:dbl[])
        n600 = Empty Array?(array=w1375) -> (empty?=w1370:bool)
        n601 = case shown="False" w1370 {
          tunnel: w1379 -> [w1390 w1398]
          tunnel: w1378 -> [w1386 w1397]
          tunnel: [w1384 w1399] -> w1377
          tunnel: w1374 -> [w1387 w1399]
          tunnel: [w1390 w1398] -> w1372
          tunnel: [w1386 w1397] -> w1371
          tunnel: w1368 -> [w1383 w1396]
          tunnel: [w1383 w1396] -> w1373
          tunnel: [w1385 _] -> w1369
          frame False {
            n602 = call "Fit EPR Spectra (QSM)-Rev2.vi"("Spectral Data In"=w1387, "Measurement Information"=w1383, "Hardware Parameters In"=w1390, "Acquisition Parameters In"=w1386) -> ("Fit Pars and Labels"=w1391:cluster{"Pars Labels":string[], "pars":dbl[]}, "Spectral Data Out"=w1384:T1, "Number of Fit Iterations"=w1381:i32, "error out"=w1385:errorcluster, "Global SNR"=w1380:dbl)  [unwired: 3 in]
            n603 = Unbundle By Name(w1384) -> ("PDT Amp [v]"=w1389:dbl, "RIS Amp [v]"=w1388:dbl)
            n604 = Unbundle By Name(w1383) -> ("DAQ Mode"=w1382:enum16{"Engineering", "Dosimetry", "Oximetry"})
            n605 = property on="Number of Fit Iterations" class="DigNum (strict)"("Value"=w1381) -> ()  [unwired: 2 in, 2 out]
            n606 = property on="PDT Amp p-p" class="DigNum (strict)"("Value"=w1389) -> ()  [unwired: 2 in, 2 out]
            n607 = property on="Tooth Amp P-P" class="DigNum (strict)"("Value"=w1388) -> ()  [unwired: 2 in, 2 out]
            n608 = property on="Fit Pars and Labels" class="Clust (strict)"("Value"=w1391) -> ()  [unwired: 2 in, 2 out]
            n609 = property on="In-Phase SNR" class="DigNum (strict)"("Value"=w1380) -> ()  [unwired: 2 in, 2 out]
            n610 = case shown="\"Oximetry\"" w1382 {
              tunnel: w1384 -> [_ w1394]
              tunnel: w1383 -> [_ w1393]
              frame Default {
              }
              frame "Oximetry" {
                n611 = call "Calculate pO2-Rev3.vi"("Spectral Data"=w1394, "Measurement Information"=w1393) -> ("pO2 [mmHg]"=w1392:dbl[])  [unwired: 5 in, 4 out]
                n612 = property on="pO2 [mmHg]" class="Arr (strict)"("Value"=w1392) -> ()  [unwired: 2 in, 2 out]
              }
            }
            n613 = call "Update Plots for Spectra Graph.vi"("Spectral Data"=w1384, "Acquisition Parameters"=w1386) -> ()
          }
          frame True {
            n614 = One Button Dialog(message="Please collect at least one scan with an EPR signal") -> ()  [unwired: 1 in, 1 out]
          }
        }
      }
      frame "Open Session Data Folder" {
        n615 = Unbundle By Name(w1405) -> ("Session Path"=w1404:path)
        n616 = Path To String(path=w1404) -> (string=w1402:string)
        n617 = Concatenate Strings("explorer " ("string"), w1402) -> (w1400:string)
        n618 = call <vilib>:"System Exec.vi"("command line"=w1400) -> ("error out"=w1403:errorcluster)  [unwired: 7 in, 3 out]
        n619 = property on="Open Session Data Folder" class="Bool (strict)"("Value"=FALSE ("Open Session Data Folder")) -> ()  [unwired: 2 in, 2 out]
      }
      frame "AfterSave" {
        n620 = Unbundle By Name(w1412) -> ("In-Phase Median Spectra"=w1411:dbl[])
        n621 = Empty Array?(array=w1411) -> (empty?=w1410:bool)
        n622 = case shown="False" w1410 {
          tunnel: w1416 -> [w1421 _]
          tunnel: w1415 -> [w1420 _]
          tunnel: w1414 -> [w1419 _]
          tunnel: w1412 -> [w1418 _]
          tunnel: [w1417 _] -> w1413
          frame False {
            n623 = call "AfterSave-Rev2.vi"("Spectral Data"=w1418, "Measurement Information"=w1419, "Hardware Parameters"=w1420, "Acquisition Parameters"=w1421) -> ("error out"=w1417:errorcluster)  [unwired: 7 in]
          }
          frame True {
            n624 = One Button Dialog(message="Please collect EPR data before using AfterSave") -> ()  [unwired: 1 in, 1 out]
          }
        }
      }
      frame "Undo Auto Update Pars" {
        n625 = property on="Previous Scan range (Gauss)" class="DigNum (strict)"() -> ("Value"=w1424:dbl)  [unwired: 2 in, 2 out]
        n626 = property on="Previous Mod. Amp. (Gauss)" class="DigNum (strict)"() -> ("Value"=w1423:dbl)  [unwired: 2 in, 2 out]
        n627 = property on="Scan range (Gauss)" class="DigNum (strict)"("Value"=w1424) -> ()  [unwired: 2 in, 2 out]
        n628 = property on="Mod. Amp. (Gauss)" class="DigNum (strict)"("Value"=w1423) -> ()  [unwired: 2 in, 2 out]
      }
      frame "Read from Script" {
        w1442 = TRUE ("Save data")
        n629 = call "Load Scripting File-Rev1.vi"("Measurement Information In"=w1438, "Hardware Parameters In"=w1461, "Acquisition Parameters In"=w1462) -> ("error out"=w1429:errorcluster, "Measurement Information Out"=w1432:T3, "Hardware Parameters Out"=w1460:T6, "Acquisition Parameters Out"=w1440:T7, "Finished Script"=w1433:bool, "Sets within script"=w1434:i32)  [unwired: 3 in]
        n630 = Unbundle By Name(w1438) -> ("Set #"=w1437:u32)
        n631 = property on="Scripting Sets" class="DigNum (strict)"("Value"=w1434) -> ()  [unwired: 2 in, 2 out]
        n632 = Unbundle By Name(w1440) -> ("No. Scans/Set"=w1458:u32, "Scan Time [s]"=w1456:dbl, "Pre-Scan Delay [ms]"=w1457:u32, "Central Field [G]"=w1455:dbl, "Scan Width [G]"=w1454:dbl, "Electromagnet Main Field [G]"=w1453:dbl, "Mod. Amp. [G]"=w1452:dbl, "X-Gradient [G/mm]"=w1451:dbl, "Y-Gradient [G/mm]"=w1450:dbl, "Z-Gradient [G/mm]"=w1449:dbl, "Magnet Angle [deg]"=w1448:dbl, "Gradients on/off"=w1447:bool, "Adaptive Tuning"=w1446:bool, "Prompt for oxy acquisition updates"=w1445:bool)
        n633 = Divide(x=w1437, y=w1434) -> (x/y=w1436:dbl)
        n634 = property on="Script Progress" class="Slide (strict)"("Value"=w1436, "Fill Color"=u32 16711680) -> ()  [unwired: 2 in, 2 out]
        n635 = Unbundle By Name(w1460) -> ("Attenuation [dB]"=w1459:u16)
        n636 = property on="Attenuation/dB" class="DigNum (strict)"("Value"=w1459) -> ()  [unwired: 2 in, 2 out]
        n637 = property on="No. Scans/Set" class="DigNum (strict)"("Value"=w1458) -> ()  [unwired: 2 in, 2 out]
        n638 = property on="Scan time (sec)" class="DigNum (strict)"("Value"=w1456) -> ()  [unwired: 2 in, 2 out]
        n639 = property on="Prescan delay (ms)" class="DigNum (strict)"("Value"=w1457) -> ()  [unwired: 2 in, 2 out]
        n640 = property on="Central field (Gauss)" class="DigNum (strict)"("Value"=w1455) -> ()  [unwired: 2 in, 2 out]
        n641 = property on="Scan range (Gauss)" class="DigNum (strict)"("Value"=w1454) -> ()  [unwired: 2 in, 2 out]
        n642 = property on="Electromagnet Main Field (Gauss)" class="DigNum (strict)"("Value"=w1453) -> ()  [unwired: 2 in, 2 out]
        n643 = property on="Mod. Amp. (Gauss)" class="DigNum (strict)"("Value"=w1452) -> ()  [unwired: 2 in, 2 out]
        n644 = property on="X-Gradient [G/mm]" class="DigNum (strict)"("Value"=w1451) -> ()  [unwired: 2 in, 2 out]
        n645 = property on="Y-Gradient [G/mm]" class="DigNum (strict)"("Value"=w1450) -> ()  [unwired: 2 in, 2 out]
        n646 = property on="Z-Gradient [G/mm]" class="DigNum (strict)"("Value"=w1449) -> ()  [unwired: 2 in, 2 out]
        n647 = property on="Magnet Angle (deg)" class="DigNum (strict)"("Value"=w1448) -> ()  [unwired: 2 in, 2 out]
        n648 = property on="Gradients on/off" class="Bool (strict)"("Value"=w1447) -> ()  [unwired: 2 in, 2 out]
        n649 = property on="AdaptiveTune_Enable" class="Bool (strict)"("Value"=w1446) -> ()  [unwired: 2 in, 2 out]
        n650 = property on="Prompt for acquisition updates" class="Bool (strict)"("Value"=w1445) -> ()  [unwired: 2 in, 2 out]
        n651 = Bundle By Name(cluster=w1432, "Save Data"=w1442) -> (w1431:T3)
        n652 = property on="Save data" class="Bool (strict)"("Value"=w1442) -> ()  [unwired: 2 in, 2 out]
        n653 = property on="Start Script" class="Bool (strict)"() -> ("Value"=w1443:bool)  [unwired: 2 in, 2 out]
        n654 = case shown="True" w1443 {
          selector: w1443 -> [w1465 _]
          tunnel: w1433 -> [_ w1472]
          tunnel: [cluster{"Enum":T8, "Data":variant}[] [{"Enum"=enum."Idle", "Data"=variant}] w1471] -> w1444
          tunnel: [w1465 w1470] -> w1441
          tunnel: w1431 -> [w1464 w1469]
          tunnel: [w1464 w1468] -> w1430
          frame False {
            n655 = One Button Dialog(message="Script was aborted") -> ()  [unwired: 1 in, 1 out]
          }
          frame True {
            n656 = case shown="True" w1472 {
              tunnel: [cluster{"Enum":T8, "Data":variant}[] [{"Enum"=enum."Configure Hardware", "Data"=variant}, {"Enum"=enum."Initialize Set", "Data"=variant}, {"Enum"=enum."Pre-Scan", "Data"=variant}] cluster{"Enum":T8, "Data":variant}[] [{"Enum"=enum."Read Config File", "Data"=variant}, {"Enum"=enum."Idle", "Data"=variant}]] -> w1471
              tunnel: [TRUE w1481] -> w1470
              tunnel: w1469 -> [w1473 w1477]
              tunnel: [w1473 w1476] -> w1468
              frame False {
              }
              frame True {
                w1481 = FALSE ("Start Script")
                n657 = property on="Script Progress" class="Slide (strict)"("Fill Color"=u32 6618880) -> ()  [unwired: 2 in, 2 out]
                n658 = property on="Start Script" class="Bool (strict)"("Value"=w1481) -> ()  [unwired: 2 in, 2 out]
                n659 = One Button Dialog(message="Script Completed Successfully") -> ()  [unwired: 1 in, 1 out]
                n660 = call "Format Script Email.vi"("Script Start/End"=enum16{"Start Script", "End Script"}."End Script", "Measurement Information"=w1477) -> ("Measurement Information Out"=w1476:T3)  [unwired: 9 in]
                n661 = call <vilib>:"Beep.vi"("frequency (Hz)"=u32 1000) -> ()  [unwired: 11 in]
              }
            }
          }
        }
        n662 = Bundle By Name(cluster=w1440, "Running Script"=w1441) -> (w1439:T7)
      }
      frame "End Session" {
        w1492 = dbl[] [] ("PDT Amp. History/Set [v]")
        w1493 = dbl[][] [] ("Fit History")
        w1494 = FALSE ("End Session?")
        n663 = property on="End Session?" class="Bool (strict)"("Value"=w1494) -> ()  [unwired: 2 in, 2 out]
        n664 = property on="Auto Set-based Field Center" class="Bool (strict)"("Value"=w1494) -> ()  [unwired: 2 in, 2 out]
        n665 = property on="Prompt for acquisition updates" class="Bool (strict)"("Value"=w1494) -> ()  [unwired: 2 in, 2 out]
        n666 = local write "Timer on/off"(w1494) -> ()
        n667 = property on="Status of EPR DAQ" class="Enum (strict)"() -> ("Strings []"=w1498:string[])  [unwired: 2 in, 2 out]
        n668 = Unbundle By Name(w1484) -> ("DAQ Mode"=w1502:enum16{"Engineering", "Dosimetry", "Oximetry"})
        n669 = call "Save Set Lot.vi"("Measurement Information"=w1484) -> ()  [unwired: 4 in]
        n670 = call "Save DAQ Log.vi"("State Control History"=w1499, "State Control Strings"=w1498, "State Control History Times"=w1500, "Measurement Information"=w1484) -> ("error out"=w1487:errorcluster)  [unwired: 7 in]
        n671 = case shown="\"Oximetry\"" w1502 {
          tunnel: w1484 -> [_ w1510 w1519]
          tunnel: w1496 -> [_ w1513 w1520]
          tunnel: [_ w1512 w1522] -> w1486
          tunnel: w1491 -> [_ _ _]
          frame "Engineering", Default {
          }
          frame "Dosimetry" {
            n672 = Unbundle By Name(w1510) -> ("Skip End Session Save"=w1511:bool)
            n673 = case shown="False" w1511 {
              selector: w1511 -> [_ w1518]
              tunnel: w1510 -> [w1516 _]
              tunnel: w1513 -> [w1515 _]
              tunnel: [w1514 _] -> w1512
              frame False {
                n674 = call "Save PDT and Tooth Amps.vi"("Spectral Data In"=w1515, "Measurement Information In"=w1516) -> ("error out"=w1514:errorcluster)  [unwired: 9 in]
              }
              frame True {
                n675 = Not(x=w1518) -> (.not. x?=w1517:bool)
                n676 = global write "Global Variables.vi" "Abort QA"(w1517) -> ()
              }
            }
          }
          frame "Oximetry" {
            # "Read keys to return\nto default values"
            n677 = Unbundle By Name(w1519) -> ("Session Type"=w1525:string)
            n678 = call "Save Fit Pars-Rev1.vi"("Spectral Data In"=w1520, "Measurement Information In"=w1519) -> ()  [unwired: 9 in, 1 out]
            n679 = call "Save Transition State History Log.vi"("Measurement Information"=w1519) -> ()  [unwired: 11 in]
            n680 = call "Report pO2.vi"("Measurement Information"=w1519) -> ("Report pO2"=w1528:bool)
            n681 = To Lower Case(string=w1525) -> (all lower case string=w1526:string)
            n682 = case shown="True" w1528 {
              tunnel: w1519 -> [_ w1535]
              tunnel: [_ w1533] -> w1521
              tunnel: w1520 -> [_ w1534]
              frame False {
              }
              frame True {
                n683 = call "Generate Oximetry Plots-Rev1.vi"("Spectral Data"=w1534, "Measurement Information"=w1535) -> ("error out"=w1531:errorcluster)  [unwired: 9 in]
                n684 = call "Save pO2 Array-Rev3.vi"("Measurement Information In"=w1535, "Spectral Data"=w1534) -> ("error out"=w1532:errorcluster)  [unwired: 8 in]
                n685 = Merge Errors(w1531, w1532) -> (w1533:errorcluster)
              }
            }
            n686 = Equal?(x=w1526, y="vivo") -> (x = y?=w1524:bool)
            n687 = case shown="True" w1524 {
              tunnel: [_ w1530] -> w1523
              tunnel: w1519 -> [_ w1529]
              frame False {
              }
              frame True {
                n688 = call "Save Session Notes.vi"("Measurement Information"=w1529) -> ("error out"=w1530:errorcluster)  [unwired: 10 in]
              }
            }
            n689 = Merge Errors(w1521, w1523) -> (w1522:errorcluster)
          }
        }
        n690 = Unbundle By Name(w1484) -> ("Set #"=w1490:u32)
        n691 = Greater?(x=w1490, y=u32 1) -> (0:w1488:bool)
        n692 = case shown="True" w1488 {
          tunnel: w1484 -> [_ w1509]
          tunnel: [_ w1508] -> w1485
          frame False {
          }
          frame True {
            n693 = call "Generate Spectra Report.vi"("Measurement Information"=w1509) -> ("error out"=w1508:errorcluster)  [unwired: 10 in]
          }
        }
        n694 = call "Enable and Disable Panel Controls.vi"("VI Reference In"=w1506, "Disabled"=T10."Disabled and Grayed Out", "Items to Hide"=string[] ["Scan?", "End Session?", "Manual Tuning", "Auto-Tune", "Calibrate", "Flag Bad Set", "Apply & Lock Center Field"]) -> ()  [unwired: 2 in, 1 out]
        n695 = Merge Errors(w1485, w1486, w1487) -> (w1497:errorcluster)
        n696 = Bundle By Name(cluster=w1496, "Fit Error History"=w1493, "Fit History"=w1493, "PDT Amp. History/Set [v]"=w1492, "RIS Amp. History/Set [v]"=w1492, "SNR History"=w1492, "Fit Pars"=w1492) -> (w1495:T1)
      }
      frame "Quit Software" {
        n697 = flat-sequence {
          tunnel: w1549 -> [w1560]
          tunnel: [w1553] -> w1548
          tunnel: w1547 -> [w1571]
          tunnel: [w1555] -> w1546
          tunnel: w1544 -> [w1554]
          tunnel: w1543 -> [w1573]
          tunnel: [w1554] -> w1542
          tunnel: [w1573] -> w1540
          tunnel: [w1567] -> w1538
          tunnel: w1548 -> [w1599]
          tunnel: [w1599] -> w1536
          tunnel: w1546 -> [w1598]
          tunnel: [w1598] -> w1545
          tunnel: w1542 -> [w1597]
          tunnel: [w1597] -> w1541
          tunnel: w1540 -> [w1596]
          tunnel: [w1596] -> w1539
          tunnel: [w1595] -> w1537
          tunnel: w1538 -> [w1595]
          frame #0 {
            n698 = Unbundle By Name(w1560) -> ("Lock-in OK?"=w1572:bool)
            n699 = case shown="True" w1572 {
              tunnel: w1571 -> [w1584 w1593]
              tunnel: w1560 -> [w1582 w1590]
              tunnel: [errorcluster {"status"=FALSE, "code"=0, "source"=""} ("error out") w1592] -> w1566
              tunnel: [w1584 w1591] -> w1551
              tunnel: [w1582 w1589] -> w1555
              frame False {
              }
              frame True {
                w1587 = 0.0 ("Mod. Amp. [G]")
                n700 = Bundle By Name(cluster=w1593, "Mod. Amp. [G]"=w1587) -> (w1591:T7)
                n701 = Bundle By Name(cluster=w1590, "Phase Output Voltage [V]"=w1587) -> (w1589:T6)
                n702 = To Long Integer(number=w1587) -> (32bit integer=w1586:i32)
                n703 = call "Lock-in Output Voltage.vi"("Output Voltage [V]"=w1586, "Output Channel"=enum16{"Ch1", "Ch2"}."Ch2", "Hardware Parameters"=w1589) -> ("error out"=w1588:errorcluster)  [unwired: 8 in]
                n704 = call "Configure Lock-in.vi"("error in (no error)"=w1588, "Hardware Parameters"=w1589, "Acquisition Parameters"=w1591) -> ("error out"=w1592:errorcluster)  [unwired: 8 in]
              }
            }
            n705 = call-poly "Write Config Key.vi"("value"=TRUE ("Safe Shutdown?"), "key"="safe_shutdown", "section"="logging") -> ("error out"=w1565:errorcluster)  [unwired: 8 in]
            n706 = call "Zero Sweep.vi"() -> ("error out"=w1557:errorcluster)  [unwired: 11 in]
            n707 = call "Set MC Analog Out.vi"("error in (no error)"=w1557, "Channel"=1, "Output Voltage"=sgl 0.0) -> ("error out"=w1556:errorcluster)  [unwired: 8 in]
            n708 = Unbundle By Name(w1555) -> ("Magnet Type"=w1562:T11)
            n709 = Equal?(x=w1562, y=T11."RRI Electromagnet" ("Magnet Type")) -> (x = y?=w1564:bool)
            n710 = case shown="True" w1564 {
              tunnel: w1555 -> [_ w1580]
              tunnel: [errorcluster {"status"=FALSE, "code"=0, "source"=""} ("error out") w1579] -> w1561
              tunnel: w1551 -> [w1574 w1577]
              tunnel: [w1574 w1576] -> w1550
              frame False {
              }
              frame True {
                w1578 = 0.0 ("Y-Gradient [G/mm]")
                n711 = Bundle By Name(cluster=w1577, "Electromagnet Main Field [G]"=w1578, "X-Gradient [G/mm]"=w1578, "Y-Gradient [G/mm]"=w1578, "Z-Gradient [G/mm]"=w1578) -> (w1576:T7)
                n712 = call "RRI LoadGo - Electromagnet.vi"("Control Coils"=T12."Main and Gradients", "Hardware Parameters"=w1580, "Acquisition Parameters"=w1576) -> ("error out"=w1579:errorcluster)  [unwired: 4 in]
              }
            }
            n713 = call "In-Context Optional Hardware Quit Software.vi"("Measurement Information In"=w1554, "Hardware Parameters In"=w1555, "Acquisition Parameters In"=w1550) -> ("error out"=w1552:errorcluster, "Acquisition Parameters Out"=w1553:T7)  [unwired: 7 in]
            n714 = Merge Errors(w1552, w1561, w1566, w1565, w1556) -> (w1567:errorcluster)
          }
          frame #1 {
            n715 = global write "Global Variables.vi" "Stop(QSM)"(TRUE ("Stop(QSM)")) -> ()
            n716 = property on="Quit" class="Bool (strict)"("Value"=FALSE ("Stop(QSM)")) -> ()  [unwired: 2 in, 2 out]
            n717 = property on="Show Variable Window?" class="Bool (strict)"("Value"=FALSE ("Show Variable Window?")) -> ()  [unwired: 2 in, 2 out]
          }
        }
      }
      frame "Error" {
        n718 = Increment(x="Error Counter") -> (x+1=w1605:i32)
        n719 = property on="Error Counter" class="DigNum (strict)"("Value"=w1605) -> ()  [unwired: 2 in, 2 out]
        "Last Error" <- w1603
      }
    }
    n720 = Equal?(x=w27, y=State_Control."Quit Software" ("State Control")) -> (x = y?=w33:bool)
    n721 = property on="Show Variable Window?" class="Bool (strict)"() -> ("Value"=w32:bool)  [unwired: 2 in, 2 out]
    n722 = call "Erase State History.vi"("State Control History In"=w36, "Erase History? (f)"=w34, "State Control Times In"=w38) -> ("State Control History Out"=w35:T8[], "State Control Times Out"=w37:string[])  [unwired: 7 in]
    n723 = call "Variable Viewer.vi"("Show Variable Window?"=w32, "Spectral Data In"=w28, "Measurement Information In"=w29, "Hardware Parameters In"=w30, "Acquisition Parameters In"=w31) -> ("Spectral Data"=w18:T1, "Measurement Information"=w19:T3, "Hardware Parameters"=w20:T6, "Acquisition Parameters"=w21:T7)  [unwired: 3 in]
    n724 = call "Queue Manager.vi"("queue in"=w60, "Queue States In"=w46, "Error IN"=w39, "Ignore Errors"="Ignore Errors") -> ("queue out"=w56:refnum<queue>, "Last Error"=w44:errorcluster, "Error OUT"=w58:errorcluster)  [unwired: 9 in]
    "Consumer Loop" <- w54
  }
  n725 = stacked-sequence {
    frame #0 {
      # "Some rare development runtime crashes can cause the MC background service not to finish, in which case the background service needs to be force stopped. \nTo prevent this from happening in either development or deployment, these functions are called at the start of the DAQ to ensure that unforseen crashes to not warrant a computer restart."
      n726 = flat-sequence {
        frame #0 {
          n727 = call "STOPBG.VI"("Function Type"=1) -> ()  [unwired: 1 in, 2 out]
        }
        frame #1 {
          n728 = call "STOPBG.VI"("Function Type"=2) -> ()  [unwired: 1 in, 2 out]
        }
      }
    }
    frame #1 {
      w1614 = u32 10 ("millisecond multiple")
      # "Parallel Threads"
      n729 = while {
        shift-right: [w1675] -> _
        shift-left: _ -> [w1666]
        tunnel: w1614 -> [w1673]
        shift-right: [w1661] -> _
        shift-left: 0.0 ("SpO2 [%]") -> [w1660]
        stop <- w1674 stop-if-true
        # "Parallel DAQ to Update Meters"
        n730 = global read "Global Variables.vi" "Pause Parallel DAQ"() -> (w1664:bool)
        n731 = Wait (ms)(milliseconds to wait=w1673) -> ()  [unwired: 1 out]
        n732 = Not(x=w1664) -> (.not. x?=w1663:bool)
        n733 = And(x=w1663, y="Acquire SpO2") -> (x .and. y?=w1662:bool)
        n734 = property on="Balance/Phase/AFC Meter" class="Knob (strict)"("Value"=w1666) -> ()  [unwired: 2 in, 2 out]
        n735 = case shown="False" w1664 {
          tunnel: w1666 -> [_ w1703]
          tunnel: [w1686 w1702] -> w1672
          tunnel: [w1685 w1701] -> w1671
          tunnel: [w1684 w1700] -> w1670
          tunnel: "Balance Scale Factor" -> [w1683 _]
          tunnel: "Phase Scale Factor" -> [w1682 _]
          tunnel: "AFC Scale Factor" -> [w1681 _]
          frame False {
            n736 = for {
              N: 4 -> [_]
              tunnel: [w1699] -> w1687 mode=indexing
              tunnel: [w1695] -> _ mode=indexing
              i -> [w1698]
              n737 = Add(x=w1698, y=2) -> (x+y=w1696:i32)
              n738 = call "Read MC Analog In.vi"("channel"=w1696) -> ("error out"=w1695:errorcluster, "Voltage Input"=w1699:dbl)  [unwired: 9 in]
            }
            n739 = Index Array(array=w1687, index #1=0 ("index"), index #2=1 ("index"), index #3=2 ("index")) -> (element #1=w1690:dbl, element #2=w1689:dbl, element #3=w1688:dbl)
            n740 = Multiply(x=w1690, y=w1683) -> (x*y=w1686:dbl)
            n741 = Multiply(x=w1689, y=w1682) -> (x*y=w1685:dbl)
            n742 = Multiply(x=w1688, y=w1681) -> (x*y=w1684:dbl)
          }
          frame True {
            n743 = Unbundle(w1703) -> (w1702:dbl, w1701:dbl, w1700:dbl)
          }
        }
        n744 = case shown="True" w1662 {
          tunnel: [w1676 w1679] -> w1661
          tunnel: w1660 -> [w1676 _]
          frame False {
          }
          frame True {
            n745 = call "Read SpO2.vi"("SpO2 Calibration [SpO2/V]"="SpO2 Calibration [SpO2/V]") -> ("Color Out"=w1677:u32, "SpO2 [%]"=w1679:dbl)  [unwired: 8 in, 1 out]
            n746 = property on="SpO2 [%]" class="DigNum (strict)"("NumText.BGColor"=w1677, "NumText.TextColor"=w1677, "NumText.FontColor"=u32 0) -> ()  [unwired: 2 in, 2 out]
          }
        }
        "SpO2 [%]" <- w1661
        n747 = global read "Global Variables.vi" "Stop(QSM)"() -> (w1674:bool)
        n748 = Bundle(cluster=w1666, w1672, w1671, w1670) -> (w1675:cluster{dbl, dbl, dbl})
      }
      n749 = while {
        stop <- w1657 stop-if-true
        # "Development"
        n750 = property on="State Control History" class="Arr (strict)"() -> ("Value"=w1653:T8[])  [unwired: 2 in, 2 out]
        n751 = Array Size(array=w1653) -> (size(s)=w1651:i32)
        n752 = To Unsigned Long Integer(number=w1651) -> (unsigned 32bit integer=w1650:u32)
        n753 = Subtract(x=w1650, y=u32 20) -> (x-y=w1654:u32)
        n754 = Build Array(w1654) -> (w1652:u32[])
        n755 = property on="State Control History" class="Arr (strict)"("Index Values"=w1652) -> ()  [unwired: 2 in, 2 out]
        n756 = Wait (ms)(milliseconds to wait=u32 250 ("millisecond multiple")) -> ()  [unwired: 1 out]
        n757 = global read "Global Variables.vi" "Stop(QSM)"() -> (w1657:bool)
        n758 = case shown="True" "Show All" {
          frame False {
          }
          frame True {
            n759 = control-ref of="This VI"() -> (w1659:refnum<vi>)
            n760 = call "Show and Hide Panel Controls.vi"("VI Reference In"=w1659) -> ()  [unwired: 4 in, 1 out]
          }
        }
      }
      n761 = while {
        tunnel: w1614 -> [w1626]
        stop <- w1625 stop-if-true
        w1623 = u32 3  # Seconds to display
        # "Display Popups"
        n762 = global read "Global Variables.vi" "Display Popup"() -> (w1624:bool)
        n763 = Wait (ms)(milliseconds to wait=w1626) -> ()  [unwired: 1 out]
        n764 = global read "Global Variables.vi" "Stop(QSM)"() -> (w1625:bool)
        n765 = case shown="False" w1624 {
          tunnel: w1623 -> [_ w1627]
          frame False {
          }
          frame True {
            n766 = call "Popup Message.vi"("Seconds to display"=w1627) -> ()  [unwired: 2 in]
          }
        }
      }
      n767 = while {
        tunnel: w1614 -> [w1641]
        stop <- w1640 stop-if-true
        # "Timer"
        n768 = Wait (ms)(milliseconds to wait=w1641) -> ()  [unwired: 1 out]
        n769 = global read "Global Variables.vi" "Finished scanning?"() -> (w1632:bool)
        n770 = case shown="True" "Timer on/off" {
          tunnel: [T10."Enabled" ("Disabled") T10."Disabled and Grayed Out" ("Disabled")] -> w1629
          frame False {
          }
          frame True {
          }
        }
        n771 = Not(x="Timer on/off") -> (.not. x?=w1636:bool)
        n772 = call "Elapsed Time"("Time Target (s)"="Timer Value", "Reset"=w1636, "Auto Reset"=FALSE) -> ("Elapsed Time (s)"=w1637:dbl, "Time has Elapsed"=w1630:bool)  [unwired: 9 in, 6 out]
        n773 = global write "Global Variables.vi" "Timer Elapsed"(w1630) -> ()
        n774 = And(x=w1632, y=w1630) -> (x .and. y?=w1639:bool)
        n775 = Less?(x="Timer Value", y=1.0) -> (x < y?=w1633:bool)
        n776 = case shown="True" w1639 {
          tunnel: w1633 -> [_ w1644]
          frame False {
          }
          frame True {
            n777 = One Button Dialog(message="Timer Elapsed") -> (true=w1645:bool)  [unwired: 1 in]
            n778 = And(x=w1645, y=w1644) -> (x .and. y?=w1646:bool)
            n779 = Not(x=w1645) -> (.not. x?=w1647:bool)
            n780 = case shown="True" w1646 {
              frame False {
              }
              frame True {
                n781 = property on="Timer Value" class="DigNum (strict)"("Value"=1.0 ("Timer")) -> ()  [unwired: 2 in, 2 out]
              }
            }
            n782 = property on="Timer on/off" class="Bool (strict)"("Value"=w1647) -> ()  [unwired: 2 in, 2 out]
          }
        }
        n783 = property on="Mark Time of Transition" class="Bool (strict)"("DisabledEnum"=w1629) -> ()  [unwired: 2 in, 2 out]
        n784 = Subtract(x="Timer Value", y=w1637) -> (x-y=→"Time Remaining":dbl)
        n785 = global read "Global Variables.vi" "Stop(QSM)"() -> (w1640:bool)
      }
      n786 = while {
        tunnel: w1614 -> [w1615]
        stop <- w1616 stop-if-true
        w1617 = T10."Enabled" ("Disabled")
        w1619 = T10."Disabled and Grayed Out" ("Disabled")
        # "Temporary Conditional Disables"
        n787 = Wait (ms)(milliseconds to wait=w1615) -> ()  [unwired: 1 out]
        n788 = global read "Global Variables.vi" "Stop(QSM)"() -> (w1616:bool)
        n789 = property on="AFC Field Correction" class="Bool (strict)"() -> ("Value"=w1622:bool)  [unwired: 2 in, 2 out]
        n790 = property on="Continuous Sweeping" class="Bool (strict)"() -> ("Value"=w1620:bool)  [unwired: 2 in, 2 out]
        n791 = Select(t=w1619, s=w1622, f=w1617) -> (s? t:f=w1621:T10)
        n792 = Select(t=w1619, s=w1620, f=w1617) -> (s? t:f=w1618:T10)
        n793 = property on="Continuous Sweeping" class="Bool (strict)"("DisabledEnum"=w1621) -> ()  [unwired: 2 in, 2 out]
        n794 = property on="AFC Field Correction" class="Bool (strict)"("DisabledEnum"=w1618) -> ()  [unwired: 2 in, 2 out]
      }
      n795 = while {
        tunnel: w1614 -> [w1721]
        stop <- w1763 stop-if-true
        # "In Phase Median"
        # "Out of Phase Median"
        # "Out of Phase Scan/Average"
        # "In-Phase Scan/Average"
        # "Update Graph"
        n796 = property on="Spectra Graph" class="XYGraph (strict)"() -> ("CrsrList"=w1764:T15)  [unwired: 2 in, 2 out]
        n797 = property on="Central field (Gauss)" class="DigNum (strict)"() -> ("Value"=w1713:dbl)  [unwired: 2 in, 2 out]
        n798 = property on="Scan range (Gauss)" class="DigNum (strict)"() -> ("Value"=w1704:dbl)  [unwired: 2 in, 2 out]
        n799 = property on="Spectra Graph" class="XYGraph (strict)"() -> ("YScale.Maximum"=w1707:dbl, "YScale.Minimum"=w1706:dbl)  [unwired: 2 in, 2 out]
        n800 = global read "Global Variables.vi" "Graphing Array"() -> (w1729:dbl[][])
        n801 = global read "Global Variables.vi" "B-Field"() -> (w1716:dbl[])
        n802 = Index Array(array=w1764, index #1=0 ("index"), index #2=1 ("index")) -> (element #1=w1762:T16, element #2=w1761:T16)
        n803 = Multiply(x=w1704, y=0.3) -> (x*y=w1709:dbl)
        n804 = Unbundle By Name(w1762) -> ("Position.X"=w1755:dbl)
        n805 = Unbundle By Name(w1762) -> ("Position.Y"=w1759:dbl)
        n806 = Unbundle By Name(w1761) -> ("Position.Y"=w1758:dbl)
        n807 = Unbundle By Name(w1761) -> ("Position.X"=w1756:dbl)
        n808 = property on="Visible-In Phase" class="Bool (strict)"() -> ("Value"=w1750:bool)  [unwired: 2 in, 2 out]
        n809 = property on="Visible-Out Phase" class="Bool (strict)"() -> ("Value"=w1748:bool)  [unwired: 2 in, 2 out]
        n810 = property on="Visible-Median In Phase" class="Bool (strict)"() -> ("Value"=w1746:bool)  [unwired: 2 in, 2 out]
        n811 = property on="Visible-Median Out Phase" class="Bool (strict)"() -> ("Value"=w1738:bool)  [unwired: 2 in, 2 out]
        n812 = property on="Visible-CFit" class="Bool (strict)"() -> ("Value"=w1740:bool)  [unwired: 2 in, 2 out]
        n813 = property on="Visible-CFitNoBaseline" class="Bool (strict)"() -> ("Value"=w1742:bool)  [unwired: 2 in, 2 out]
        n814 = property on="Visible-Center PDT" class="Bool (strict)"() -> ("Value"=w1744:bool)  [unwired: 2 in, 2 out]
        n815 = Add(x=w1713, y=w1709) -> (x+y=w1710:dbl)
        n816 = Transpose Matrix(1:w1729) -> (0:w1728:dbl[][])
        n817 = Not(x=w1750) -> (.not. x?=w1749:bool)
        n818 = Not(x=w1748) -> (.not. x?=w1747:bool)
        n819 = Not(x=w1746) -> (.not. x?=w1745:bool)
        n820 = Not(x=w1738) -> (.not. x?=w1737:bool)
        n821 = Not(x=w1740) -> (.not. x?=w1739:bool)
        n822 = Not(x=w1742) -> (.not. x?=w1741:bool)
        n823 = Not(x=w1744) -> (.not. x?=w1743:bool)
        n824 = Build Array(w1710, w1710) -> (w1711:dbl[])
        n825 = Build Array(w1707, w1706) -> (w1712:dbl[])
        n826 = Index Array(array=w1728, index (row) #1=0 ("index (row)"), index (row) #2=1 ("index (row)"), index (row) #3=2 ("index (row)"), index (row) #4=3 ("index (row)"), index (row) #5=4 ("index (row)"), index (row) #6=5 ("index (row)")) -> (element #1=w1736:dbl[], element #2=w1732:dbl[], element #3=w1726:dbl[], element #4=w1725:dbl[], element #5=w1718:dbl[], element #6=w1717:dbl[])  [unwired: 6 in]
        n827 = Subtract(x=w1755, y=w1756) -> (x-y=w1757:dbl)
        n828 = Subtract(x=w1759, y=w1758) -> (x-y=w1760:dbl)
        n829 = Bundle(w1711, w1712) -> (w1705:cluster{dbl[], dbl[]})  [unwired: 1 out]
        n830 = Build Array(w1749, w1747, w1745, w1737, w1739, w1741, w1743) -> (w1751:bool[])
        n831 = Absolute Value(x=w1757) -> (abs(x)=w1754:dbl)
        n832 = Absolute Value(x=w1760) -> (abs(x)=w1753:dbl)
        n833 = Bundle("B-Field"=w1716, "Graphing Array"=w1736) -> (w1735:cluster{"B-Field":dbl[], "Graphing Array":dbl[]})  [unwired: 1 in]
        n834 = Bundle("B-Field"=w1716, "Graphing Array"=w1732) -> (w1731:cluster{"B-Field":dbl[], "Graphing Array":dbl[]})  [unwired: 1 in]
        n835 = Bundle("B-Field"=w1716, "Graphing Array"=w1726) -> (w1723:cluster{"B-Field":dbl[], "Graphing Array":dbl[]})  [unwired: 1 in]
        n836 = Bundle("B-Field"=w1716, "Graphing Array"=w1725) -> (w1722:cluster{"B-Field":dbl[], "Graphing Array":dbl[]})  [unwired: 1 in]
        n837 = Bundle("B-Field"=w1716, "Graphing Array"=w1718) -> (w1715:cluster{"B-Field":dbl[], "Graphing Array":dbl[]})  [unwired: 1 in]
        n838 = Bundle("B-Field"=w1716, "Graphing Array"=w1717) -> (w1714:cluster{"B-Field":dbl[], "Graphing Array":dbl[]})  [unwired: 1 in]
        n839 = for {
          tunnel: w1751 -> [w1769] mode=indexing
          i -> [w1768]
          n840 = To Unsigned Long Integer(number=w1768) -> (unsigned 32bit integer=w1767:u32)
          n841 = property on="Spectra Graph" class="XYGraph (strict)"("Active Plot"=w1767, "Plot.Visible?"=w1769) -> ()  [unwired: 2 in, 2 out]
        }
        n842 = global read "Global Variables.vi" "Stop(QSM)"() -> (w1763:bool)
        n843 = Build Array(w1754, w1753) -> (w1752:dbl[])
        n844 = Build Array(w1735, w1731, w1723, w1722, w1715, w1714, w1705) -> (w1730:T18)
        n845 = property on="LW,\nAmp" class="Arr (strict)"("Value"=w1752) -> ()  [unwired: 2 in, 2 out]
        n846 = property on="Spectra Graph" class="XYGraph (strict)"("Value"=w1730) -> ()  [unwired: 2 in, 2 out]
        n847 = Wait (ms)(milliseconds to wait=w1721) -> ()  [unwired: 1 out]
      }
    }
  }
  n848 = stacked-sequence {
    frame #0 {
      w1789 = ""
      w1792 = dbl[][] [] ("Calibration dBpp/Set [Gauss]")
      w1790 = 0.0 ("Phase Voltage")
      w1793 = FALSE ("Show Calibration Constants")
      w1805 = u32 16711680
      w1807 = u32 6618880
      # "Initialize GUI variables, colors, and panel size"
      n849 = property on="Fit Pars and Labels" class="Clust (strict)"("Value"=cluster{"Pars Labels":string[], "pars":dbl[]} {"Pars Labels"=[], "pars"=[]} ("Fit Pars and Labels")) -> ()  [unwired: 2 in, 2 out]
      n850 = property on="Show Calibration Constants" class="Bool (strict)"("Value"=w1793) -> ()  [unwired: 2 in, 2 out]
      n851 = property on="Show Variable Window?" class="Bool (strict)"("Value"=w1793) -> ()  [unwired: 2 in, 2 out]
      n852 = property on="Directory Input" class="Str"("Value"=w1789) -> ()  [unwired: 2 in, 2 out]
      n853 = property on="Comments" class="Str"("Value"=w1789) -> ()  [unwired: 2 in, 2 out]
      n854 = property on="Sample ID" class="Str"("Value"=w1789) -> ()  [unwired: 2 in, 2 out]
      n855 = property on="Volunteer ID" class="Str"("Value"=w1789) -> ()  [unwired: 2 in, 2 out]
      n856 = property on="Operators" class="Str"("Value"=w1789) -> ()  [unwired: 2 in, 2 out]
      n857 = property on="Session Type" class="Str"("Value"=w1789) -> ()  [unwired: 2 in, 2 out]
      n858 = property on="Out-Phase Noise" class="DigNum (strict)"("Value"=w1790) -> ()  [unwired: 2 in, 2 out]
      n859 = property on="In-Phase Noise" class="DigNum (strict)"("Value"=w1790) -> ()  [unwired: 2 in, 2 out]
      n860 = property on="Frequency Voltage" class="DigNum (strict)"("Value"=w1790) -> ()  [unwired: 2 in, 2 out]
      n861 = property on="Phase Voltage" class="DigNum (strict)"("Value"=w1790) -> ()  [unwired: 2 in, 2 out]
      n862 = property on="In Phase Offset" class="DigNum (strict)"("Value"=w1790) -> ()  [unwired: 2 in, 2 out]
      n863 = property on="Out Phase Offset" class="DigNum (strict)"("Value"=w1790) -> ()  [unwired: 2 in, 2 out]
      n864 = property on="Q Start" class="DigNum (strict)"("Value"=w1790) -> ()  [unwired: 2 in, 2 out]
      n865 = property on="Script Progress" class="Slide (strict)"("Value"=w1790) -> ()  [unwired: 2 in, 2 out]
      n866 = property on="Set Progress" class="Slide (strict)"("Value"=w1790) -> ()  [unwired: 2 in, 2 out]
      n867 = control-ref of="This VI"() -> (w1778:refnum<vi>)
      n868 = property on="Error Counter" class="DigNum (strict)"("Value"=0 ("Error Counter")) -> ()  [unwired: 2 in, 2 out]
      n869 = property on="pO2/Scan [mmHg]" class="WFGraph (strict)"("Value"=w1792) -> ()  [unwired: 2 in, 2 out]
      n870 = property on="Linewidth (HWHM)/Set [Gauss]" class="WFGraph (strict)"("Value"=w1792) -> ()  [unwired: 2 in, 2 out]
      n871 = property on="Linewidth (HWHM) [Gauss]" class="WFGraph (strict)"("Value"=w1792) -> ()  [unwired: 2 in, 2 out]
      n872 = property on="pO2/Set [mmHg]" class="WFGraph (strict)"("Value"=w1792) -> ()  [unwired: 2 in, 2 out]
      n873 = property class="VI"(reference=w1778) -> (reference out=w1770:refnum<vi>, error out=w1779:errorcluster, "Panel"=w1780:refnum<vi>)  [unwired: 1 in]
      n874 = property class="Pnl"(reference=w1780, error in=w1779) -> (reference out=w1771:refnum<vi>, error out=w1781:errorcluster, "Panes[]"=w1782:refnum<vi>[])
      n875 = Index Array(array=w1782, index=0) -> (element=w1784:refnum<vi>)
      n876 = property class="Pane"(reference=w1784, error in=w1781) -> (reference out=w1773:refnum<vi>, error out=w1772:errorcluster, "Origin"=w1785:T19)
      n877 = Bundle By Name(cluster=w1785, "Horizontal"=i16 -522, "Vertical"=i16 -663) -> (w1786:T19)
      n878 = Bundle("y"=-10.0, w1805) -> (w1802:cluster{"y":dbl, u32})  [unwired: 1 in]
      n879 = Bundle("y"=-2.5, w1807) -> (w1799:cluster{"y":dbl, u32})  [unwired: 1 in]
      n880 = Bundle("y"=0.0, w1807) -> (w1796:cluster{"y":dbl, u32})  [unwired: 1 in]
      n881 = Bundle("y"=2.5, w1805) -> (w1801:cluster{"y":dbl, u32})  [unwired: 1 in]
      n882 = Bundle("y"=10.0, w1805) -> (w1803:cluster{"y":dbl, u32})  [unwired: 1 in]
      n883 = property class="Pane"(reference=w1773, error in=w1772, "Origin"=w1786) -> (reference out=w1774:refnum<vi>, error out=w1775:errorcluster)
      n884 = Build Array(w1802, w1799, w1796, w1801, w1803) -> (w1794:cluster{"y":dbl, u32}[])
      n885 = property on="Balance/Phase/AFC Meter" class="Knob (strict)"("Scale.MarkerVals[]"=w1794) -> ()  [unwired: 2 in, 2 out]
      n886 = Close Reference(reference=w1774, error in (no error)=w1775) -> (error out=w1777:errorcluster)
      n887 = Close Reference(reference=w1771, error in (no error)=w1777) -> (error out=w1776:errorcluster)
      n888 = Close Reference(reference=w1770, error in (no error)=w1776) -> ()  [unwired: 1 out]
    }
    frame #1 {
      # "User Mode"
    }
    frame #2 {
      # "Mode-Specific Options"
    }
  }
  n889 = while {
    tunnel: w11 -> [w1812]
    i -> [w1811]
    stop <- w1810 stop-if-true
    n890 = event shown="[28] \"End Session?\": Value Change" {
      selector: _ -> [_ _ _ _ _ _ _ _ _ _ _ _ _ _ _ _ _ _ _ _ _ _ _ _ _ _ _ _ _]
      dyn-events: _ -> [_ _ _ _ _ _ _ _ _ _ _ _ _ _ _ _ _ _ _ _ _ _ _ _ _ _ _ _ _]
      timeout: _ -> [_ _ _ _ _ _ _ _ _ _ _ _ _ _ _ _ _ _ _ _ _ _ _ _ _ _ _ _ _]
      tunnel: w1812 -> [w1814 _ w1818 w1820 _ w1834 w1878 w1880 w1884 w1886 w1887 w1889 w1891 w1893 w1895 w1897 w1899 w1901 w1903 w1905 w1907 w1909 w1911 w1913 w1915 w1917 w1919 w1921 w1924]
      tunnel: [TRUE ("x") _ _ _ _ _ _ _ _ _ _ _ _ _ _ _ _ _ _ _ _ _ _ _ _ _ _ _ _] -> w1808
      event "Quit": Value Change {
        n891 = event-data() -> ()  [unwired: 1 in, 5 out]
        n892 = call "Queue Manager.vi"("queue in"=w1814, "Queue States In"=cluster{"Enum":T8, "Data":variant}[] [{"Enum"=enum."Quit Software", "Data"=variant}]) -> ()  [unwired: 11 in, 3 out]
      }
      event "Applied State": Value Change {
        n893 = event-data() -> ("OldVal"=w1817:i32, "NewVal"=w1816:i32)  [unwired: 1 in, 3 out]
        n894 = property on="Initial State" class="Ring (strict)"("Value"=w1817) -> ()  [unwired: 2 in, 2 out]
        n895 = property on="Applied State" class="Ring (strict)"("Value"=w1816) -> ()  [unwired: 2 in, 2 out]
      }
      event "Mode": Value Change {
        n896 = event-data() -> ()  [unwired: 1 in, 5 out]
        n897 = call "Queue Manager.vi"("queue in"=w1818, "Queue States In"=cluster{"Enum":T8, "Data":variant}[] [{"Enum"=enum."Read GUI Pars", "Data"=variant}, {"Enum"=enum."Idle", "Data"=variant}]) -> ()  [unwired: 11 in, 3 out]
      }
      event "Update Scan/Mod from Cursors": Value Change {
        n898 = event-data() -> ()  [unwired: 1 in, 5 out]
        n899 = call "Queue Manager.vi"("queue in"=w1820, "Queue States In"=cluster{"Enum":T8, "Data":variant}[] [{"Enum"=enum."Update from Cursors", "Data"=variant}, {"Enum"=enum."Idle", "Data"=variant}]) -> ()  [unwired: 11 in, 3 out]
      }
      event "Stop Scan": Value Change {
        n900 = event-data() -> ()  [unwired: 1 in, 5 out]
        n901 = global read "Global Variables.vi" "Finished scanning?"() -> (w1824:bool)
        n902 = Not(x=w1824) -> (.not. x?=w1823:bool)
        n903 = property on="Stop Scan" class="Bool (strict)"("Value"=FALSE ("Stop Scan")) -> ()  [unwired: 2 in, 2 out]
        n904 = global write "Global Variables.vi" "Abort Scan"(w1823) -> ()
      }
      event Menu Selection (User) {
        w1825 = 1 ("offset (0)")
        w1826 = ":" ("search string/char (-)")
        n905 = event-data() -> ("MenuRef"=w1827:refnum<k9>, "ItemPath"=w1830:string)  [unwired: 1 in, 4 out]
        n906 = Search/Split String(string=w1830, search string/char (-)=w1826) -> (match + rest of string=w1831:string)  [unwired: 1 in, 2 out]
        n907 = String Subset(string=w1831, offset (0)=w1825) -> (substring=w1832:string)  [unwired: 1 in]
        n908 = Search/Split String(string=w1832, search string/char (-)=w1826) -> (substring before match=w1829:string, match + rest of string=w1833:string)  [unwired: 1 in, 1 out]
        n909 = String Subset(string=w1833, offset (0)=w1825) -> (substring=w1828:string)  [unwired: 1 in]
        n910 = case shown="\"Show/Hide Variables\"" w1829 {
          tunnel: w1834 -> [w1835 w1842 w1872 w1874 w1875 _]
          tunnel: w1828 -> [_ w1844 _ _ _ _]
          tunnel: w1827 -> [_ w1846 _ _ _ _]
          frame "Change Calibration Values" {
            n911 = flat-sequence {
              tunnel: w1835 -> [w1840]
              frame #0 {
                n912 = Two Button Dialog(message="Are you sure you wish to change the calibration values?", 1:"Hide values" ("F button name (\"Cancel\")"), 2:"Change values" ("T button name (\"OK\")")) -> (T button?=w1836:bool)
                n913 = property on="Show Calibration Constants" class="Bool (strict)"("Value"=w1836) -> ()  [unwired: 2 in, 2 out]
              }
              frame #1 {
                n914 = call "Queue Manager.vi"("queue in"=w1840, "Queue States In"=cluster{"Enum":T8, "Data":variant}[] [{"Enum"=enum."Read GUI Pars", "Data"=variant}, {"Enum"=enum."Idle", "Data"=variant}]) -> ()  [unwired: 11 in, 3 out]
              }
            }
          }
          frame "DAQ Mode" {
            n915 = Set Menu Item Info(6:TRUE ("checked"), 7:w1844, 11:w1846) -> (3:w1843:refnum<k9>)  [unwired: 4 in, 1 out]
            n916 = flat-sequence {
              tunnel: w1844 -> [w1848]
              tunnel: w1843 -> [w1847]
              tunnel: w1842 -> [w1867]
              frame #0 {
                n917 = case shown="\"Engineering\"" w1848 {
                  tunnel: w1847 -> [w1854 w1860 w1866 _]
                  frame "Dosimetry" {
                    w1850 = FALSE ("checked")
                    n918 = Set Menu Item Info(6:w1850, 7:"Oximetry" ("item tag"), 11:w1854) -> (3:w1853:refnum<k9>)  [unwired: 4 in, 1 out]
                    n919 = Set Menu Item Info(6:w1850, 7:"Engineering" ("item tag"), 11:w1853) -> ()  [unwired: 4 in, 2 out]
                    n920 = property on="DAQ Mode" class="Enum (strict)"("Value"=enum16{"Engineering", "Dosimetry", "Oximetry"}."Dosimetry" ("DAQ Mode")) -> ()  [unwired: 2 in, 2 out]
                  }
                  frame "Oximetry" {
                    w1856 = FALSE ("checked")
                    n921 = Set Menu Item Info(6:w1856, 7:"Dosimetry" ("item tag"), 11:w1860) -> (3:w1859:refnum<k9>)  [unwired: 4 in, 1 out]
                    n922 = Set Menu Item Info(6:w1856, 7:"Engineering" ("item tag"), 11:w1859) -> ()  [unwired: 4 in, 2 out]
                    n923 = property on="DAQ Mode" class="Enum (strict)"("Value"=enum16{"Engineering", "Dosimetry", "Oximetry"}."Oximetry" ("DAQ Mode")) -> ()  [unwired: 2 in, 2 out]
                  }
                  frame "Engineering" {
                    w1862 = FALSE ("checked")
                    n924 = Set Menu Item Info(6:w1862, 7:"Oximetry" ("item tag"), 11:w1866) -> (3:w1865:refnum<k9>)  [unwired: 4 in, 1 out]
                    n925 = Set Menu Item Info(6:w1862, 7:"Dosimetry" ("item tag"), 11:w1865) -> ()  [unwired: 4 in, 2 out]
                    n926 = property on="DAQ Mode" class="Enum (strict)"("Value"=enum16{"Engineering", "Dosimetry", "Oximetry"}."Engineering" ("DAQ Mode")) -> ()  [unwired: 2 in, 2 out]
                  }
                  frame Default {
                  }
                }
              }
              frame #1 {
                n927 = call "Queue Manager.vi"("queue in"=w1867, "Queue States In"=cluster{"Enum":T8, "Data":variant}[] [{"Enum"=enum."Read GUI Pars", "Data"=variant}, {"Enum"=enum."Idle", "Data"=variant}]) -> ()  [unwired: 11 in, 3 out]
              }
            }
          }
          frame "Show/Hide Variables" {
            n928 = property on="Show Variable Window?" class="Bool (strict)"() -> ("Value"=w1871:bool)  [unwired: 2 in, 2 out]
            n929 = Not(x=w1871) -> (.not. x?=w1870:bool)
            n930 = property on="Show Variable Window?" class="Bool (strict)"("Value"=w1870) -> ()  [unwired: 2 in, 2 out]
            n931 = call "Queue Manager.vi"("queue in"=w1872, "Queue States In"=cluster{"Enum":T8, "Data":variant}[] [{"Enum"=enum."Read GUI Pars", "Data"=variant}, {"Enum"=enum."Idle", "Data"=variant}]) -> ()  [unwired: 11 in, 3 out]
          }
          frame "AfterSave" {
            n932 = call "Queue Manager.vi"("queue in"=w1874, "Queue States In"=cluster{"Enum":T8, "Data":variant}[] [{"Enum"=enum."Read GUI Pars", "Data"=variant}, {"Enum"=enum."AfterSave", "Data"=variant}, {"Enum"=enum."Idle", "Data"=variant}]) -> ()  [unwired: 11 in, 3 out]
          }
          frame "Undo Auto Update Pars" {
            n933 = call "Queue Manager.vi"("queue in"=w1875, "Queue States In"=cluster{"Enum":T8, "Data":variant}[] [{"Enum"=enum."Undo Auto Update Pars", "Data"=variant}, {"Enum"=enum."Idle", "Data"=variant}]) -> ()  [unwired: 11 in, 3 out]
          }
          frame Default {
            n934 = One Button Dialog(message="Error - Undefined Menu Item") -> ()  [unwired: 1 in, 1 out]
          }
        }
      }
      event "Find Peaks": Value Change {
        n935 = event-data() -> ()  [unwired: 1 in, 5 out]
        n936 = call "Queue Manager.vi"("queue in"=w1878, "Queue States In"=cluster{"Enum":T8, "Data":variant}[] [{"Enum"=enum."Find Peaks", "Data"=variant}, {"Enum"=enum."Idle", "Data"=variant}]) -> ()  [unwired: 11 in, 3 out]
      }
      event "Lock Field", "Apply & Lock Center Field": Value Change {
        n937 = event-data() -> ()  [unwired: 1 in, 5 out]
        n938 = call "Queue Manager.vi"("queue in"=w1880, "Queue States In"=cluster{"Enum":T8, "Data":variant}[] [{"Enum"=enum."Lock Field", "Data"=variant}, {"Enum"=enum."Idle", "Data"=variant}]) -> ()  [unwired: 11 in, 3 out]
      }
      event "Scan?": Value Change {
        w1882 = FALSE ("Visible")
        n939 = event-data() -> ()  [unwired: 1 in, 5 out]
        n940 = property on="Flag Bad Set" class="Bool (strict)"("Visible"=w1882) -> ()  [unwired: 2 in, 2 out]
        n941 = property on="Scan?" class="Bool (strict)"("Visible"=w1882) -> ()  [unwired: 2 in, 2 out]
        n942 = property on="End Session?" class="Bool (strict)"("Visible"=w1882) -> ()  [unwired: 2 in, 2 out]
        n943 = call "Queue Manager.vi"("queue in"=w1884, "Queue States In"=cluster{"Enum":T8, "Data":variant}[] [{"Enum"=enum."Read GUI Pars", "Data"=variant}, {"Enum"=enum."Configure Hardware", "Data"=variant}, {"Enum"=enum."Initialize Set", "Data"=variant}, {"Enum"=enum."Pre-Scan", "Data"=variant}]) -> ()  [unwired: 11 in, 3 out]
      }
      event "Calibrate": Value Change {
        # "State values replicated in the 'Check Calibration' VI"
        n944 = event-data() -> ()  [unwired: 1 in, 5 out]
        n945 = call "Queue Manager.vi"("queue in"=w1886, "Queue States In"=cluster{"Enum":T8, "Data":variant}[] [{"Enum"=enum."Check Calibration", "Data"=variant}, {"Enum"=enum."Configure Hardware", "Data"=variant}, {"Enum"=enum."Initialize Set", "Data"=variant}, {"Enum"=enum."Pre-Scan", "Data"=variant}]) -> ()  [unwired: 11 in, 3 out]
        n946 = disable-structure shown="Disabled" {
          frame Disabled {
            n947 = call "Check Calibration.vi"() -> ()  [unwired: 8 in, 4 out]
          }
          frame Enabled {
          }
        }
      }
      event "Start Script": Value Change {
        n948 = event-data() -> ()  [unwired: 1 in, 5 out]
        n949 = call "Queue Manager.vi"("queue in"=w1887, "Queue States In"=cluster{"Enum":T8, "Data":variant}[] [{"Enum"=enum."Read GUI Pars", "Data"=variant}, {"Enum"=enum."Read from Script", "Data"=variant}]) -> ()  [unwired: 11 in, 3 out]
      }
      event "Frequency (Hz)", "Time constant", "Phase (deg)", "Mod. Amp. (Gauss)", "Sensitivity", "Offset comp.?", "AFC Control", "Electromagnet Main Field (Gauss)", "Attenuation/dB": Value Change {
        n950 = event-data() -> ()  [unwired: 1 in, 5 out]
        n951 = call "Queue Manager.vi"("queue in"=w1889, "Queue States In"=cluster{"Enum":T8, "Data":variant}[] [{"Enum"=enum."Read GUI Pars", "Data"=variant}, {"Enum"=enum."Configure Hardware", "Data"=variant}, {"Enum"=enum."Idle", "Data"=variant}]) -> ()  [unwired: 11 in, 3 out]
      }
      event "Optimize RF Power": Value Change {
        n952 = event-data() -> ()  [unwired: 1 in, 5 out]
        n953 = call "Queue Manager.vi"("queue in"=w1891, "Queue States In"=cluster{"Enum":T8, "Data":variant}[] [{"Enum"=enum."Optimize RF Power", "Data"=variant}]) -> ()  [unwired: 11 in, 3 out]
      }
      event "Magnet Angle (deg)": Value Change {
        n954 = event-data() -> ()  [unwired: 1 in, 5 out]
        n955 = call "Queue Manager.vi"("queue in"=w1893, "Queue States In"=cluster{"Enum":T8, "Data":variant}[] [{"Enum"=enum."Read GUI Pars", "Data"=variant}, {"Enum"=enum."Rotate Magnet", "Data"=variant}, {"Enum"=enum."Idle", "Data"=variant}]) -> ()  [unwired: 11 in, 3 out]
      }
      event "Get Q": Value Change {
        n956 = event-data() -> ()  [unwired: 1 in, 5 out]
        n957 = call "Queue Manager.vi"("queue in"=w1895, "Queue States In"=cluster{"Enum":T8, "Data":variant}[] [{"Enum"=enum."Measure Q", "Data"=variant}, {"Enum"=enum."Idle", "Data"=variant}]) -> ()  [unwired: 11 in, 3 out]
      }
      event "Zero All Voltage": Value Change {
        n958 = event-data() -> ()  [unwired: 1 in, 5 out]
        n959 = call "Queue Manager.vi"("queue in"=w1897, "Queue States In"=cluster{"Enum":T8, "Data":variant}[] [{"Enum"=enum."Zero Voltages", "Data"=variant}, {"Enum"=enum."Idle", "Data"=variant}]) -> ()  [unwired: 11 in, 3 out]
      }
      event "Set Phase", "Set Freq": Value Change {
        n960 = event-data() -> ()  [unwired: 1 in, 5 out]
        n961 = call "Queue Manager.vi"("queue in"=w1899, "Queue States In"=cluster{"Enum":T8, "Data":variant}[] [{"Enum"=enum."Engineering Tuning", "Data"=variant}, {"Enum"=enum."Idle", "Data"=variant}]) -> ()  [unwired: 11 in, 3 out]
      }
      event "Refit Spectra": Value Change {
        n962 = event-data() -> ()  [unwired: 1 in, 5 out]
        n963 = call "Queue Manager.vi"("queue in"=w1901, "Queue States In"=cluster{"Enum":T8, "Data":variant}[] [{"Enum"=enum."Read GUI Pars", "Data"=variant}, {"Enum"=enum."Refit Data", "Data"=variant}, {"Enum"=enum."Idle", "Data"=variant}]) -> ()  [unwired: 11 in, 3 out]
      }
      event "Measure Noise": Value Change {
        n964 = event-data() -> ()  [unwired: 1 in, 5 out]
        n965 = call "Queue Manager.vi"("queue in"=w1903, "Queue States In"=cluster{"Enum":T8, "Data":variant}[] [{"Enum"=enum."Measure Noise", "Data"=variant}, {"Enum"=enum."Idle", "Data"=variant}]) -> ()  [unwired: 11 in, 3 out]
      }
      event "Collect QA Scan": Value Change {
        n966 = event-data() -> ()  [unwired: 1 in, 5 out]
        n967 = call "Queue Manager.vi"("queue in"=w1905, "Queue States In"=cluster{"Enum":T8, "Data":variant}[] [{"Enum"=enum."Read GUI Pars", "Data"=variant}, {"Enum"=enum."Set Oxy QA-Scan Pars", "Data"=variant}, {"Enum"=enum."Configure Hardware", "Data"=variant}, {"Enum"=enum."Initialize Set", "Data"=variant}, {"Enum"=enum."Pre-Scan", "Data"=variant}]) -> ()  [unwired: 11 in, 3 out]
      }
      event "Single Test Scan": Value Change {
        n968 = event-data() -> ()  [unwired: 1 in, 6 out]
        n969 = call "Queue Manager.vi"("queue in"=w1907, "Queue States In"=cluster{"Enum":T8, "Data":variant}[] [{"Enum"=enum."Read GUI Pars", "Data"=variant}, {"Enum"=enum."Test Scan", "Data"=variant}, {"Enum"=enum."Configure Hardware", "Data"=variant}, {"Enum"=enum."Initialize Set", "Data"=variant}, {"Enum"=enum."Pre-Scan", "Data"=variant}]) -> ()  [unwired: 11 in, 3 out]
      }
      event "Open Session Data Folder": Value Change {
        n970 = event-data() -> ()  [unwired: 1 in, 5 out]
        n971 = call "Queue Manager.vi"("queue in"=w1909, "Queue States In"=cluster{"Enum":T8, "Data":variant}[] [{"Enum"=enum."Open Session Data Folder", "Data"=variant}, {"Enum"=enum."Idle", "Data"=variant}]) -> ()  [unwired: 11 in, 3 out]
      }
      event "Update Center Field": Value Change {
        n972 = event-data() -> ()  [unwired: 1 in, 5 out]
        n973 = call "Queue Manager.vi"("queue in"=w1911, "Queue States In"=cluster{"Enum":T8, "Data":variant}[] [{"Enum"=enum."Update Center Field", "Data"=variant}, {"Enum"=enum."Idle", "Data"=variant}]) -> ()  [unwired: 11 in, 3 out]
      }
      event "Mark Time of Transition": Value Change {
        n974 = event-data() -> ()  [unwired: 1 in, 5 out]
        n975 = call "Queue Manager.vi"("queue in"=w1913, "Queue States In"=cluster{"Enum":T8, "Data":variant}[] [{"Enum"=enum."Mark transition time", "Data"=variant}, {"Enum"=enum."Idle", "Data"=variant}]) -> ()  [unwired: 11 in, 3 out]
      }
      event "Flag Bad Set": Value Change {
        n976 = event-data() -> ()  [unwired: 1 in, 6 out]
        n977 = call "Queue Manager.vi"("queue in"=w1915, "Queue States In"=cluster{"Enum":T8, "Data":variant}[] [{"Enum"=enum."Flag Bad Set", "Data"=variant}, {"Enum"=enum."Idle", "Data"=variant}]) -> ()  [unwired: 11 in, 3 out]
      }
      event "Auto-Tune": Value Change {
        n978 = event-data() -> ()  [unwired: 1 in, 5 out]
        n979 = call "Queue Manager.vi"("queue in"=w1917, "Queue States In"=cluster{"Enum":T8, "Data":variant}[] [{"Enum"=enum."Automated Tuning", "Data"=variant}, {"Enum"=enum."Idle", "Data"=variant}]) -> ()  [unwired: 11 in, 3 out]
      }
      event "Manual Tuning": Value Change {
        n980 = event-data() -> ()  [unwired: 1 in, 5 out]
        n981 = call "Queue Manager.vi"("queue in"=w1919, "Queue States In"=cluster{"Enum":T8, "Data":variant}[] [{"Enum"=enum."Manual Tuning", "Data"=variant}, {"Enum"=enum."Idle", "Data"=variant}]) -> ()  [unwired: 11 in, 3 out]
      }
      event "New Session": Value Change {
        n982 = event-data() -> ()  [unwired: 1 in, 5 out]
        n983 = call "Queue Manager.vi"("queue in"=w1921, "Queue States In"=cluster{"Enum":T8, "Data":variant}[] [{"Enum"=enum."Read GUI Pars", "Data"=variant}, {"Enum"=enum."New Session", "Data"=variant}]) -> ()  [unwired: 11 in, 3 out]
      }
      event "End Session?": Value Change {
        n984 = event-data() -> ()  [unwired: 1 in, 5 out]
        n985 = global write "Global Variables.vi" "Abort QA"(FALSE ("Abort QA")) -> ()
        n986 = call "Queue Manager.vi"("queue in"=w1924, "Queue States In"=cluster{"Enum":T8, "Data":variant}[] [{"Enum"=enum."End Session", "Data"=variant}]) -> ()  [unwired: 11 in, 3 out]
      }
    }
    n987 = global read "Global Variables.vi" "Stop(QSM)"() -> (w1809:bool)
    n988 = Or(x=w1808, y=w1809) -> (x .or. y?=w1810:bool)
    "Producer Loop" <- w1811
  }
  n989 = Release Queue(queue=w12, error in (no error)=w10) -> (error out=w9:errorcluster)  [unwired: 1 in, 2 out]
  n990 = call <vilib>:"Clear Errors.vi"("error in (no error)"=w9) -> ()  [unwired: 5 in, 2 out]
